vi "Results_file_Plotter.vi"() -> ()   [LabVIEW 2015]
uses:
  Anemometry/Anemometry Sub Vis/Data_plotting_vis/Plot_Slice.ctl
  Anemometry/Anemometry Sub Vis/Data_plotting_vis/Plotter_Mode.ctl
  Anemometry/Anemometry Sub Vis/Data_plotting_vis/Data_File_Type.ctl
  Anemometry/Anemometry Sub Vis/File/Setup_Filetype.ctl
  Anemometry/Anemometry Sub Vis/Controls/Global_mode.ctl
  Anemometry/Anemometry Sub Vis/Data_plotting_vis/Results_plotter_Global.vi
  Instance           1 28Saved   Results_file_Plotter .vi
  Anemometry/Anemometry Sub Vis/Globals/Constants_global.vi
  Anemometry/Anemometry Sub Vis/Globals/Trav_pos_global.vi
  kernel32.dll
panel:
  out "Index when last displayed":i32
  out "Index when last plotted":i32
  out "Edit Raw DF?":bool
  in  "Tab Control":T1(tab)=enum."Save "
  in  "Template":path
  in  "Empty":bool
  in  "Result files to read":path[](array[path])
  in  "Add results file":bool
  in  "File Types to Read":T2
  in  "Dot Plot?":bool
  in  "Vector Plot?":bool
  in  "Ordinate Name":string
  out "2nd Add label":string
  out "First Add label":string
  in  "Additional X Values":dbl[](array[numeric]) format="%.2f"
  in  "Additional Y Values":dbl[](array[numeric]) format="%.2f"
  in  "Show Results Space Analysis":bool
  in  "Show Plot Space Analysis":bool
  in  "Multi Ordinate":i32[](listbox)
  in  "Multi Ordinate?":bool
  in  "Ordinate":u16(ring) items=["File", "Date", "Time", "Comments", "Chilled Water Temp", "Inlet_Temp Average", "Av Floor Temp", "Max deltaT", "X (mm)", "Y (mm)", "Z (mm)", "Z (m)", "U/Uref", "u^2/Uref^2", "w^2/Uref^2", "-uw/Uref^2", "Inlet DeltaT", "DeltaT", "t^2", "ut", "wt", "Grad Ri", "Flux Ri", "B-V Freq N", "DeltaT/DeltaTmax", "W/Uref", "T thermistor", "dT/dZ", "dU/dZ", "Inlet Delta_Set", "u'/U", "w'/U", "W/U", "Location XY", "Location XZ", "U m/s", "W m/s", "u^2", "w^2", "Speed/Uref", "T cw", "Uref", "Flow Meas Time", "Profile", "t'/T", "t'", "uw", "Spires", "Roughness", "Z=1450 Inlet Temp", "Z=1350 Inlet Temp", "Z=1250 Inlet Temp", "Z=1150 Inlet Temp", "Z=1050 Inlet Temp", "Z=950 Inlet Temp", "Z=850 Inlet Temp", "Z=750 Inlet Temp", "Z=650 Inlet Temp", "Z=550 Inlet Temp", "Z=450 Inlet Temp", "Z=350 Inlet Temp", "Z=250 Inlet Temp", "Z=150 Inlet Temp", "Z=50 Inlet Temp", "EnFlo Lab Hygrometry Dew Point temp", "EnFlo Lab Hygrometry Dew Point temp_PN", "Multi Run Start Time", "T cw Offset A", "T cw Grad B", "LDA (U) Standard Error in Variance", "LDA (U) Standard Error in Mean", "LDA (W) Standard Error in Mean", "LDA (W) Standard Error in Variance", "U/Uref Err", "u^2/Uref^2 Err", "W/Uref Err", "w^2/Uref^2 Err", "Inlet Temp", "Inlet Setpoint", "Inlet Temp Error", "Seconds since 1st Jan", "Uni Chilled Water Temp", "EnFlo_Tunnel Chilled Water Valve Dem Pos", "EnFlo_Tunnel Temp Floor_Up_Y=-1585", "EnFlo_Tunnel Temp Floor_Up_Y=-1250", "EnFlo_Tunnel Temp Floor_Up_Y=-920", "EnFlo_Tunnel Temp Floor_Up_Y=-585", "EnFlo_Tunnel Temp Floor_Up_Y=-250", "EnFlo_Tunnel Temp Floor_Up_Y=80", "EnFlo_Tunnel Temp Floor_Up_Y=415", "EnFlo_Tunnel Temp Floor_Up_Y=750", "EnFlo_Tunnel Temp Floor_Up_Y=1080", "EnFlo_Tunnel Temp Floor_Up_Y=1415", "Raw Data Filename", "Z=1450 Inlet Setpoint", "Z=1350 Inlet Setpoint", "Z=1250 Inlet Setpoint", "Z=1150 Inlet Setpoint", "Z=1050 Inlet Setpoint", "Z=950 Inlet Setpoint", "Z=850 Inlet Setpoint", "Z=750 Inlet Setpoint", "Z=650 Inlet Setpoint", "Z=550 Inlet Setpoint", "Z=450 Inlet Setpoint", "Z=350 Inlet Setpoint", "Z=250 Inlet Setpoint", "Z=150 Inlet Setpoint", "Z=50 Inlet Setpoint", "Freq Hz", "LDA (U) E(f)", "LDA (W) E(f)", "CW (T) f.E(f)", "LDA (U) f.E(f)", "LDA (W) f.E(f)", "Folder"]
  in  "Intensity Plot?":bool
  in  "Absisca":u16(ring) items=["File", "Date", "Time", "Comments", "Chilled Water Temp", "Inlet_Temp Average", "Av Floor Temp", "Max deltaT", "X (mm)", "Y (mm)", "Z (mm)", "Z (m)", "U/Uref", "u^2/Uref^2", "w^2/Uref^2", "-uw/Uref^2", "Inlet DeltaT", "DeltaT", "t^2", "ut", "wt", "Grad Ri", "Flux Ri", "B-V Freq N", "DeltaT/DeltaTmax", "W/Uref", "T thermistor", "dT/dZ", "dU/dZ", "Inlet Delta_Set", "u'/U", "w'/U", "W/U", "Location XY", "Location XZ", "U m/s", "W m/s", "u^2", "w^2", "Speed/Uref", "T cw", "Uref", "Flow Meas Time", "Profile", "t'/T", "t'", "uw", "Spires", "Roughness", "Z=1450 Inlet Temp", "Z=1350 Inlet Temp", "Z=1250 Inlet Temp", "Z=1150 Inlet Temp", "Z=1050 Inlet Temp", "Z=950 Inlet Temp", "Z=850 Inlet Temp", "Z=750 Inlet Temp", "Z=650 Inlet Temp", "Z=550 Inlet Temp", "Z=450 Inlet Temp", "Z=350 Inlet Temp", "Z=250 Inlet Temp", "Z=150 Inlet Temp", "Z=50 Inlet Temp", "EnFlo Lab Hygrometry Dew Point temp", "EnFlo Lab Hygrometry Dew Point temp_PN", "Multi Run Start Time", "T cw Offset A", "T cw Grad B", "LDA (U) Standard Error in Variance", "LDA (U) Standard Error in Mean", "LDA (W) Standard Error in Mean", "LDA (W) Standard Error in Variance", "U/Uref Err", "u^2/Uref^2 Err", "W/Uref Err", "w^2/Uref^2 Err", "Inlet Temp", "Inlet Setpoint", "Inlet Temp Error", "Seconds since 1st Jan", "Uni Chilled Water Temp", "EnFlo_Tunnel Chilled Water Valve Dem Pos", "EnFlo_Tunnel Temp Floor_Up_Y=-1585", "EnFlo_Tunnel Temp Floor_Up_Y=-1250", "EnFlo_Tunnel Temp Floor_Up_Y=-920", "EnFlo_Tunnel Temp Floor_Up_Y=-585", "EnFlo_Tunnel Temp Floor_Up_Y=-250", "EnFlo_Tunnel Temp Floor_Up_Y=80", "EnFlo_Tunnel Temp Floor_Up_Y=415", "EnFlo_Tunnel Temp Floor_Up_Y=750", "EnFlo_Tunnel Temp Floor_Up_Y=1080", "EnFlo_Tunnel Temp Floor_Up_Y=1415", "Raw Data Filename", "Z=1450 Inlet Setpoint", "Z=1350 Inlet Setpoint", "Z=1250 Inlet Setpoint", "Z=1150 Inlet Setpoint", "Z=1050 Inlet Setpoint", "Z=950 Inlet Setpoint", "Z=850 Inlet Setpoint", "Z=750 Inlet Setpoint", "Z=650 Inlet Setpoint", "Z=550 Inlet Setpoint", "Z=450 Inlet Setpoint", "Z=350 Inlet Setpoint", "Z=250 Inlet Setpoint", "Z=150 Inlet Setpoint", "Z=50 Inlet Setpoint", "Freq Hz", "LDA (U) E(f)", "LDA (W) E(f)", "CW (T) f.E(f)", "LDA (U) f.E(f)", "LDA (W) f.E(f)", "Folder"]
  in  "Job Directory":path
  in  "Save Averaged rows":bool
  in  "Save Surface Fit":bool
  in  "Output Filename":path
  in  "Save Data in Rows":bool
  in  "Save Plot data":bool
  in  "Header":string
  in  "Process Point":bool
  in  "Kill Point":bool
  out "Table":string[][](table)
  in  "Post Process Plotted Data":bool
  in  "...using routine":string
  in  "Calculate new metadata":bool
  in  "Add /Edit metadata":bool
  in  "Delete Plotted data from file":bool
  in  "Add Inlet Temperature offset":bool
  in  "Plot EnFlo Tunnel Display":bool
  in  "Save Setup":bool
  in  "Load Setup":bool
  in  "stop":bool
  out "Current":string="Graph Scales"
  in  "Single Series":i32[](listbox)=[0]
  in  "Edit Template File":bool
  in  "color and symbol":bool
  out "nRows":i32
  in  "Filter Bins 2":i32[](listbox)=[0]
  in  "Filter 6":u16(ring)
  in  "Filter 5":u16(ring)
  in  "Filter 4":u16(ring)
  in  "Filter 3":u16(ring) items=["Show All (135)", "Vertical Profile (135)", "NOT Vertical Profile (0)"]
  in  "Filter Array":u16[](array[ring])=[0, 0, 0, 0, 0, 0] items=["Don't Filter", "File", "Date", "Time", "Comments", "Chilled Water Temp", "Inlet_Temp Average", "Av Floor Temp", "Max deltaT", "X (mm)", "Y (mm)", "Z (mm)", "Z (m)", "U/Uref", "u^2/Uref^2", "w^2/Uref^2", "-uw/Uref^2", "Inlet DeltaT", "DeltaT", "t^2", "ut", "wt", "Grad Ri", "Flux Ri", "B-V Freq N", "DeltaT/DeltaTmax", "W/Uref", "T thermistor", "dT/dZ", "dU/dZ", "Inlet Delta_Set", "u'/U", "w'/U", "W/U", "Location XY", "Location XZ", "U m/s", "W m/s", "u^2", "w^2", "Speed/Uref", "T cw", "Uref", "Flow Meas Time", "Profile", "t'/T", "t'", "uw", "Spires", "Roughness", "Z=1450 Inlet Temp", "Z=1350 Inlet Temp", "Z=1250 Inlet Temp", "Z=1150 Inlet Temp", "Z=1050 Inlet Temp", "Z=950 Inlet Temp", "Z=850 Inlet Temp", "Z=750 Inlet Temp", "Z=650 Inlet Temp", "Z=550 Inlet Temp", "Z=450 Inlet Temp", "Z=350 Inlet Temp", "Z=250 Inlet Temp", "Z=150 Inlet Temp", "Z=50 Inlet Temp", "EnFlo Lab Hygrometry Dew Point temp", "EnFlo Lab Hygrometry Dew Point temp_PN", "Multi Run Start Time", "T cw Offset A", "T cw Grad B", "LDA (U) Standard Error in Variance", "LDA (U) Standard Error in Mean", "LDA (W) Standard Error in Mean", "LDA (W) Standard Error in Variance", "U/Uref Err", "u^2/Uref^2 Err", "W/Uref Err", "w^2/Uref^2 Err", "Inlet Temp", "Inlet Setpoint", "Inlet Temp Error", "Seconds since 1st Jan", "Uni Chilled Water Temp", "EnFlo_Tunnel Chilled Water Valve Dem Pos", "EnFlo_Tunnel Temp Floor_Up_Y=-1585", "EnFlo_Tunnel Temp Floor_Up_Y=-1250", "EnFlo_Tunnel Temp Floor_Up_Y=-920", "EnFlo_Tunnel Temp Floor_Up_Y=-585", "EnFlo_Tunnel Temp Floor_Up_Y=-250", "EnFlo_Tunnel Temp Floor_Up_Y=80", "EnFlo_Tunnel Temp Floor_Up_Y=415", "EnFlo_Tunnel Temp Floor_Up_Y=750", "EnFlo_Tunnel Temp Floor_Up_Y=1080", "EnFlo_Tunnel Temp Floor_Up_Y=1415", "Raw Data Filename", "Z=1450 Inlet Setpoint", "Z=1350 Inlet Setpoint", "Z=1250 Inlet Setpoint", "Z=1150 Inlet Setpoint", "Z=1050 Inlet Setpoint", "Z=950 Inlet Setpoint", "Z=850 Inlet Setpoint", "Z=750 Inlet Setpoint", "Z=650 Inlet Setpoint", "Z=550 Inlet Setpoint", "Z=450 Inlet Setpoint", "Z=350 Inlet Setpoint", "Z=250 Inlet Setpoint", "Z=150 Inlet Setpoint", "Z=50 Inlet Setpoint", "Freq Hz", "LDA (U) E(f)", "LDA (W) E(f)", "CW (T) f.E(f)", "LDA (U) f.E(f)", "LDA (W) f.E(f)", "Folder"]
  in  "Filter Bins 1":i32[](listbox)=[0]
  in  "Create picture Vi Name":string caption="Picture VI:"
  in  "Save Plot as jpg":bool
  in  "Reload Files":bool
  out "Selected Row":i32
  out "Selected Row?":bool
  out "Warning!":string
  out "XY Plot":cluster{dbl[], dbl[]}[](graph)
  out "Edit Raw Data Header Info":bool
  out "Raw DF in Orig Pos?":bool
  out "Intensity Graph":dbl[][](graph)
  in  "Bkgnd Value":dbl
  in  "Update":bool
  in  "Plot Resolution":bool
  in  "Point Size":i32(slide)=1 scale=0.0..10.0
  in  "No of Contours":i32=20
  in  "Slice mode":T3
  in  "Z Ch Name":u16(ring) items=["File", "Date", "Time", "Comments", "Chilled Water Temp", "Inlet_Temp Average", "Av Floor Temp", "Max deltaT", "X (mm)", "Y (mm)", "Z (mm)", "Z (m)", "U/Uref", "u^2/Uref^2", "w^2/Uref^2", "-uw/Uref^2", "Inlet DeltaT", "DeltaT", "t^2", "ut", "wt", "Grad Ri", "Flux Ri", "B-V Freq N", "DeltaT/DeltaTmax", "W/Uref", "T thermistor", "dT/dZ", "dU/dZ", "Inlet Delta_Set", "u'/U", "w'/U", "W/U", "Location XY", "Location XZ", "U m/s", "W m/s", "u^2", "w^2", "Speed/Uref", "T cw", "Uref", "Flow Meas Time", "Profile", "t'/T", "t'", "uw", "Spires", "Roughness", "Z=1450 Inlet Temp", "Z=1350 Inlet Temp", "Z=1250 Inlet Temp", "Z=1150 Inlet Temp", "Z=1050 Inlet Temp", "Z=950 Inlet Temp", "Z=850 Inlet Temp", "Z=750 Inlet Temp", "Z=650 Inlet Temp", "Z=550 Inlet Temp", "Z=450 Inlet Temp", "Z=350 Inlet Temp", "Z=250 Inlet Temp", "Z=150 Inlet Temp", "Z=50 Inlet Temp", "EnFlo Lab Hygrometry Dew Point temp", "EnFlo Lab Hygrometry Dew Point temp_PN", "Multi Run Start Time", "T cw Offset A", "T cw Grad B", "LDA (U) Standard Error in Variance", "LDA (U) Standard Error in Mean", "LDA (W) Standard Error in Mean", "LDA (W) Standard Error in Variance", "U/Uref Err", "u^2/Uref^2 Err", "W/Uref Err", "w^2/Uref^2 Err", "Inlet Temp", "Inlet Setpoint", "Inlet Temp Error", "Seconds since 1st Jan", "Uni Chilled Water Temp", "EnFlo_Tunnel Chilled Water Valve Dem Pos", "EnFlo_Tunnel Temp Floor_Up_Y=-1585", "EnFlo_Tunnel Temp Floor_Up_Y=-1250", "EnFlo_Tunnel Temp Floor_Up_Y=-920", "EnFlo_Tunnel Temp Floor_Up_Y=-585", "EnFlo_Tunnel Temp Floor_Up_Y=-250", "EnFlo_Tunnel Temp Floor_Up_Y=80", "EnFlo_Tunnel Temp Floor_Up_Y=415", "EnFlo_Tunnel Temp Floor_Up_Y=750", "EnFlo_Tunnel Temp Floor_Up_Y=1080", "EnFlo_Tunnel Temp Floor_Up_Y=1415", "Raw Data Filename", "Z=1450 Inlet Setpoint", "Z=1350 Inlet Setpoint", "Z=1250 Inlet Setpoint", "Z=1150 Inlet Setpoint", "Z=1050 Inlet Setpoint", "Z=950 Inlet Setpoint", "Z=850 Inlet Setpoint", "Z=750 Inlet Setpoint", "Z=650 Inlet Setpoint", "Z=550 Inlet Setpoint", "Z=450 Inlet Setpoint", "Z=350 Inlet Setpoint", "Z=250 Inlet Setpoint", "Z=150 Inlet Setpoint", "Z=50 Inlet Setpoint", "Freq Hz", "LDA (U) E(f)", "LDA (W) E(f)", "CW (T) f.E(f)", "LDA (U) f.E(f)", "LDA (W) f.E(f)", "Folder"]
  in  "Y Ch Name":u16(ring) items=["File", "Date", "Time", "Comments", "Chilled Water Temp", "Inlet_Temp Average", "Av Floor Temp", "Max deltaT", "X (mm)", "Y (mm)", "Z (mm)", "Z (m)", "U/Uref", "u^2/Uref^2", "w^2/Uref^2", "-uw/Uref^2", "Inlet DeltaT", "DeltaT", "t^2", "ut", "wt", "Grad Ri", "Flux Ri", "B-V Freq N", "DeltaT/DeltaTmax", "W/Uref", "T thermistor", "dT/dZ", "dU/dZ", "Inlet Delta_Set", "u'/U", "w'/U", "W/U", "Location XY", "Location XZ", "U m/s", "W m/s", "u^2", "w^2", "Speed/Uref", "T cw", "Uref", "Flow Meas Time", "Profile", "t'/T", "t'", "uw", "Spires", "Roughness", "Z=1450 Inlet Temp", "Z=1350 Inlet Temp", "Z=1250 Inlet Temp", "Z=1150 Inlet Temp", "Z=1050 Inlet Temp", "Z=950 Inlet Temp", "Z=850 Inlet Temp", "Z=750 Inlet Temp", "Z=650 Inlet Temp", "Z=550 Inlet Temp", "Z=450 Inlet Temp", "Z=350 Inlet Temp", "Z=250 Inlet Temp", "Z=150 Inlet Temp", "Z=50 Inlet Temp", "EnFlo Lab Hygrometry Dew Point temp", "EnFlo Lab Hygrometry Dew Point temp_PN", "Multi Run Start Time", "T cw Offset A", "T cw Grad B", "LDA (U) Standard Error in Variance", "LDA (U) Standard Error in Mean", "LDA (W) Standard Error in Mean", "LDA (W) Standard Error in Variance", "U/Uref Err", "u^2/Uref^2 Err", "W/Uref Err", "w^2/Uref^2 Err", "Inlet Temp", "Inlet Setpoint", "Inlet Temp Error", "Seconds since 1st Jan", "Uni Chilled Water Temp", "EnFlo_Tunnel Chilled Water Valve Dem Pos", "EnFlo_Tunnel Temp Floor_Up_Y=-1585", "EnFlo_Tunnel Temp Floor_Up_Y=-1250", "EnFlo_Tunnel Temp Floor_Up_Y=-920", "EnFlo_Tunnel Temp Floor_Up_Y=-585", "EnFlo_Tunnel Temp Floor_Up_Y=-250", "EnFlo_Tunnel Temp Floor_Up_Y=80", "EnFlo_Tunnel Temp Floor_Up_Y=415", "EnFlo_Tunnel Temp Floor_Up_Y=750", "EnFlo_Tunnel Temp Floor_Up_Y=1080", "EnFlo_Tunnel Temp Floor_Up_Y=1415", "Raw Data Filename", "Z=1450 Inlet Setpoint", "Z=1350 Inlet Setpoint", "Z=1250 Inlet Setpoint", "Z=1150 Inlet Setpoint", "Z=1050 Inlet Setpoint", "Z=950 Inlet Setpoint", "Z=850 Inlet Setpoint", "Z=750 Inlet Setpoint", "Z=650 Inlet Setpoint", "Z=550 Inlet Setpoint", "Z=450 Inlet Setpoint", "Z=350 Inlet Setpoint", "Z=250 Inlet Setpoint", "Z=150 Inlet Setpoint", "Z=50 Inlet Setpoint", "Freq Hz", "LDA (U) E(f)", "LDA (W) E(f)", "CW (T) f.E(f)", "LDA (U) f.E(f)", "LDA (W) f.E(f)", "Folder"]
  in  "X Ch Name":u16(ring) items=["File", "Date", "Time", "Comments", "Chilled Water Temp", "Inlet_Temp Average", "Av Floor Temp", "Max deltaT", "X (mm)", "Y (mm)", "Z (mm)", "Z (m)", "U/Uref", "u^2/Uref^2", "w^2/Uref^2", "-uw/Uref^2", "Inlet DeltaT", "DeltaT", "t^2", "ut", "wt", "Grad Ri", "Flux Ri", "B-V Freq N", "DeltaT/DeltaTmax", "W/Uref", "T thermistor", "dT/dZ", "dU/dZ", "Inlet Delta_Set", "u'/U", "w'/U", "W/U", "Location XY", "Location XZ", "U m/s", "W m/s", "u^2", "w^2", "Speed/Uref", "T cw", "Uref", "Flow Meas Time", "Profile", "t'/T", "t'", "uw", "Spires", "Roughness", "Z=1450 Inlet Temp", "Z=1350 Inlet Temp", "Z=1250 Inlet Temp", "Z=1150 Inlet Temp", "Z=1050 Inlet Temp", "Z=950 Inlet Temp", "Z=850 Inlet Temp", "Z=750 Inlet Temp", "Z=650 Inlet Temp", "Z=550 Inlet Temp", "Z=450 Inlet Temp", "Z=350 Inlet Temp", "Z=250 Inlet Temp", "Z=150 Inlet Temp", "Z=50 Inlet Temp", "EnFlo Lab Hygrometry Dew Point temp", "EnFlo Lab Hygrometry Dew Point temp_PN", "Multi Run Start Time", "T cw Offset A", "T cw Grad B", "LDA (U) Standard Error in Variance", "LDA (U) Standard Error in Mean", "LDA (W) Standard Error in Mean", "LDA (W) Standard Error in Variance", "U/Uref Err", "u^2/Uref^2 Err", "W/Uref Err", "w^2/Uref^2 Err", "Inlet Temp", "Inlet Setpoint", "Inlet Temp Error", "Seconds since 1st Jan", "Uni Chilled Water Temp", "EnFlo_Tunnel Chilled Water Valve Dem Pos", "EnFlo_Tunnel Temp Floor_Up_Y=-1585", "EnFlo_Tunnel Temp Floor_Up_Y=-1250", "EnFlo_Tunnel Temp Floor_Up_Y=-920", "EnFlo_Tunnel Temp Floor_Up_Y=-585", "EnFlo_Tunnel Temp Floor_Up_Y=-250", "EnFlo_Tunnel Temp Floor_Up_Y=80", "EnFlo_Tunnel Temp Floor_Up_Y=415", "EnFlo_Tunnel Temp Floor_Up_Y=750", "EnFlo_Tunnel Temp Floor_Up_Y=1080", "EnFlo_Tunnel Temp Floor_Up_Y=1415", "Raw Data Filename", "Z=1450 Inlet Setpoint", "Z=1350 Inlet Setpoint", "Z=1250 Inlet Setpoint", "Z=1150 Inlet Setpoint", "Z=1050 Inlet Setpoint", "Z=950 Inlet Setpoint", "Z=850 Inlet Setpoint", "Z=750 Inlet Setpoint", "Z=650 Inlet Setpoint", "Z=550 Inlet Setpoint", "Z=450 Inlet Setpoint", "Z=350 Inlet Setpoint", "Z=250 Inlet Setpoint", "Z=150 Inlet Setpoint", "Z=50 Inlet Setpoint", "Freq Hz", "LDA (U) E(f)", "LDA (W) E(f)", "CW (T) f.E(f)", "LDA (U) f.E(f)", "LDA (W) f.E(f)", "Folder"]
  in  "Resolution":dbl=1.0 min=0.0 format="%.4f"
  out "Surface Area":dbl format="%^_6g"
  out "Surface Integral":dbl format="%^_6g"
  out "Surface Average":dbl format="%^#.6g"
  out "Uadvec":dbl
  in  "Full_Res_Results_Folder":path
  out "Last used Template":path
  out "Cursor index":i32
  out "Choosen Path":path
  in  "VI Refnum Calculation":refnum<vi>
  out "Filetype":string[](array[string])
  out "Mode":T4
  out "Plotted rows only?":bool
  in  "type specifier VI Refnum (for type only) 2":refnum<vi>
  in  "type specifier VI Refnum (for type only)":refnum<vi>
  out "Accept Array":bool[][](array[boolean])
  out "Previous slice mode":T3
  out "Slice mode Change?":bool
  out "Non-Blank Rows":bool[](array[boolean])
  out "File Index":i32
  out "Tolerances":dbl[](array[numeric]) format="%.2f"
  in  "Results files choosen":path[](array[path])
  in  "Transpose":bool
  out "Plotted Series":bool[][](array[boolean])
  in  "Results file":path
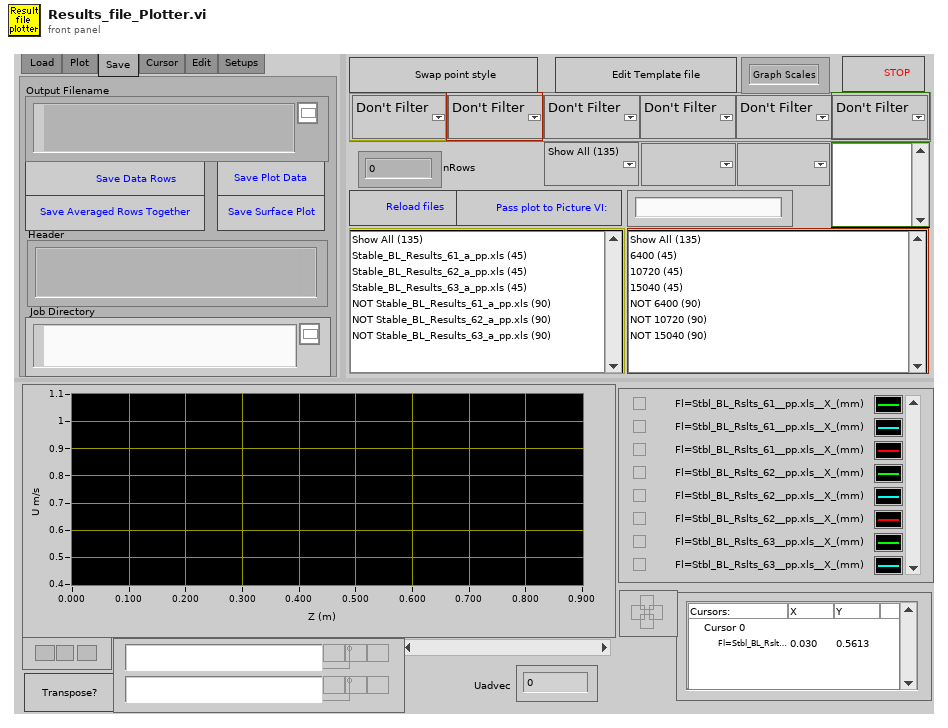
[diagram p1: front panel]
types:
  T1 = enum32{"Load ", "Plot ", "Save ", "Cursor", "Edit", "Setups"}
  T2 = typedef "Data_File_Type.ctl" = enum16{"Read All File Types", "Results Files Only", "Raw Data Files Only", "Calibration Files Only", "Gas Desk Files Only", "Old Results Files Only", "Tabulated Data Files Only"}
  T3 = typedef "Plot_Slice.ctl" = enum16{"XY Slice (Plan)", "YX Slice (Plan)", "YZ Slice (Cross)", "ZY Slice (Cross)", "XZ Slice (Side)", "ZX Slice (Side)"}
  T4 = typedef "Plotter_Mode.ctl" = enum16{"Save file", "Delete unwanted rows", "Edit Values with constants", "Edit values per row", "Edit Raw Data file header", "Post Process Plotted Rows", "Plot EnFlo Tunnel Display", "Add Inlet Temperature Offset"}
  T5 = typedef "Setup_Filetype.ctl" = enum16{"Measurement Setups", "Calibration Setups", "General", "Results File Plotter Setups", "Speed Calib Tweaks"}
  T6 = enum16{"Zero or one", "One", "Zero or more", "One or more"}
  T7 = typedef "Global_mode.ctl" = enum16{"Read Global", "Load Global From File", "Write Global to File"}
  T8 = enum16{"Edit Existing Template File", "Create New Template File"}
  T9 = enum16{"Show only data summary", "Show data summary", "No data summary"}
  T10 = typedef "All_Setup.ctl" = cluster{"Result files to read":path[], "Template":path, "Transpose":bool, "Additional X Values":dbl[], "Additional Y Values":dbl[], "Ordinate":u16, "Absisca":u16, "Filter Array":u16[], "color and symbol":bool, "Output Filename":path, "Jpg Vi Name":string, "Intensity Plot?":bool, "Multi Ordinate?":bool, "Filter Bins 1":i32[], "Filter Bins 2":i32[], "Multi Ordinate":i32[]}
  T11 = enum16{"Left Button", "Center Button", "Right Button", "Window Close"}
  T12 = enum32{"existing file", "new file", "new or existing file", "existing dir", "new dir", "new or existing dir", "existing file (use LLBs)", "new file (use LLBs)", "new or existing file (use LLBs)", "new or existing file or directory (use LLBs)"}
  T13 = cluster{"Plot Color":u32, "Plot Interpolation":u8, "Point Style":u8, "Line Style":u8, "Fill/Pt. Color":u32, "Line Width":u8, "Bar Plot Style":u8, "Fill To":i16}[]
  T14 = cluster{"X Max":dbl, "Y Max ":dbl, "X Scale":cluster{"Xo":dbl, "delta X":dbl}, "Y Scale":cluster{"Xo":dbl, "delta X":dbl}, "X Values":dbl[], "Y Values":dbl[], "Z Max":dbl, "Z Min":dbl}
  T15 = typedef "Group_Binning.ctl" = cluster{"Index":i32, "Tolerance":dbl, "Precision":string}
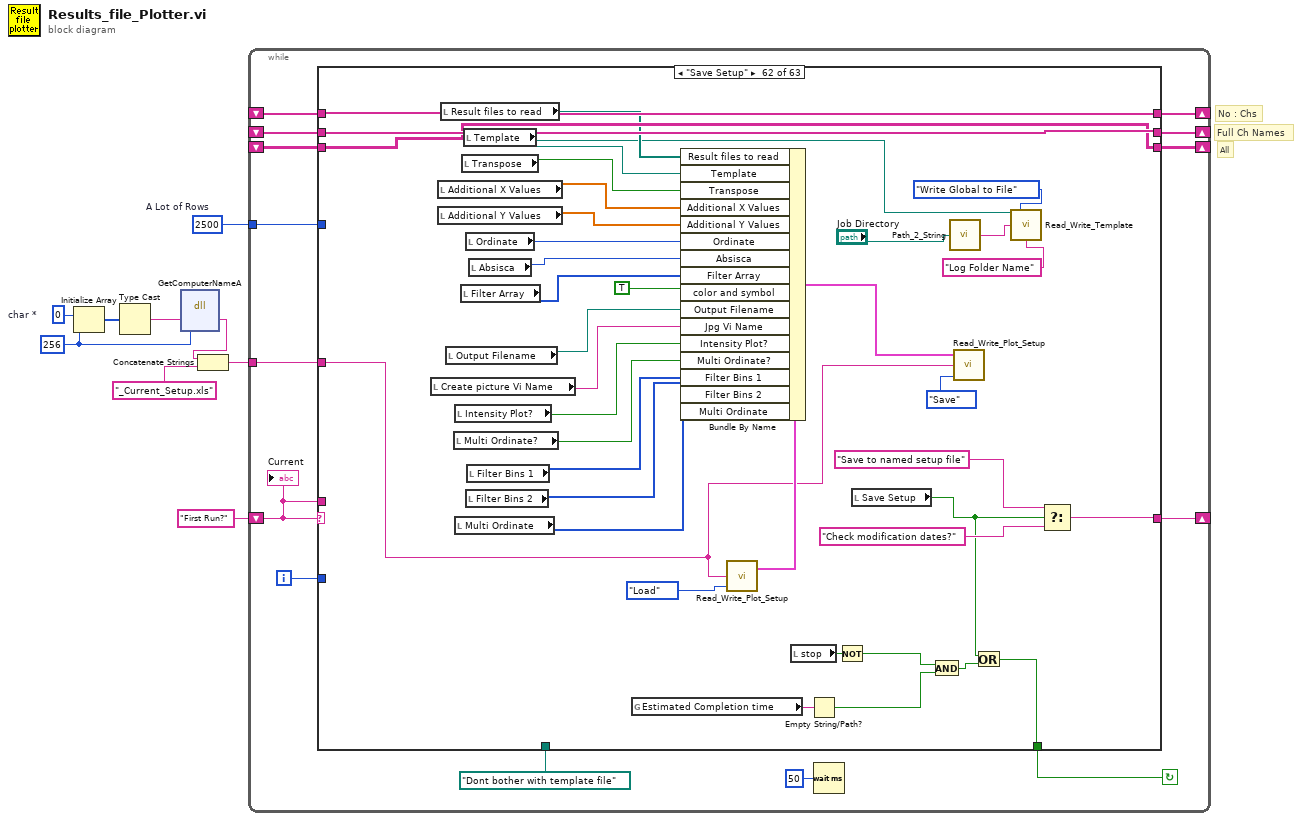
[diagram p0: block diagram]
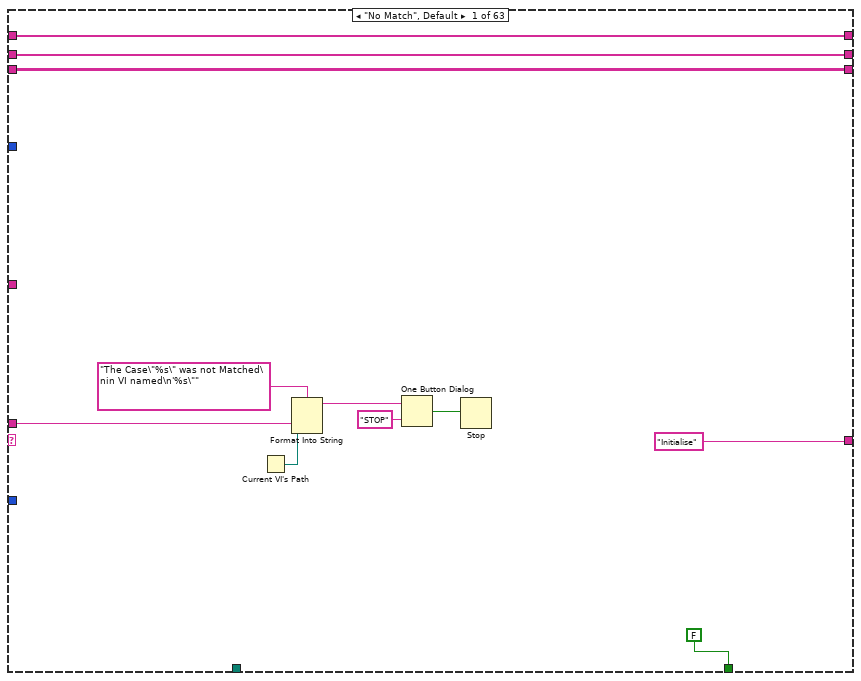
[diagram p2: hidden frame]
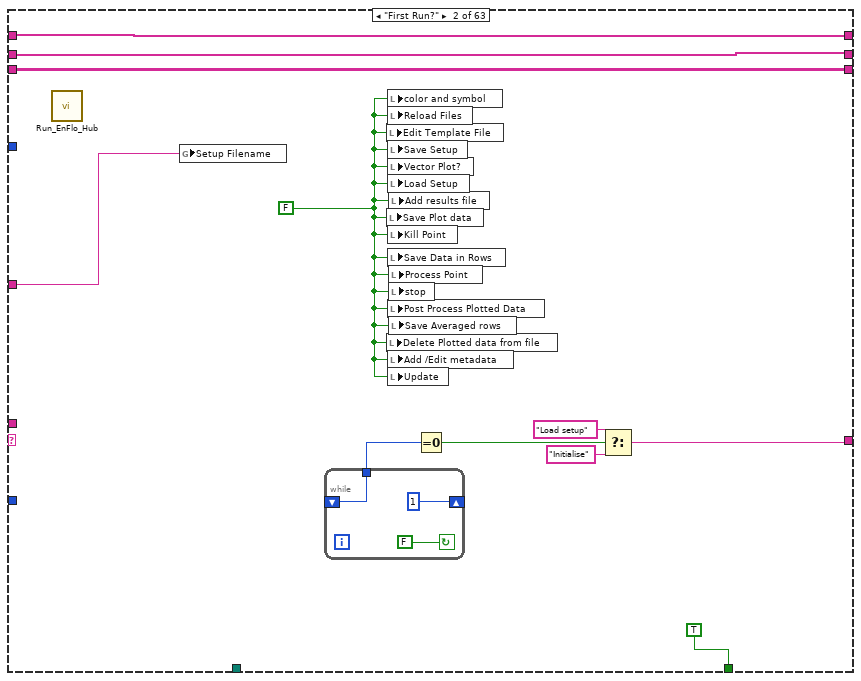
[diagram p3: hidden frame]
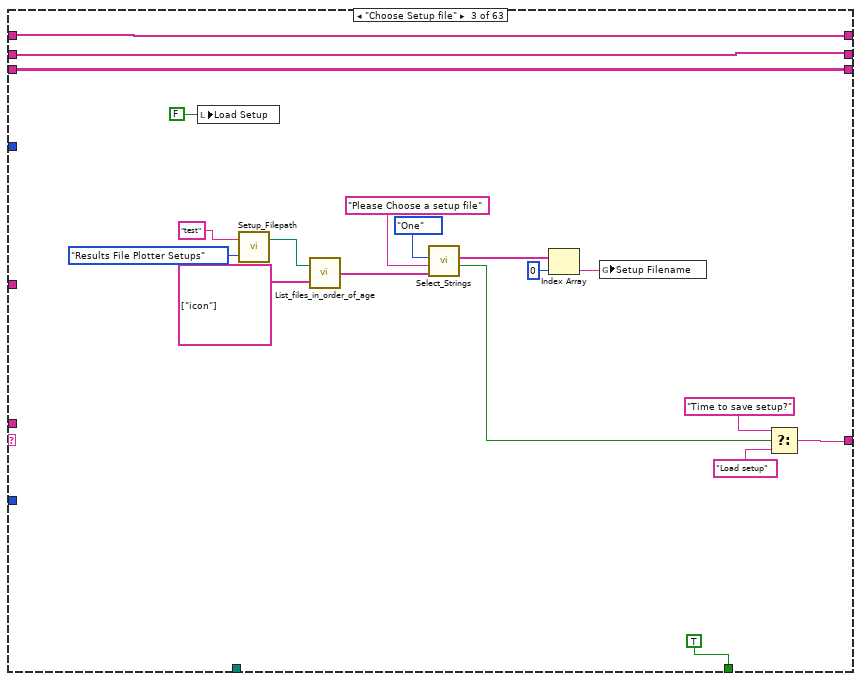
[diagram p4: hidden frame]
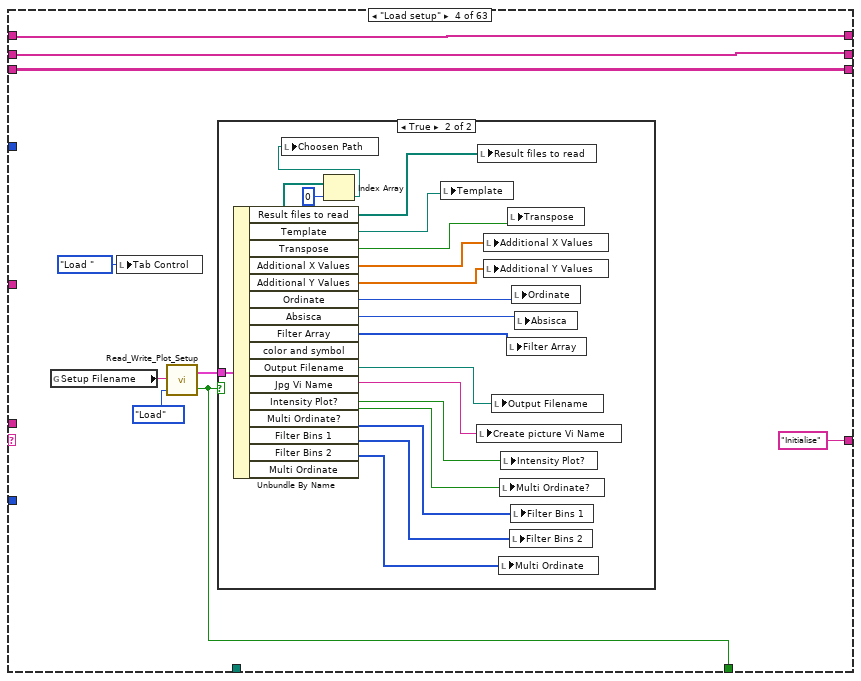
[diagram p5: hidden frame]
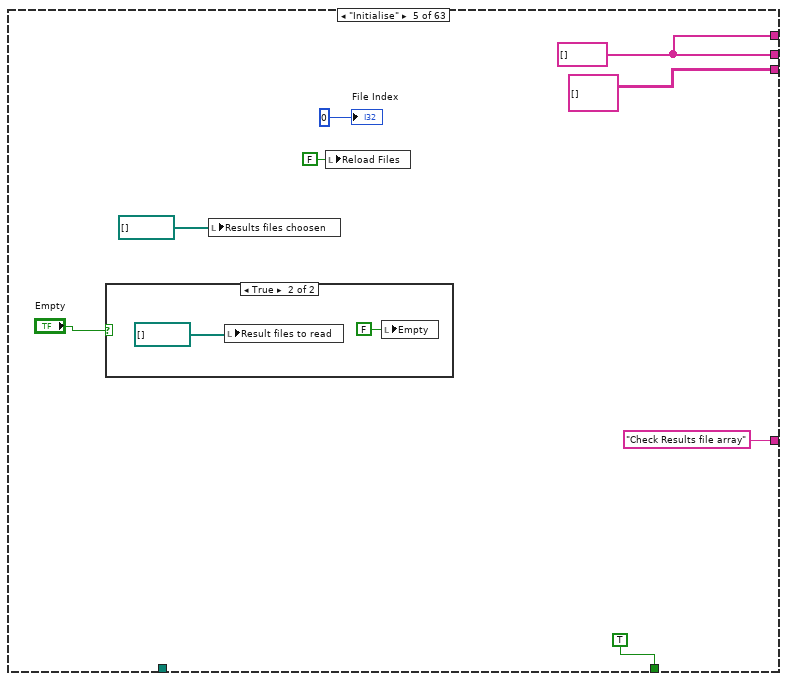
[diagram p7: hidden frame]
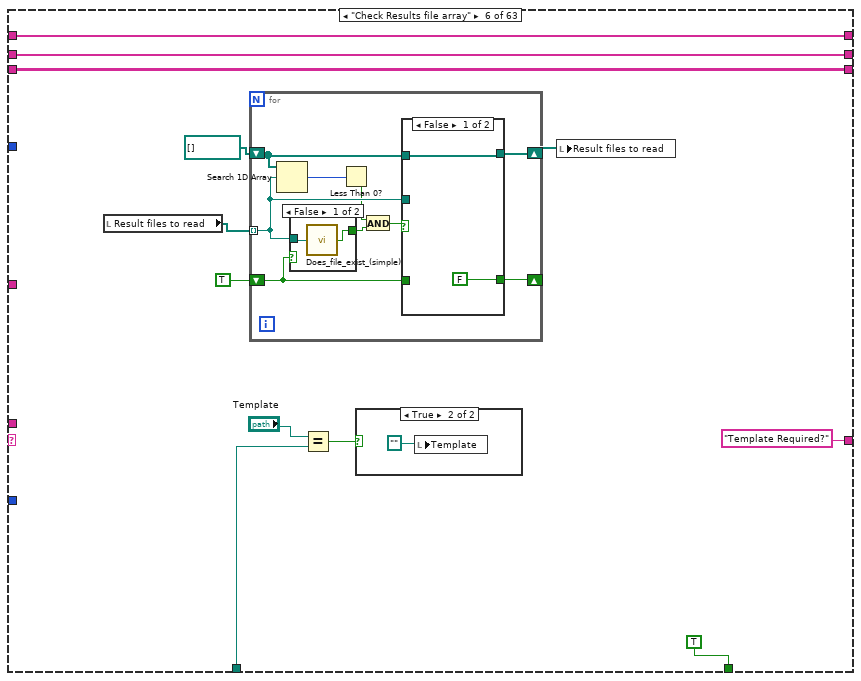
[diagram p9: hidden frame]
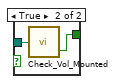
[diagram p11: hidden frame]
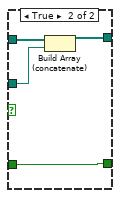
[diagram p12: hidden frame]
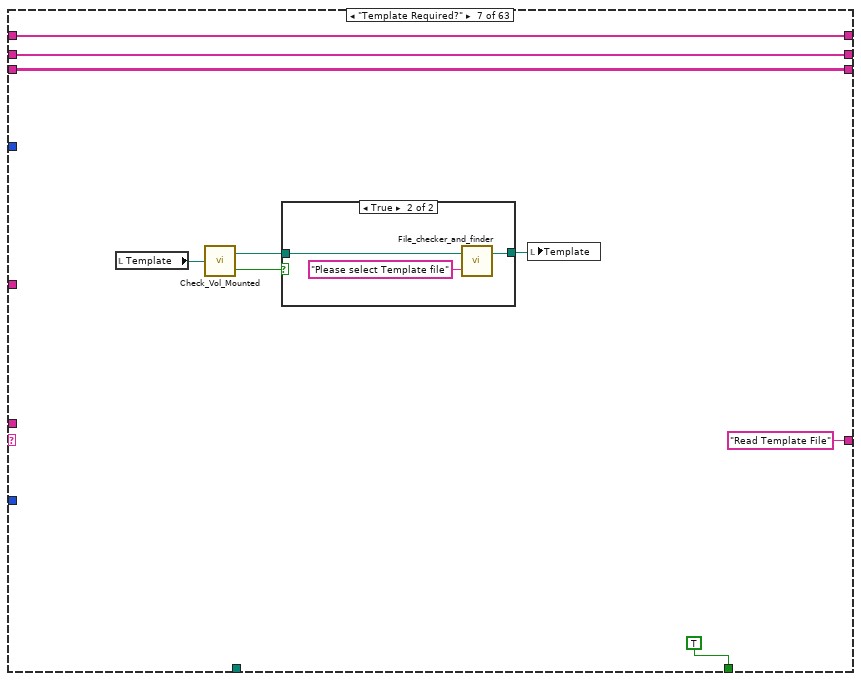
[diagram p13: hidden frame]
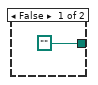
[diagram p14: hidden frame]
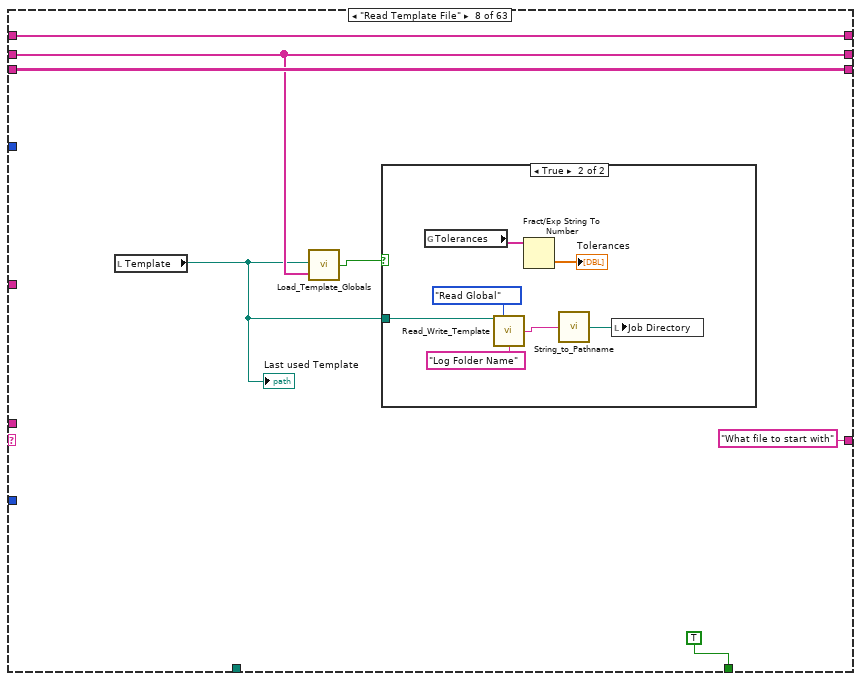
[diagram p15: hidden frame]
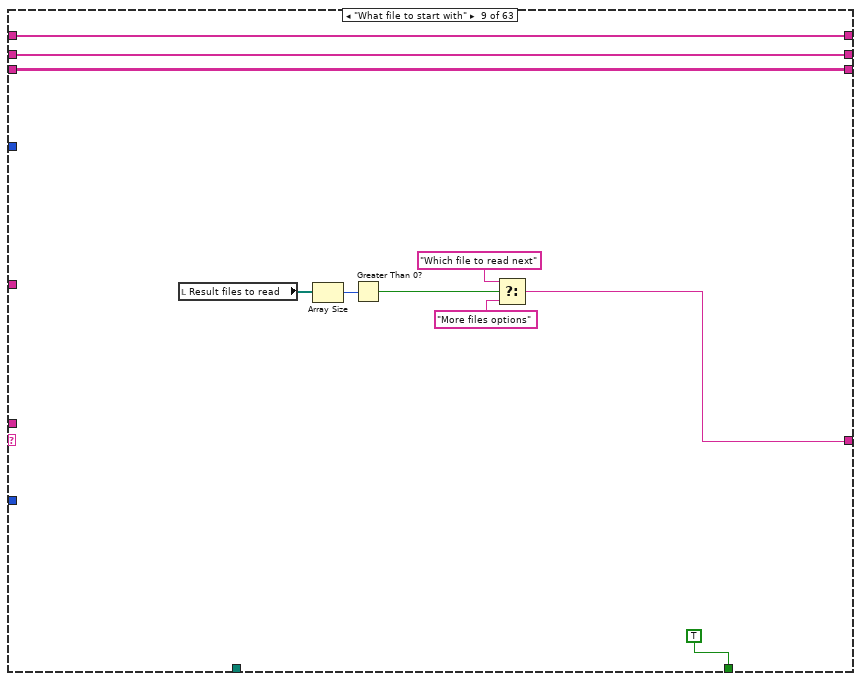
[diagram p17: hidden frame]
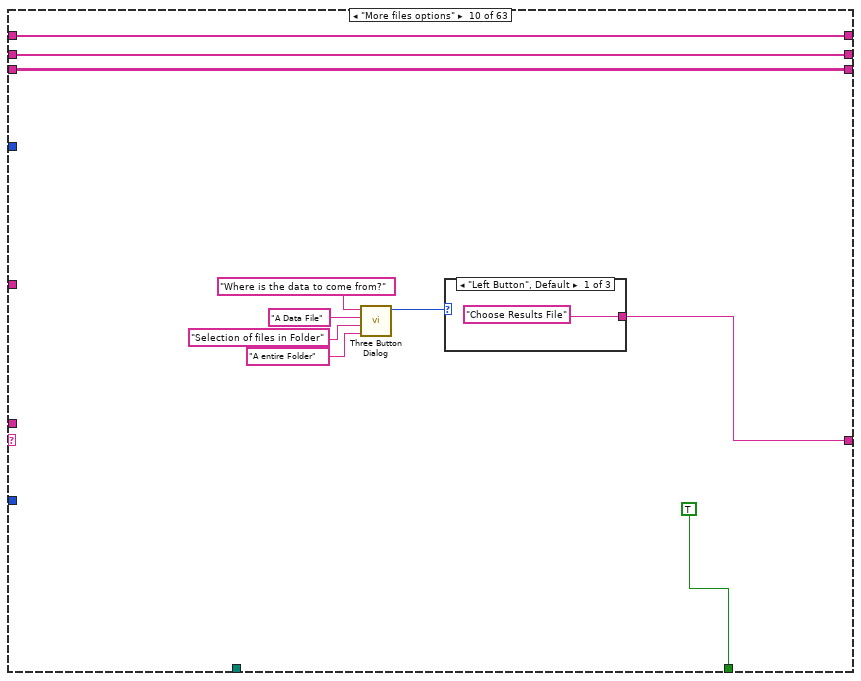
[diagram p18: hidden frame]
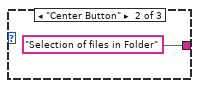
[diagram p19: hidden frame]
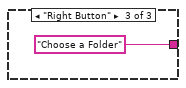
[diagram p20: hidden frame]
diagram:
  w7 = 256 ("dimension size")
  w4 = u8 0  # char *
  w8 = 2500  # A Lot of Rows
  # "No : Chs"
  # "Full Ch Names"
  # "All"
  n1 = Initialize Array(w4, w7) -> (w5:u8[])
  n2 = Type Cast(x=w5) -> (*(type *) &x=w6:string)  [unwired: 1 in]
  n3 = dll-call lib="kernel32.dll" fn="GetComputerNameA" label="unsigned long GetComputerNameA(CStr lpBuffer, long *nSize);"("lpBuffer"=w6, "nSize"=w7) -> ("lpBuffer"=w2:string)  [unwired: 5 in, 2 out]
  n4 = Concatenate Strings(w2, "_Current_Setup.xls" ("Setup filename")) -> (w1:string)
  n5 = while {
    shift-left: _ -> [w16]
    shift-right: [w17] -> _
    shift-left: "First Run?" -> [w20]
    shift-right: [w13] -> _
    shift-left: _ -> [w18]
    shift-right: [w23] -> _
    shift-left: _ -> [w21]
    shift-right: [w14] -> _
    tunnel: w8 -> [w12]
    tunnel: w1 -> [w10]
    i -> [w15]
    stop <- w22 continue-if-true
    n6 = case shown="\"Save Setup\"" w20 {
      tunnel: w18 -> [w34 w44 w66 w74 _ w115 w143 w152 w173 w183 w195 w209 w240 w267 w290 w412 w434 w460 w485 w511 w565 w579 w616 w926 w997 w1052 w1077 w1097 w1185 w1239 w1269 w1569 w1585 w1597 w1629 w1659 w1731 w1769 w1779 w1848 w1871 w1886 w1950 w2004 w2030 w2239 w2251 w2279 w2423 w2567 w2601 w2616 w2641 w2668 w2711 w2729 w2772 w2875 w2909 w3318 w3333 w3373 w3381]
      tunnel: [w34 w44 w66 w74 w100 w115 w143 w152 w173 w183 w195 w209 w240 w267 w288 w412 w434 w460 w485 w511 w565 w579 w616 w926 w997 w1052 w1077 w1097 w1185 w1239 w1267 w1569 w1585 w1597 w1629 w1659 w1731 w1769 w1779 w1848 w1871 w1886 w1950 w2004 w2028 w2239 w2251 w2277 w2416 w2567 w2601 w2616 w2641 w2668 w2711 w2729 w2772 w2875 w2909 w3318 w3333 w3373 w3381] -> w23
      tunnel: ["Initialise" w37 w61 "Initialise" ("t") "Check Results file array" ("t") "Template Required?" "Read Template File" "What file to start with" w164 w179 "Which file to read next" "Which file to read next" "Which file to read next" w263 w285 w403 "What is present?" "Ordinate Selector Type" w482 "Which rows are Non-Blank?" w558 "Create Selectors" w605 "Re Plot Data?" w993 "Prepare Filter2 strings" "Plot Data" w1094 "Add Axis names" "Analyse Plot Space" w1270 "What to do next?" "What to do next?" ("t") "What to do next?" ("t") w1611 w1652 w1707 w1765 w1777 w1843 w1867 w1885 w1949 "Initialise" w2031 w2230 "Create Selectors" w2280 w2424 w2565 w2599 w2606 w2625 "Save XY plot as jpg" "Create Selectors" w2726 w2775 w2859 w2914 "Save Setup" ("t") "Initialise" ("t") w3347 "Time to save setup?"] -> w13
      tunnel: [FALSE TRUE TRUE w70 TRUE TRUE TRUE TRUE TRUE TRUE TRUE TRUE TRUE w258 w292 TRUE TRUE TRUE TRUE TRUE TRUE TRUE TRUE TRUE TRUE TRUE TRUE w1095 TRUE TRUE w1271 TRUE TRUE ("OK?") TRUE ("OK?") TRUE TRUE ("OK?") TRUE ("OK?") TRUE ("OK?") TRUE ("OK?") TRUE TRUE w1884 w1948 TRUE w2032 TRUE ("OK?") TRUE ("OK?") w2281 w2425 TRUE TRUE TRUE TRUE TRUE TRUE TRUE TRUE TRUE TRUE TRUE TRUE w3340 TRUE ("OK?")] -> w22
      tunnel: w21 -> [w33 w43 w65 w73 _ w114 w142 w154 w172 w182 w194 w208 w239 w266 w291 w408 w433 w461 w486 w512 w564 w577 w611 w928 w987 w1054 w1079 w1096 w1187 w1241 w1268 w1568 w1584 w1596 w1628 w1670 w1730 w1768 w1778 w1847 w1870 w1883 w1947 w2003 w2029 w2238 w2248 w2278 w2422 w2568 w2600 w2615 w2645 w2671 w2710 w2728 w2771 w2874 w2908 w3317 w3332 w3372 w3380]
      tunnel: w20 -> [w25 _ _ _ _ _ _ _ _ _ _ _ _ _ _ _ _ _ _ _ _ _ _ _ _ _ _ _ _ _ _ _ _ _ _ _ _ _ _ _ _ _ _ _ _ _ _ _ _ _ _ _ _ _ _ _ _ _ _ _ _ _ _]
      tunnel: path "Dont bother with template file" ("Template File") -> [_ _ _ _ _ w108 _ _ _ _ _ _ _ _ _ _ _ _ _ _ _ _ _ _ _ _ _ _ _ _ _ _ _ _ _ _ _ _ _ _ _ _ _ _ _ _ _ _ _ _ _ _ _ _ _ _ _ _ _ w3315 w3327 _ _]
      tunnel: [w24 w42 w64 w75 w100 w113 w141 w153 w170 w180 w192 w206 w237 w265 w287 w396 w432 w462 w484 w510 w556 w578 w609 w925 w989 w1045 w1072 w1093 w1179 w1234 w1263 w1565 w1586 w1598 w1627 w1660 w1732 w1770 w1780 w1846 w1869 w1882 w1946 w2002 w2022 w2240 w2256 w2268 w2419 w2577 w2602 w2617 w2642 w2669 w2712 w2730 w2776 w2876 w2915 w3319 w3334 w3374 w3382] -> w17
      tunnel: w16 -> [w24 w42 w64 w75 _ w113 w141 w153 w170 w180 w192 w206 w237 w265 w286 w396 w432 w462 w484 w510 w556 w578 w609 w925 w989 w1045 w1072 w1093 w1179 w1234 w1262 w1565 w1586 w1598 w1627 w1660 w1732 w1770 w1780 w1846 w1869 w1882 w1946 w2002 w2021 w2240 w2256 w2272 w2418 w2577 w2602 w2617 w2642 w2669 w2712 w2730 w2776 w2876 w2915 w3319 w3334 w3374 w3382]
      tunnel: w15 -> [_ _ _ _ _ _ _ _ _ _ _ _ _ _ _ _ _ _ _ _ _ _ _ _ _ _ _ w1092 _ _ _ _ _ _ _ _ _ _ w1776 _ _ _ _ _ _ _ _ _ _ _ _ _ _ _ _ _ _ _ _ _ _ _ _]
      tunnel: [w33 w43 w65 w73 string[][] [] w114 w142 w154 w172 w182 w194 w208 w239 w266 w289 w408 w433 w461 w486 w512 w564 w577 w611 w928 w987 w1054 w1079 w1096 w1187 w1241 w1266 w1568 w1584 w1596 w1628 w1670 w1730 w1768 w1778 w1847 w1870 w1883 w1947 w2003 w2027 w2238 w2248 w2276 w2415 w2568 w2600 w2615 w2645 w2671 w2710 w2728 w2771 w2874 w2908 w3317 w3332 w3372 w3380] -> w14
      tunnel: w12 -> [_ _ _ _ _ _ _ _ _ _ _ _ _ _ _ _ _ _ _ _ _ _ _ _ _ _ _ _ _ _ _ _ _ _ _ _ _ _ _ _ w1865 _ w1945 _ _ _ _ _ _ _ _ _ _ _ _ w2725 w2769 _ w2906 _ _ _ _]
      tunnel: w10 -> [_ w35 _ _ _ _ _ _ _ _ _ _ _ _ _ _ _ _ _ _ _ _ _ _ _ _ _ _ _ _ _ _ _ _ _ _ _ _ _ _ _ _ _ _ _ _ _ _ _ _ _ _ _ _ _ _ _ _ _ _ _ w3339 _]
      frame "No Match", Default {
        n7 = Current VI's Path() -> (path=w26:path)
        n8 = Format Into String(format string="The Case\"%s\" was not Matched\nin VI named\n'%s\"" ("Format String"), w25, w26) -> (resulting string=w29:string)  [unwired: 2 in, 1 out]
        n9 = One Button Dialog(message=w29, button name ("OK")="STOP") -> (true=w27:bool)
        n10 = Stop(stop? (T)=w27) -> ()
      }
      frame "First Run?" {
        w36 = FALSE ("Save Plot data")
        n11 = call "Run_EnFlo_Hub.vi"() -> ()  [unwired: 8 out]
        n12 = global write "Results_plotter_Global.vi" "Setup Filename"(w35) -> ()
        n13 = while {
          shift-right: [1] -> _
          shift-left: _ -> [w47]
          tunnel: [w47] -> w39
          stop <- FALSE continue-if-true
        }
        n14 = local write "Edit Template File"(w36) -> ()
        n15 = local write "Save Plot data"(w36) -> ()
        n16 = local write "Delete Plotted data from file"(w36) -> ()
        n17 = local write "color and symbol"(w36) -> ()
        n18 = local write "Reload Files"(w36) -> ()
        n19 = local write "Save Setup"(w36) -> ()
        n20 = local write "Vector Plot?"(w36) -> ()
        n21 = local write "Load Setup"(w36) -> ()
        n22 = local write "Kill Point"(w36) -> ()
        n23 = local write "Save Data in Rows"(w36) -> ()
        n24 = local write "Post Process Plotted Data"(w36) -> ()
        n25 = local write "Add /Edit metadata"(w36) -> ()
        n26 = local write "Update"(w36) -> ()
        n27 = local write "Add results file"(w36) -> ()
        n28 = local write "Process Point"(w36) -> ()
        n29 = local write "stop"(w36) -> ()
        n30 = local write "Save Averaged rows"(w36) -> ()
        n31 = Equal To 0?(x=w39) -> (x = 0?=w38:bool)
        n32 = Select(t="Load setup", s=w38, f="Initialise") -> (s? t:f=w37:string)
      }
      frame "Choose Setup file" {
        n33 = local write "Load Setup"(FALSE ("Save Setup")) -> ()
        n34 = call "Setup_Filepath.vi"("Setup File Type"=Setup_Filetype."Results File Plotter Setups", "Filename in"="test") -> ("Directory"=w49:path)  [unwired: 1 out]
        n35 = call "List_files_in_order_of_age.vi"("Files to Hide"=string[] ["icon"], "Folder"=w49) -> ("file names"=w60:string[])
        n36 = call "Select_Strings.vi"("Available Ch names"=w60, "Message"="Please Choose a setup file", "Selector mode"=T6."One") -> ("Cancel"=w54:bool, "Selected Channel Names"=w57:string[])  [unwired: 1 in, 3 out]
        n37 = Index Array(array=w57, index=0) -> (element=w55:string)
        n38 = global write "Results_plotter_Global.vi" "Setup Filename"(w55) -> ()
        n39 = Select(t="Time to save setup?", s=w54, f="Load setup") -> (s? t:f=w61:string)
      }
      frame "Load setup" {
        n40 = global read "Results_plotter_Global.vi" "Setup Filename"() -> (w69:string)
        n41 = local write "Tab Control"(T1."Load " ("Tab Control")) -> ()
        n42 = call "Read_Write_Plot_Setup.vi"("Mode"=enum16{"Load", "Save"}."Load", "Setup filename"=w69) -> ("OK?"=w70:bool, "Cluster 2"=w71:T10)  [unwired: 1 in]
        n43 = case shown="True" w70 {
          tunnel: w71 -> [_ w94]
          frame False {
          }
          frame True {
            n44 = Unbundle By Name(w94) -> ("Result files to read"=w79:path[], "Template"=w77:path, "Transpose"=w84:bool, "Additional X Values"=w85:dbl[], "Additional Y Values"=w86:dbl[], "Ordinate"=w87:u16, "Absisca"=w88:u16, "Filter Array"=w89:u16[], "Output Filename"=w90:path, "Jpg Vi Name"=w91:string, "Intensity Plot?"=w92:bool, "Multi Ordinate?"=w93:bool, "Filter Bins 1"=w83:i32[], "Filter Bins 2"=w82:i32[], "Multi Ordinate"=w81:i32[])  [unwired: 1 out]
            n45 = Index Array(array=w79, index=0) -> (element=w78:path)
            n46 = local write "Choosen Path"(w78) -> ()
            n47 = local write "Template"(w77) -> ()
            n48 = local write "Create picture Vi Name"(w91) -> ()
            n49 = local write "Result files to read"(w79) -> ()
            n50 = local write "Additional X Values"(w85) -> ()
            n51 = local write "Additional Y Values"(w86) -> ()
            n52 = local write "Output Filename"(w90) -> ()
            n53 = local write "Multi Ordinate"(w81) -> ()
            n54 = local write "Multi Ordinate?"(w93) -> ()
            n55 = local write "Intensity Plot?"(w92) -> ()
            n56 = local write "Filter Array"(w89) -> ()
            n57 = local write "Transpose"(w84) -> ()
            n58 = local write "Filter Bins 2"(w82) -> ()
            n59 = local write "Filter Bins 1"(w83) -> ()
            n60 = local write "Ordinate"(w87) -> ()
            n61 = local write "Absisca"(w88) -> ()
          }
        }
      }
      frame "Initialise" {
        w100 = string[] [] ("Channel names")
        n62 = case shown="True" "Empty" {
          frame False {
          }
          frame True {
            n63 = local write "Result files to read"(path[] [] ("Result files to read")) -> ()
            n64 = local write "Empty"(FALSE ("Empty")) -> ()
          }
        }
        n65 = local write "Results files choosen"(path[] [] ("Results file choosen")) -> ()
        n66 = local write "Reload Files"(FALSE ("Reload Files")) -> ()
        "File Index" <- 0
      }
      frame "Check Results file array" {
        n67 = local read "Result files to read"() -> (w112:path[])
        n68 = for {
          shift-right: [w126] -> w110
          shift-left: path[] [] -> [w125]
          tunnel: w112 -> [w124] mode=indexing
          shift-right: [w119] -> _
          shift-left: TRUE -> [w118]
          n69 = Search 1D Array(1D array=w125, element=w124) -> (index of element=w123:i32)  [unwired: 1 out]
          n70 = case shown="False" w118 {
            tunnel: w124 -> [w128 w130]
            tunnel: [w127 w129] -> w121
            frame False {
              n71 = call "Does_file_exist_(simple).vi"("Pathname"=w128) -> ("exists?"=w127:bool)
            }
            frame True {
              n72 = call "Check_Vol_Mounted.vi"("Filename"=w130) -> ("exists?"=w129:bool)  [unwired: 1 out]
            }
          }
          n73 = Less Than 0?(x=w123) -> (x < 0?=w120:bool)
          n74 = And(x=w120, y=w121) -> (x .and. y?=w122:bool)
          n75 = case shown="False" w122 {
            tunnel: w125 -> [w132 w136]
            tunnel: w124 -> [_ w135]
            tunnel: [w132 w134] -> w126
            tunnel: [FALSE w133] -> w119
            tunnel: w118 -> [_ w133]
            frame False {
            }
            frame True {
              n76 = Build Array (concatenate)(w136, w135) -> (w134:path[])
            }
          }
        }
        n77 = Equal?(x="Template", y=w108) -> (x = y?=w107:bool)
        n78 = case shown="True" w107 {
          frame False {
          }
          frame True {
            n79 = local write "Template"(path "") -> ()
          }
        }
        n80 = local write "Result files to read"(w110) -> ()
      }
      frame "Template Required?" {
        n81 = local read "Template"() -> (w140:path)
        n82 = call "Check_Vol_Mounted.vi"("Filename"=w140) -> ("Filename Out"=w139:path, "exists?"=w138:bool)
        n83 = case shown="True" w138 {
          tunnel: w139 -> [_ w148]
          tunnel: [path "" w147] -> w137
          frame False {
          }
          frame True {
            n84 = call "File_checker_and_finder.vi"("Promp if not found"="Please select Template file", "Filename In"=w148) -> ("Filename Out"=w147:path)  [unwired: 1 out]
          }
        }
        n85 = local write "Template"(w137) -> ()
      }
      frame "Read Template File" {
        n86 = local read "Template"() -> (w150:path)
        "Last used Template" <- w150
        n87 = call "Load_Template_Globals.vi"("Channel Names"=w152, "Template-read"=w150) -> ("Valid Template File?"=w151:bool)
        n88 = case shown="True" w151 {
          tunnel: w150 -> [_ w159]
          frame False {
          }
          frame True {
            n89 = global read "Results_plotter_Global.vi" "Tolerances"() -> (w162:string[])
            n90 = call "Read_Write_Template.vi"("Template File"=w159, "Mode"=Global_mode."Read Global", "Data type"="Log Folder Name" ("Variable name")) -> ("Single Value Out"=w157:string)  [unwired: 5 in, 7 out]
            n91 = Fract/Exp String To Number(string=w162) -> (number=→"Tolerances":dbl[])  [unwired: 4 out]
            n92 = call "String_to_Pathname.vi"("Input String"=w157) -> ("path"=w158:path)
            n93 = local write "Job Directory"(w158) -> ()
          }
        }
      }
      frame "What file to start with" {
        n94 = local read "Result files to read"() -> (w169:path[])
        n95 = Array Size(array=w169) -> (size(s)=w168:i32)
        n96 = Greater Than 0?(x=w168) -> (x > 0?=w165:bool)
        n97 = Select(t="Which file to read next", s=w165, f="More files options") -> (s? t:f=w164:string)
      }
      frame "More files options" {
        n98 = call <vilib>:"Three Button Dialog.vi"("Right Button Text (\"Cancel\")"="A entire Folder" ("F button name (\"Cancel\")"), "Center Button Text (\"No\")"="Selection of files in Folder" ("T button name (\"OK\")"), "Left Button Text (\"Yes\")"="A Data File" ("T button name (\"OK\")"), "message"="Where is the data to come from?") -> ("Which Button?"=w178:T11)  [unwired: 1 in, 6 out]
        n99 = case shown="\"Left Button\", Default" w178 {
          tunnel: ["Choose Results File" "Selection of files in Folder" "Choose a Folder"] -> w179
          frame "Left Button", Default {
          }
          frame "Center Button" {
          }
          frame "Right Button" {
          }
        }
      }
      frame "Choose Results File" {
        (unwired) T12."existing file" ("select mode (2)")
        n100 = local read "Choosen Path"() -> (w187:path)
        n101 = File Dialog(7:"Please Choose a Results File" ("Promp if not found"), 11:w187) -> (1:w189:bool, 3:w188:path)  [unwired: 1 in, 6 out]
        "Choosen Path" <- w188
        n102 = case shown="False" w189 {
          tunnel: w188 -> [w196 _]
          frame False {
            n103 = local read "Result files to read"() -> (w197:path[])
            n104 = Build Array (concatenate)(w197, w196) -> (w198:path[])
            n105 = local write "Result files to read"(w198) -> ()
          }
          frame True {
          }
        }
      }
      frame "Choose a Folder" {
        n106 = local read "Choosen Path"() -> (w200:path)
        n107 = File Dialog(7:"Please Choose the folder that contains the Results files to be plotted" ("prompt"), 11:w200) -> (3:w199:path)  [unwired: 1 in, 7 out]
        n108 = local write "Choosen Path"(w199) -> ()
        n109 = call "Get_folder_and_filenames.vi"("file path (dialog if empty)"=w199) -> ("Files"=w201:path[])  [unwired: 1 out]
        n110 = for {
          shift-right: [w220] -> w202
          shift-left: "Result files to read" -> [w219]
          tunnel: w201 -> [w217] mode=indexing
          n111 = Search 1D Array(1D array=w219, element=w217) -> (index of element=w218:i32)  [unwired: 1 out]
          n112 = Strip Path(path=w217) -> (name=w216:string)  [unwired: 1 out]
          n113 = Less Than 0?(x=w218) -> (x < 0?=w215:bool)
          n114 = call "Add_filename_suffix.vi"("Filename"=w216) -> ("Original Suffix"=w213:string)  [unwired: 1 in, 3 out]
          n115 = call "Match_Pat_Case_In.vi"("String to match"=".jpg" ("x"), "String"=w213) -> ("offset past match"=w211:i32)  [unwired: 1 in, 3 out]
          n116 = Less Than 0?(x=w211) -> (x < 0?=w210:bool)
          n117 = And(x=w215, y=w210) -> (x .and. y?=w214:bool)
          n118 = case shown="True" w214 {
            tunnel: w219 -> [w221 w224]
            tunnel: w217 -> [_ w223]
            tunnel: [w221 w222] -> w220
            frame False {
            }
            frame True {
              n119 = Build Array (concatenate)(w224, w223) -> (w222:path[])
            }
          }
        }
        n120 = local write "Result files to read"(w202) -> ()
      }
      frame "Selection of files in Folder" {
        n121 = local read "Choosen Path"() -> (w226:path)
        n122 = local read "Result files to read"() -> (w229:path[])
        n123 = File Dialog(7:"Please Choose the folder that contains the Results files to be plotted" ("prompt"), 11:w226) -> (3:w225:path)  [unwired: 1 in, 7 out]
        n124 = call "Get_folder_and_filenames.vi"("file path (dialog if empty)"=w225) -> ("Files"=w231:path[])  [unwired: 1 out]
        n125 = local write "Choosen Path"(w225) -> ()
        n126 = for {
          tunnel: w231 -> [w254] mode=indexing
          tunnel: [w253] -> w234 mode=indexing
          n127 = Strip Path(path=w254) -> (name=w253:string)  [unwired: 1 out]
        }
        n128 = call "Select_Strings.vi"("Available Ch names"=w234, "Message"="Please select the desired data files", "Selector mode"=T6."Zero or more") -> ("Ch Indicies Choosen"=w232:i32[])  [unwired: 1 in, 4 out]
        n129 = for {
          tunnel: w232 -> [w252] mode=indexing
          tunnel: w231 -> [w251]
          tunnel: [w250] -> w227 mode=indexing
          n130 = Index Array(array=w251, index=w252) -> (element=w250:path)
        }
        n131 = for {
          shift-right: [w245] -> w228
          shift-left: w229 -> [w244]
          tunnel: w227 -> [w243] mode=indexing
          n132 = Search 1D Array(1D array=w244, element=w243) -> (index of element=w242:i32)  [unwired: 1 out]
          n133 = Less Than 0?(x=w242) -> (x < 0?=w241:bool)
          n134 = case shown="True" w241 {
            tunnel: w244 -> [w246 w249]
            tunnel: w243 -> [_ w248]
            tunnel: [w246 w247] -> w245
            frame False {
            }
            frame True {
              n135 = Build Array (concatenate)(w249, w248) -> (w247:path[])
            }
          }
        }
        n136 = local write "Result files to read"(w228) -> ()
      }
      frame "Which file to read next" {
        n137 = local read "Result files to read"() -> (w264:path[])
        n138 = local read "File Index"() -> (w261:i32)
        n139 = Array Size(array=w264) -> (size(s)=w262:i32)
        n140 = Equal?(x=w262, y=w261) -> (x = y?=w260:bool)
        n141 = case shown="False" w260 {
          tunnel: w264 -> [w270 _]
          tunnel: [w271 "Load Selectors"] -> w263
          tunnel: w261 -> [w269 w283]
          tunnel: [w268 w283] -> w256
          frame False {
            n142 = Index Array(array=w270, index=w269) -> (element=w272:path)
            n143 = Search 1D Array(1D array="Results files choosen", element=w272) -> (index of element=w274:i32)  [unwired: 1 out]
            n144 = call "Add_filename_suffix.vi"() -> ()  [unwired: 2 in, 4 out]
            n145 = case shown="-1" w274 {
              tunnel: "Results files choosen" -> [_ w282]
              tunnel: w272 -> [w278 w281]
              tunnel: ["Which file to read next" "Load Data"] -> w271
              frame 0, Default {
                n146 = Format Into String(format string="The filename\n \"%s\"\n has already been chosen" ("Format String"), w278) -> (resulting string=w276:string)  [unwired: 2 in, 1 out]
                n147 = One Button Dialog(message=w276) -> ()  [unwired: 2 out]
              }
              frame -1 {
                n148 = Build Array (concatenate)(w282, w281) -> (w280:path[])
                n149 = local write "Results files choosen"(w280) -> ()
              }
            }
            n150 = local write "Results file"(w272) -> ()
            n151 = Increment(x=w269) -> (x+1=w268:i32)
          }
          frame True {
          }
        }
        n152 = local read "stop"() -> (w259:bool)
        n153 = Decrement(x=w256) -> (x-1=w255:i32)
        n154 = Build Array(w255) -> (w257:i32[])
        n155 = Not(x=w259) -> (.not. x?=w258:bool)
        n156 = local write "File Index"(w256) -> ()
        n157 = property on="Result files to read" class="Arr (strict)"("Index Values"=w257) -> ()  [unwired: 2 in, 2 out]
      }
      frame "Load Data" {
        n158 = stacked-sequence {
          seq-local: [w297 _] -> [_ w357]
          seq-local: [w296 _] -> [_ w362]
          seq-local: [w295 _] -> [_ w361]
          seq-local: [w293 _] -> [_ w360]
          tunnel: [TRUE _] -> w292
          tunnel: w291 -> [w311 w363]
          tunnel: w290 -> [w310 _]
          tunnel: [w309 _] -> w289
          tunnel: [w308 _] -> w288
          tunnel: [w307 _] -> w287
          tunnel: w286 -> [w306 _]
          tunnel: ["Which file to read next" _] -> w285
          frame #0 {
            w300 = TRUE  # Add Extra Channels?
            n159 = local read "Template"() -> (w304:path)
            n160 = call "Read_Data_file.vi"("Results file"="Results file", "Add Extra Channels?"=w300, "Template File"=w304, "Desired File Types"="File Types to Read") -> ("Row numbers"=w295:i32[], "Template File Out"=w301:path, "Filetype"=w296:string, "Results file Out"=w297:path, "Ch names Out"=w302:string[], "Channel Values Out"=w298:string[][])  [unwired: 1 in, 9 out]
            n161 = local write "Template"(w301) -> ()
            n162 = Array Size(array=w302) -> (size(s)=w303:i32)
            n163 = Greater Than 0?(x=w303) -> (x > 0?=w293:bool)
            n164 = case shown="True" w293 {
              tunnel: w311 -> [w313 w327]
              tunnel: w310 -> [w315 w322]
              tunnel: w298 -> [_ w320]
              tunnel: [w313 w318] -> w309
              tunnel: [w315 w316] -> w308
              tunnel: [w314 w317] -> w307
              tunnel: w306 -> [w314 _]
              tunnel: w302 -> [_ w321]
              frame False {
              }
              frame True {
                n165 = for {
                  tunnel: w320 -> [w329] mode=indexing
                  tunnel: [w328] -> w319 mode=indexing
                  n166 = for {
                    tunnel: w329 -> [w331] mode=indexing
                    tunnel: [w330] -> w328 mode=indexing
                    n167 = call "Fast_string_Replace.vi"("Replace match with:"="[", "Input String"=w331, "regular expression"="(") -> ("Output String"=w332:string)  [unwired: 2 out]
                    n168 = call "Fast_string_Replace.vi"("Replace match with:"="]", "Input String"=w332, "regular expression"=")") -> ("Output String"=w330:string)  [unwired: 2 out]
                  }
                }
                n169 = call "Merge_channel_names.vi"("Preferred Channel array"=w322, "Channel array"=w321) -> ("Merged Channels"=w316:string[], "Preferred Channels Changed?"=w324:bool, "Channel Array Changed?"=w325:bool)
                n170 = for {
                  tunnel: w316 -> [w354] mode=indexing
                  tunnel: [w351] -> w317 mode=indexing
                  n171 = call "Fast_string_Replace.vi"("Replace match with:"=" ", "Input String"=w354, "regular expression"=":") -> ("Output String"=w350:string)  [unwired: 2 out]
                  n172 = call "Fast_string_Replace.vi"("Replace match with:"=" ", "Input String"=w350, "regular expression"="  ") -> ("Output String"=w349:string)  [unwired: 2 out]
                  n173 = call <vilib>:"Trim Whitespace.vi"("string"=w349) -> ("trimmed string"=w351:string)  [unwired: 1 in]
                }
                n174 = case shown="True" w324 {
                  tunnel: w327 -> [w342 w344]
                  tunnel: w322 -> [_ w346]
                  tunnel: [w342 w343] -> w323
                  tunnel: w316 -> [_ w345]
                  frame False {
                  }
                  frame True {
                    n175 = call "Merge_2D_values.vi"("Values In"=w344, "Present Channels"=w346, "Desired Channels"=w345) -> ("Values Out"=w343:string[][])
                  }
                }
                n176 = case shown="True" w325 {
                  tunnel: [w337 w341] -> w326
                  tunnel: w321 -> [_ w340]
                  tunnel: w319 -> [w337 w339]
                  tunnel: w316 -> [_ w338]
                  frame False {
                  }
                  frame True {
                    n177 = call "Merge_2D_values.vi"("Values In"=w339, "Present Channels"=w340, "Desired Channels"=w338) -> ("Values Out"=w341:string[][])
                  }
                }
                n178 = global write "Results_plotter_Global.vi" "Channel names"(w317) -> ()
                n179 = global write "Results_plotter_Global.vi" "Full Ch Names"(w316) -> ()
                n180 = Build Array (concatenate)(w323, w326) -> (w318:string[][])
                n181 = global write "Results_plotter_Global.vi" "All Data"(w318) -> ()
              }
            }
          }
          frame #1 {
            n182 = local read "File Index"() -> (w359:i32)
            n183 = Decrement(x=w359) -> (x-1=w358:i32)
            n184 = local read "Result files to read"() -> (w356:path[])
            n185 = case shown="True" w360 {
              tunnel: w363 -> [_ w376]
              tunnel: w362 -> [_ w374]
              tunnel: w361 -> [_ w372]
              tunnel: w358 -> [w364 w370]
              tunnel: w357 -> [_ w369]
              tunnel: w356 -> [w366 w371]
              tunnel: [w365 w368] -> w355
              frame False {
                n186 = Delete From Array(array=w366, length=1, index=w364) -> (array with subset deleted=w365:path[])  [unwired: 1 out]
                n187 = local write "File Index"(w364) -> ()
              }
              frame True {
                n188 = Array Size(array=w376) -> (size(s)=w378:i32[])
                n189 = Index Array(array=w378, index=0 ("Index")) -> (element=w375:i32)
                n190 = for {
                  tunnel: w370 -> [w395]
                  tunnel: [w394] -> w380 mode=indexing
                  tunnel: w375 -> [w391]
                  tunnel: w372 -> [w390] mode=indexing
                  i -> [w392]
                  n191 = Add(x=w392, y=w391) -> (x+y=w393:i32)
                  n192 = Build Array(w395, w390, w393) -> (w394:i32[])
                }
                n193 = case shown="1, Default" w370 {
                  tunnel: w380 -> [w383 w388]
                  tunnel: [w383 w387] -> w379
                  tunnel: w374 -> [w382 w386]
                  tunnel: [w381 w384] -> w373
                  frame 0 {
                    n194 = Build Array(w382) -> (w381:string[])
                  }
                  frame 1, Default {
                    n195 = global read "Results_plotter_Global.vi" "Row Reference"() -> (w389:i32[][])
                    n196 = local read "Filetype"() -> (w385:string[])
                    n197 = Build Array (concatenate)(w385, w386) -> (w384:string[])
                    n198 = Build Array (concatenate)(w389, w388) -> (w387:i32[][])
                  }
                }
                "Filetype" <- w373
                n199 = Replace Array Subset(array=w371, new element=w369, index=w370) -> (w368:path[])
                n200 = global write "Results_plotter_Global.vi" "Row Reference"(w379) -> ()
              }
            }
            n201 = local write "Result files to read"(w355) -> ()
          }
        }
      }
      frame "Load Selectors" {
        n202 = while {
          shift-right: [w416] -> w401
          shift-left: _ -> [w418]
          tunnel: [w418] -> w400
          tunnel: w396 -> [w416]
          stop <- FALSE continue-if-true
        }
        n203 = Array Size(array=w408) -> (size(s)=w407:i32[])
        n204 = local read "Tolerances"() -> (w404:dbl[])
        n205 = Index Array(array=w407, index=0 ("Index")) -> (element=→"nRows":i32)
        n206 = Equal?(x=w401, y=w400) -> (x = y?=w399:bool)
        n207 = Build Array (concatenate)("Don't Filter" ("Input Element"), w396) -> (w413:string[])
        n208 = Array Size(array=w396) -> (size(s)=w410:i32)
        n209 = Array Size(array=w404) -> (size(s)=w409:i32)
        n210 = property on="Multi Ordinate" class="LstBox (strict)"("Item Names"=w396) -> ()  [unwired: 2 in, 2 out]
        n211 = property on="Z Ch Name" class="Ring (strict)"("Strings []"=w396) -> ()  [unwired: 2 in, 2 out]
        n212 = property on="Y Ch Name" class="Ring (strict)"("Strings []"=w396) -> ()  [unwired: 2 in, 2 out]
        n213 = property on="X Ch Name" class="Ring (strict)"("Strings []"=w396) -> ()  [unwired: 2 in, 2 out]
        n214 = property on="X Axis" class="Ring (strict)"("Strings []"=w396) -> ()  [unwired: 2 in, 2 out]
        n215 = property on="Ordinate" class="Ring (strict)"("Strings []"=w396) -> ()  [unwired: 2 in, 2 out]
        n216 = property on="Filter on column 1:" class="Ring (strict)"("Strings []"=w413) -> ()  [unwired: 2 in, 2 out]
        n217 = Not Equal?(x=w410, y=w409) -> (x != y?=w411:bool)
        n218 = case shown="True" w411 {
          tunnel: w410 -> [_ w425]
          tunnel: w409 -> [_ w424]
          tunnel: w404 -> [_ w421]
          frame False {
          }
          frame True {
            n219 = Subtract(x=w425, y=w424) -> (x-y=w423:i32)
            n220 = Initialize Array(1.0 ("Element Data"), w423) -> (w420:dbl[])
            n221 = Build Array (concatenate)(w421, w420) -> (w419:dbl[])
            n222 = local write "Tolerances"(w419) -> ()
          }
        }
        n223 = global write "Results_plotter_Global.vi" "First Loop"(TRUE) -> ()
        n224 = Select(t="What is present?", s=w399, f="Set Axis Channels") -> (s? t:f=w403:string)
      }
      frame "Set Axis Channels" {
        n225 = Array Size(array=w432) -> (size(s)=w431:i32)
        n226 = Build Array("X" ("regular expression"), "Y" ("regular expression"), "Z" ("regular expression")) -> (w426:string[])
        n227 = Decrement(x=w431) -> (x-1=w430:i32)
        n228 = for {
          tunnel: w432 -> [w444]
          tunnel: w430 -> [w443]
          tunnel: w426 -> [w442] mode=indexing
          i -> [w438]
          n229 = while {
            tunnel: w444 -> [w458] mode=indexing
            tunnel: w443 -> [w457]
            tunnel: w442 -> [w455]
            tunnel: [w448] -> w441
            tunnel: [w453] -> w440
            i -> [w453]
            stop <- w456 continue-if-true
            n230 = call "Match_Pat_Case_In.vi"("String to match"=w455, "String"=w458) -> ("offset past match"=w452:i32)  [unwired: 1 in, 3 out]
            n231 = In Range and Coerce(upper limit=4, x=w452, lower limit=0) -> (In Range?=w449:bool)  [unwired: 1 out]
            n232 = Less?(x=w453, y=w457) -> (x < y?=w454:bool)
            n233 = Not(x=w449) -> (.not. x?=w448:bool)
            n234 = And(x=w448, y=w454) -> (x .and. y?=w456:bool)
          }
          n235 = Select(t=0, s=w441, f=w440) -> (s? t:f=w437:i32)
          n236 = case shown="1" w438 {
            tunnel: w437 -> [w445 w446 w447]
            frame 0, Default {
              n237 = local write "X Ch Name"(w445) -> ()
            }
            frame 1 {
              n238 = local write "Y Ch Name"(w446) -> ()
            }
            frame 2 {
              n239 = local write "Z Ch Name"(w447) -> ()
            }
          }
        }
      }
      frame "What is present?" {
        n240 = case shown="True" "Show Results Space Analysis" {
          tunnel: w462 -> [_ w466]
          tunnel: w461 -> [_ w465]
          frame False {
          }
          frame True {
            n241 = stacked-sequence {
              tunnel: w466 -> [w470]
              tunnel: w465 -> [w469]
              frame #0 {
                w467 = FALSE  # Summarise All
                n242 = call "Summarise.vi"("Channel Names"=w470, "Data"=w469, "Summarise All"=w467) -> ("Summary"=w468:string[][])  [unwired: 2 in]
                n243 = call "Results_Space_Analysis.vi"("Table"=w468) -> ()
              }
            }
          }
        }
      }
      frame "Ordinate Selector Type" {
        n244 = while {
          tunnel: [w489] -> w480
          shift-left: _ -> [w489]
          shift-right: ["Slice mode"] -> w481
          stop <- FALSE continue-if-true
          "Previous slice mode" <- w489
        }
        n245 = Not(x="Multi Ordinate?") -> (.not. x?=w475:bool)
        n246 = property on="Multi Ordinate" class="LstBox (strict)"("Visible"="Multi Ordinate?") -> ()  [unwired: 2 in, 2 out]
        n247 = property on="Ordinate Name" class="Str"("Visible"="Multi Ordinate?") -> ()  [unwired: 2 in, 2 out]
        n248 = property on="Ordinate" class="Ring (strict)"("Visible"=w475) -> ()  [unwired: 2 in, 2 out]
        n249 = property on="First Add label" class="Str"("Visible"=w475) -> ()  [unwired: 2 in, 2 out]
        n250 = property on="2nd Add label" class="Str"("Visible"=w475) -> ()  [unwired: 2 in, 2 out]
        n251 = property on="Additional Y Values" class="Arr (strict)"("Visible"=w475) -> ()  [unwired: 2 in, 2 out]
        n252 = property on="Additional X Values" class="Arr (strict)"("Visible"=w475) -> ()  [unwired: 2 in, 2 out]
        n253 = Not Equal?(x=w481, y=w480) -> (x != y?=w472:bool)
        n254 = local read "Intensity Plot?"() -> (w479:bool)
        n255 = Or(x=w472, y="Update") -> (x .or. y?=w473:bool)
        n256 = global read "Results_plotter_Global.vi" "First Loop"() -> (w476:bool)
        n257 = case shown="False" "Multi Ordinate?" {
          frame False {
            n258 = Build Array("Ordinate") -> (w491:u16[])
            n259 = local write "Multi Ordinate"(w491) -> ()
          }
          frame True {
          }
        }
        n260 = Compound Arithmetic op=AND(invert w476, w473, w479) -> (w478:bool)
        "Slice mode Change?" <- w478
        n261 = Select(t="Change Slice mode", s=w478, f="Which rows are Non-Blank?") -> (s? t:f=w482:string)
      }
      frame "Change Slice mode" {
        n262 = local read "Previous slice mode"() -> (w495:T3)
        n263 = local read "Slice mode"() -> (w509:T3)
        n264 = case shown="\"YX Slice (Plan)\"" w509 {
          tunnel: [w521 w526 w533 w538 w545 w551] -> w508
          tunnel: "Y Ch Name" -> [w519 w526 w533 w539 w544 w549]
          tunnel: "X Ch Name" -> [w521 w525 w532 w537 w545 w550]
          tunnel: [w520 w527 w532 w537 w544 w549] -> w499
          tunnel: "Z Ch Name" -> [w520 w527 w531 w538 w543 w551]
          tunnel: [w519 w525 w531 w539 w543 w550] -> w497
          tunnel: w495 -> [w518 w523 w529 w535 w542 w547]
          tunnel: [w516 w522 w528 w534 w541 w546] -> w494
          frame "XY Slice (Plan)" {
            n265 = Equal?(x=Plot_Slice."YX Slice (Plan)" ("Previous slice mode"), y=w518) -> (x = y?=w516:bool)
          }
          frame "YX Slice (Plan)" {
            n266 = Equal?(x=Plot_Slice."XY Slice (Plan)" ("Previous slice mode"), y=w523) -> (x = y?=w522:bool)
          }
          frame "YZ Slice (Cross)" {
            n267 = Equal?(x=Plot_Slice."ZY Slice (Cross)" ("Previous slice mode"), y=w529) -> (x = y?=w528:bool)
          }
          frame "ZY Slice (Cross)" {
            n268 = Equal?(x=Plot_Slice."YZ Slice (Cross)" ("Previous slice mode"), y=w535) -> (x = y?=w534:bool)
          }
          frame "XZ Slice (Side)" {
            n269 = Equal?(x=Plot_Slice."ZX Slice (Side)" ("Previous slice mode"), y=w542) -> (x = y?=w541:bool)
          }
          frame "ZX Slice (Side)" {
            n270 = Equal?(x=Plot_Slice."XZ Slice (Side)" ("Previous slice mode"), y=w547) -> (x = y?=w546:bool)
          }
        }
        n271 = case shown="True" w494 {
          frame False {
          }
          frame True {
            n272 = local read "Transpose"() -> (w515:bool)
            n273 = Not(x=w515) -> (.not. x?=w514:bool)
            n274 = local write "Transpose"(w514) -> ()
          }
        }
        n275 = local write "Update"(FALSE ("Update")) -> ()
        n276 = Increment(x=w499) -> (x+1=w502:u16)
        n277 = Increment(x=w497) -> (x+1=w501:u16)
        n278 = local read "Filter Array"() -> (w506:u16[])
        n279 = Array Subset(array=w506, index=2 ("Array Index")) -> (w504:u16[])  [unwired: 1 in]
        n280 = Build Array (concatenate)(w502, w501, w504) -> (w503:u16[])
        n281 = local write "Filter Array"(w503) -> ()
        n282 = local write "Absisca"(w508) -> ()
      }
      frame "Which rows are Non-Blank?" {
        n283 = while {
          tunnel: [w568] -> w562
          tunnel: [w569] -> w563
          shift-left: _ -> [w570]
          shift-right: [w571] -> w555
          shift-left: _ -> [w573]
          shift-right: [w572] -> _
          stop <- FALSE continue-if-true
          n284 = local read "Multi Ordinate"() -> (w571:i32[])
          n285 = local read "Absisca"() -> (w572:u16)
          n286 = Equal?(x=w572, y=w573) -> (x = y?=w569:bool)
          n287 = Equal?(x=w571, y=w570) -> (x = y?=w568:bool)
        }
        n288 = global read "Results_plotter_Global.vi" "First Loop"() -> (w557:bool)
        n289 = Compound Arithmetic op=AND(invert w557, w563, w562) -> (w561:bool)
        n290 = Array Size(array=w555) -> (size(s)=w554:i32)
        n291 = Greater?(x=w554, y=1) -> (0:w552:bool)
        n292 = global write "Results_plotter_Global.vi" "Multi Ordinate?"(w552) -> ()
        n293 = Select(t="Create Selectors", s=w561, f="Evaluate Blank Rows") -> (s? t:f=w558:string)
      }
      frame "Evaluate Blank Rows" {
        n294 = local read "Multi Ordinate"() -> (w575:i32[])
        n295 = local read "Absisca"() -> (w576:u16)
        n296 = for {
          tunnel: w577 -> [w583] mode=indexing
          tunnel: w576 -> [w586]
          tunnel: w575 -> [w585]
          tunnel: [w582] -> w574 mode=indexing
          n297 = Index Array(array=w583, index=w586) -> (element=w587:string)
          n298 = call "Convert_to_number.vi"("string"=w587) -> ("Number"=w588:dbl)  [unwired: 1 out]
          n299 = Not A Number/Path/Refnum?(number/path/refnum=w588) -> (NaN/Path/Refnum?=w584:bool)
          n300 = case shown="False" w584 {
            tunnel: w585 -> [w592 _]
            tunnel: w583 -> [w591 _]
            tunnel: [w589 FALSE] -> w582
            frame False {
              n301 = for {
                tunnel: w592 -> [w598] mode=indexing
                tunnel: w591 -> [w596]
                tunnel: [w593] -> w590 mode=indexing
                n302 = Index Array(array=w596, index=w598) -> (element=w597:string)
                n303 = call "Convert_to_number.vi"("string"=w597) -> ("Number"=w595:dbl)  [unwired: 1 out]
                n304 = Not A Number/Path/Refnum?(number/path/refnum=w595) -> (NaN/Path/Refnum?=w594:bool)
                n305 = Not(x=w594) -> (.not. x?=w593:bool)
              }
              n306 = Or Array Elements(Boolean array=w590) -> (logical OR=w589:bool)
            }
            frame True {
            }
          }
        }
        "Non-Blank Rows" <- w574
      }
      frame "Create Selectors" {
        n307 = local read "Non-Blank Rows"() -> (w603:bool[])
        n308 = local read "Tolerances"() -> (w601:dbl[])
        n309 = global read "Results_plotter_Global.vi" "Precision"() -> (w600:string[])
        n310 = Array Size(array=w611) -> (size(s)=w610:i32[])
        n311 = Index Array(array=w610, index=0 ("Index")) -> (element=w613:i32)
        n312 = for {
          tunnel: w611 -> [w629]
          tunnel: "Filter Array" -> [w621] mode=indexing
          shift-right: [w628] -> w602
          shift-left: _ -> [w626]
          tunnel: w613 -> [w627]
          tunnel: [w624] -> w608 mode=indexing
          tunnel: w603 -> [w623]
          tunnel: w601 -> [w622]
          tunnel: w600 -> [w619]
          i -> [w625]
          n313 = Decrement(x=w621) -> (x-1=w618:u16)
          n314 = Index Array(array=w619, index=w618) -> (element=w617:string)
          n315 = Index Array(array=w622, index=w618) -> (element=w620:dbl)
          n316 = case shown="0, Default" w625 {
            tunnel: w629 -> [w642 w678 w719 w760 w801 w844 w885]
            tunnel: w621 -> [w641 w677 w718 w759 w800 w843 w884]
            tunnel: w620 -> [w640 w676 w717 w758 w799 w842 w883]
            tunnel: [w639 w675 w716 w757 w798 w841 w882] -> w628
            tunnel: w627 -> [w637 w674 w715 w756 w797 w840 w881]
            tunnel: w626 -> [_ w673 w714 w755 w796 w839 w880]
            tunnel: w625 -> [w636 w672 w711 w752 w793 w838 w877]
            tunnel: [w632 w667 w710 w751 w792 w833 w876] -> w624
            tunnel: w623 -> [w631 w666 w709 w750 w791 w832 w875]
            tunnel: w617 -> [w630 w665 w708 w749 w790 w831 w874]
            frame 0, Default {
              n317 = case shown="1, Default" w641 {
                tunnel: w642 -> [w648 w658]
                tunnel: w641 -> [w649 w657]
                tunnel: w640 -> [_ w664]
                tunnel: [w644 w661] -> w639
                tunnel: "Filter Bins 1" -> [_ w662]
                tunnel: [string[] [] ("Write Attribute") w663] -> w638
                tunnel: w637 -> [w646 _]
                tunnel: w636 -> [w652 w660]
                tunnel: [i32[] [0] ("Filter Bins Out") w659] -> w634
                tunnel: [TRUE ("Unchanged?") w656] -> w632
                tunnel: w631 -> [_ w655]
                tunnel: w630 -> [_ w654]
                frame 0 {
                  n318 = call "Create_filter_points.vi"("Channel to Filter On"=w649, "Index"=w652, "Ch Values In"=w648) -> ()  [unwired: 4 in, 4 out]
                  n319 = Initialize Array(TRUE, w646) -> (w645:bool[])
                  n320 = Build Array(w645) -> (w644:bool[][])
                }
                frame 1, Default {
                  n321 = call "Create_filter_points.vi"("Non-Blank Rows"=w655, "Precision"=w654, "Channel to Filter On"=w657, "Tolerance"=w664, "Index"=w660, "Filter Bins 1"=w662, "Ch Values In"=w658) -> ("Unchanged?"=w656:bool, "Accept array"=w661:bool[][], "Filter Bins Out"=w659:i32[], "Bin Names"=w663:string[])
                }
              }
              n322 = Equal?(x="Filter Bins 1", y=w634) -> (x = y?=w633:bool)
              n323 = case shown="False" w633 {
                tunnel: w634 -> [w643 _]
                frame False {
                  n324 = local write "Filter Bins 1"(w643) -> ()
                }
                frame True {
                }
              }
              n325 = property on="Filter bins 1" class="LstBox (strict)"("Item Names"=w638) -> ()  [unwired: 2 in, 2 out]
            }
            frame 1 {
              n326 = case shown="0" w677 {
                tunnel: w678 -> [_ w690]
                tunnel: w677 -> [w681 w689]
                tunnel: w676 -> [_ w697]
                tunnel: [w685 w693] -> w675
                tunnel: "Filter Bins 2" -> [_ w695]
                tunnel: [string[] [] ("Write Attribute") w699] -> w671
                tunnel: w674 -> [_ _]
                tunnel: w673 -> [w685 w698]
                tunnel: w672 -> [w684 w696]
                tunnel: [i32[] [0] ("Filter Bins Out") w691] -> w670
                tunnel: [TRUE ("Unchanged?") w688] -> w667
                tunnel: w666 -> [_ w687]
                tunnel: w665 -> [_ w686]
                frame 0 {
                  n327 = call "Create_filter_points.vi"("Channel to Filter On"=w681, "Index"=w684) -> ()  [unwired: 5 in, 4 out]
                }
                frame 1, Default {
                  n328 = call "Create_filter_points.vi"("Non-Blank Rows"=w687, "Precision"=w686, "Channel to Filter On"=w689, "Tolerance"=w697, "Index"=w696, "Filter Bins 1"=w695, "Ch Values In"=w690) -> ("Unchanged?"=w688:bool, "Accept array"=w694:bool[][], "Filter Bins Out"=w691:i32[], "Bin Names"=w699:string[])
                  n329 = for {
                    tunnel: w698 -> [w704]
                    tunnel: w694 -> [w703] mode=indexing
                    shift-right: [w700] -> w693
                    shift-left: bool[][] [] -> [w702]
                    n330 = for {
                      tunnel: w703 -> [w707]
                      tunnel: w704 -> [w706] mode=indexing
                      tunnel: [w705] -> _ mode=indexing
                      tunnel: [w705] -> w701 mode=indexing
                      n331 = And(x=w707, y=w706) -> (x .and. y?=w705:bool[])
                    }
                    n332 = Build Array (concatenate)(w702, w701) -> (w700:bool[][])
                  }
                }
              }
              n333 = Equal?(x="Filter Bins 2", y=w670) -> (x = y?=w668:bool)
              n334 = case shown="False" w668 {
                tunnel: w670 -> [w679 _]
                frame False {
                  n335 = local write "Filter Bins 2"(w679) -> ()
                }
                frame True {
                }
              }
              n336 = property on="Filter Bins 2" class="LstBox (strict)"("Item Names"=w671) -> ()  [unwired: 2 in, 2 out]
            }
            frame 2 {
              n337 = case shown="0" w718 {
                tunnel: w719 -> [_ w729]
                tunnel: w718 -> [w722 w730]
                tunnel: w717 -> [_ w741]
                tunnel: [w725 w742] -> w716
                tunnel: "Filter 3" -> [_ w733]
                tunnel: [string[] [] ("Write Attribute") w744] -> w712
                tunnel: w715 -> [_ _]
                tunnel: w714 -> [w725 w743]
                tunnel: w711 -> [w724 w736]
                tunnel: [TRUE ("Unchanged?") w728] -> w710
                tunnel: w709 -> [_ w727]
                tunnel: w708 -> [_ w726]
                frame 0 {
                  n338 = call "Create_filter_points.vi"("Channel to Filter On"=w722, "Index"=w724) -> ()  [unwired: 5 in, 4 out]
                  n339 = local write "Filter 3"(0) -> ()
                }
                frame 1, Default {
                  n340 = Build Array(w733) -> (w740:u16[])
                  n341 = call "Create_filter_points.vi"("Non-Blank Rows"=w727, "Precision"=w726, "Channel to Filter On"=w730, "Tolerance"=w741, "Index"=w736, "Filter Bins 1"=w740, "Ch Values In"=w729) -> ("Unchanged?"=w728:bool, "Accept array"=w738:bool[][], "Filter Bins Out"=w734:i32[], "Bin Names"=w744:string[])
                  n342 = Index Array(array=w734, index=0 ("Index")) -> (element=w731:i32)
                  n343 = Index Array(array=w738, index (row)=0 ("Index")) -> (element=w737:bool[])  [unwired: 1 in]
                  n344 = Equal?(x=w733, y=w731) -> (x = y?=w732:bool)
                  n345 = case shown="True" w732 {
                    tunnel: w731 -> [w745 _]
                    frame False {
                      n346 = local write "Filter 3"(w745) -> ()
                    }
                    frame True {
                    }
                  }
                  n347 = for {
                    tunnel: w737 -> [w748]
                    tunnel: w743 -> [w747] mode=indexing
                    tunnel: [w746] -> w742 mode=indexing
                    n348 = And(x=w748, y=w747) -> (x .and. y?=w746:bool[])
                  }
                }
              }
              n349 = property on="Filter 3" class="Ring (strict)"("Strings []"=w712) -> ()  [unwired: 2 in, 2 out]
            }
            frame 3 {
              n350 = case shown="1, Default" w759 {
                tunnel: w760 -> [_ w771]
                tunnel: w759 -> [w763 w770]
                tunnel: w758 -> [_ w782]
                tunnel: [w766 w783] -> w757
                tunnel: "Filter 4" -> [_ w774]
                tunnel: [string[] [] ("Write Attribute") w785] -> w753
                tunnel: w756 -> [_ _]
                tunnel: w755 -> [w766 w784]
                tunnel: w752 -> [w765 w777]
                tunnel: [TRUE ("Unchanged?") w769] -> w751
                tunnel: w750 -> [_ w768]
                tunnel: w749 -> [_ w767]
                frame 0 {
                  n351 = call "Create_filter_points.vi"("Channel to Filter On"=w763, "Index"=w765) -> ()  [unwired: 5 in, 4 out]
                  n352 = local write "Filter 4"(0) -> ()
                }
                frame 1, Default {
                  n353 = Build Array(w774) -> (w781:u16[])
                  n354 = call "Create_filter_points.vi"("Non-Blank Rows"=w768, "Precision"=w767, "Channel to Filter On"=w770, "Tolerance"=w782, "Index"=w777, "Filter Bins 1"=w781, "Ch Values In"=w771) -> ("Unchanged?"=w769:bool, "Accept array"=w779:bool[][], "Filter Bins Out"=w775:i32[], "Bin Names"=w785:string[])
                  n355 = Index Array(array=w775, index=0 ("Index")) -> (element=w773:i32)
                  n356 = Equal?(x=w774, y=w773) -> (x = y?=w772:bool)
                  n357 = Index Array(array=w779, index (row)=0 ("Index")) -> (element=w778:bool[])  [unwired: 1 in]
                  n358 = case shown="False" w772 {
                    tunnel: w773 -> [w786 _]
                    frame False {
                      n359 = local write "Filter 4"(w786) -> ()
                    }
                    frame True {
                    }
                  }
                  n360 = for {
                    tunnel: w778 -> [w789]
                    tunnel: w784 -> [w788] mode=indexing
                    tunnel: [w787] -> w783 mode=indexing
                    n361 = And(x=w789, y=w788) -> (x .and. y?=w787:bool[])
                  }
                }
              }
              n362 = property on="Filter 4" class="Ring (strict)"("Strings []"=w753) -> ()  [unwired: 2 in, 2 out]
            }
            frame 4 {
              n363 = case shown="1, Default" w800 {
                tunnel: w801 -> [_ w812]
                tunnel: w800 -> [w804 w811]
                tunnel: w799 -> [_ w823]
                tunnel: [w807 w824] -> w798
                tunnel: "Filter 5" -> [_ w814]
                tunnel: [string[] [] ("Write Attribute") w826] -> w794
                tunnel: w797 -> [_ _]
                tunnel: w796 -> [w807 w825]
                tunnel: w793 -> [w806 w818]
                tunnel: [TRUE ("Unchanged?") w810] -> w792
                tunnel: w791 -> [_ w809]
                tunnel: w790 -> [_ w808]
                frame 0 {
                  n364 = call "Create_filter_points.vi"("Channel to Filter On"=w804, "Index"=w806) -> ()  [unwired: 5 in, 4 out]
                  n365 = local write "Filter 5"(0) -> ()
                }
                frame 1, Default {
                  n366 = Build Array(w814) -> (w822:u16[])
                  n367 = call "Create_filter_points.vi"("Non-Blank Rows"=w809, "Precision"=w808, "Channel to Filter On"=w811, "Tolerance"=w823, "Index"=w818, "Filter Bins 1"=w822, "Ch Values In"=w812) -> ("Unchanged?"=w810:bool, "Accept array"=w820:bool[][], "Filter Bins Out"=w816:i32[], "Bin Names"=w826:string[])
                  n368 = Index Array(array=w816, index=0 ("Index")) -> (element=w815:i32)
                  n369 = Equal?(x=w814, y=w815) -> (x = y?=w813:bool)
                  n370 = Index Array(array=w820, index (row)=0 ("Index")) -> (element=w819:bool[])  [unwired: 1 in]
                  n371 = case shown="False" w813 {
                    tunnel: w815 -> [w827 _]
                    frame False {
                      n372 = local write "Filter 5"(w827) -> ()
                    }
                    frame True {
                    }
                  }
                  n373 = for {
                    tunnel: w819 -> [w830]
                    tunnel: w825 -> [w829] mode=indexing
                    tunnel: [w828] -> w824 mode=indexing
                    n374 = And(x=w830, y=w829) -> (x .and. y?=w828:bool[])
                  }
                }
              }
              n375 = property on="Filter 5" class="Ring (strict)"("Strings []"=w794) -> ()  [unwired: 2 in, 2 out]
            }
            frame 5 {
              n376 = case shown="1, Default" w843 {
                tunnel: w844 -> [_ w861]
                tunnel: w843 -> [w847 w860]
                tunnel: w842 -> [_ w865]
                tunnel: [w851 w852] -> w841
                tunnel: "Single Series" -> [_ w863]
                tunnel: [string[] [] ("Write Attribute") w867] -> w837
                tunnel: w840 -> [_ _]
                tunnel: w839 -> [w851 w866]
                tunnel: w838 -> [w850 w864]
                tunnel: [i32[] [0] ("Filter Bins Out") w862] -> w836
                tunnel: [TRUE ("Unchanged?") w859] -> w833
                tunnel: w832 -> [_ w858]
                tunnel: w831 -> [_ w857]
                frame 0 {
                  n377 = call "Create_filter_points.vi"("Channel to Filter On"=w847, "Index"=w850) -> ()  [unwired: 5 in, 4 out]
                }
                frame 1, Default {
                  n378 = call "Create_filter_points.vi"("Non-Blank Rows"=w858, "Precision"=w857, "Channel to Filter On"=w860, "Tolerance"=w865, "Index"=w864, "Filter Bins 1"=w863, "Ch Values In"=w861) -> ("Unchanged?"=w859:bool, "Accept array"=w854:bool[][], "Filter Bins Out"=w862:i32[], "Bin Names"=w867:string[])
                  n379 = Index Array(array=w854, index (row)=0 ("Index")) -> (element=w855:bool[])  [unwired: 1 in]
                  n380 = for {
                    shift-right: [w868] -> w853
                    shift-left: w855 -> [w870]
                    tunnel: w854 -> [w869] mode=indexing
                    n381 = Or(x=w869, y=w870) -> (x .or. y?=w868:bool[])
                  }
                  n382 = for {
                    tunnel: w853 -> [w873]
                    tunnel: w866 -> [w872] mode=indexing
                    tunnel: [w871] -> w852 mode=indexing
                    n383 = And(x=w873, y=w872) -> (x .and. y?=w871:bool[])
                  }
                }
              }
              n384 = Equal?(x="Single Series", y=w836) -> (x = y?=w834:bool)
              n385 = case shown="False" w834 {
                tunnel: w836 -> [w845 _]
                frame False {
                  n386 = local write "Single Series"(w845) -> ()
                }
                frame True {
                }
              }
              n387 = property on="Single Series" class="LstBox (strict)"("Item Names"=w837) -> ()  [unwired: 2 in, 2 out]
            }
            frame 6 {
              n388 = case shown="1, Default" w884 {
                tunnel: w885 -> [_ w896]
                tunnel: w884 -> [w888 w895]
                tunnel: w883 -> [_ w903]
                tunnel: [w891 w908] -> w882
                tunnel: "Filter 6" -> [_ w898]
                tunnel: [string[] [] ("Write Attribute") w910] -> w878
                tunnel: w881 -> [_ _]
                tunnel: w880 -> [w891 w909]
                tunnel: w877 -> [w890 w902]
                tunnel: [TRUE ("Unchanged?") w894] -> w876
                tunnel: w875 -> [_ w893]
                tunnel: w874 -> [_ w892]
                frame 0 {
                  n389 = call "Create_filter_points.vi"("Channel to Filter On"=w888, "Index"=w890) -> ()  [unwired: 5 in, 4 out]
                  n390 = local write "Filter 6"(0) -> ()
                }
                frame 1, Default {
                  n391 = Build Array(w898) -> (w904:u16[])
                  n392 = call "Create_filter_points.vi"("Non-Blank Rows"=w893, "Precision"=w892, "Channel to Filter On"=w895, "Tolerance"=w903, "Index"=w902, "Filter Bins 1"=w904, "Ch Values In"=w896) -> ("Unchanged?"=w894:bool, "Accept array"=w906:bool[][], "Filter Bins Out"=w900:i32[], "Bin Names"=w910:string[])
                  n393 = Index Array(array=w900, index=0 ("Index")) -> (element=w899:i32)
                  n394 = Equal?(x=w898, y=w899) -> (x = y?=w897:bool)
                  n395 = Index Array(array=w906, index (row)=0 ("Index")) -> (element=w905:bool[])  [unwired: 1 in]
                  n396 = case shown="False" w897 {
                    tunnel: w899 -> [w911 _]
                    frame False {
                      n397 = local write "Filter 6"(w911) -> ()
                    }
                    frame True {
                    }
                  }
                  n398 = for {
                    tunnel: w905 -> [w914]
                    tunnel: w909 -> [w913] mode=indexing
                    tunnel: [w912] -> w908 mode=indexing
                    n399 = And(x=w914, y=w913) -> (x .and. y?=w912:bool[])
                  }
                }
              }
              n400 = property on="Filter 6" class="Ring (strict)"("Strings []"=w878) -> ()  [unwired: 2 in, 2 out]
            }
          }
        }
        "Accept Array" <- w602
        n401 = And Array Elements(Boolean array=w608) -> (logical AND=w607:bool)
        n402 = Select(t="Select all for Filter 2", s=w607, f="Create Selectors") -> (s? t:f=w605:string)
      }
      frame "Select all for Filter 2" {
        n403 = local read "Slice mode Change?"() -> (w924:bool)
        n404 = property on="Filter bins 1" class="LstBox (strict)"() -> ("Item Names"=w920:string[], "Top Row"=w919:i32)  [unwired: 2 in, 2 out]
        n405 = case shown="True" w924 {
          frame False {
          }
          frame True {
            n406 = property on="Filter Bins 2" class="LstBox (strict)"() -> ("Item Names"=w940:string[])  [unwired: 2 in, 2 out]
            n407 = Array Size(array=w940) -> (size(s)=w939:i32)
            n408 = Build Array("Blanks", "Numeric", "Non Numeric", "Non Blanks", "Show All" ("Input Element")) -> (w933:string[])
            n409 = local read "Filter Bins 1"() -> (w942:i32[])
            n410 = while {
              tunnel: w940 -> [w955] mode=indexing
              tunnel: w939 -> [w958]
              shift-right: [w949] -> w931
              shift-left: i32[] [] -> [w950]
              tunnel: w933 -> [w952]
              i -> [w951]
              stop <- w956 stop-if-true
              n411 = String Subset(string=w955, length (rest)=4 ("length (rest)")) -> (substring=w960:string)  [unwired: 1 out]
              n412 = Match Pattern(string=w955, regular expression=" (") -> (before substring=w953:string)  [unwired: 4 out]
              n413 = Search 1D Array(1D array=w952, element=w953) -> (index of element=w948:i32)  [unwired: 1 out]
              n414 = Equal?(x="NOT ", y=w960) -> (x = y?=w947:bool)
              n415 = Equal?(x=w958, y=w951) -> (x = y?=w957:bool)
              n416 = Less Than 0?(x=w948) -> (x < 0?=w946:bool)
              n417 = Or(x=w947, y=w957) -> (x .or. y?=w956:bool)
              n418 = Compound Arithmetic op=AND(w946, invert w947) -> (w945:bool)
              n419 = case shown="False" w945 {
                tunnel: w951 -> [_ w965]
                tunnel: w950 -> [w962 w964]
                tunnel: [w962 w963] -> w949
                frame False {
                }
                frame True {
                  n420 = Build Array (concatenate)(w964, w965) -> (w963:i32[])
                }
              }
            }
            n421 = Array Size(array=w942) -> (size(s)=w944:i32)
            n422 = case shown="1" w944 {
              tunnel: [w966 w969] -> w943
              tunnel: w942 -> [_ w968]
              tunnel: i32[] [1] ("Filter Bins 1") -> [w966 w967]
              frame 0, Default {
              }
              frame 1 {
                n423 = Index Array(array=w968, index=0 ("Index")) -> (element=w971:i32)
                n424 = Greater Than 0?(x=w971) -> (x > 0?=w970:bool)
                n425 = Select(t=w968, s=w970, f=w967) -> (s? t:f=w969:i32[])
              }
            }
            n426 = local write "Filter Bins 1"(w943) -> ()
            n427 = local write "Filter Bins 2"(w931) -> ()
          }
        }
        n428 = Array Size(array=w920) -> (size(s)=w921:i32)
        n429 = Less?(x=w921, y=w919) -> (x < y?=w922:bool)
        n430 = case shown="True" w922 {
          frame False {
          }
          frame True {
            n431 = property on="Filter bins 1" class="LstBox (strict)"("Top Row"=0 ("Active Row:Active Row Number")) -> ()  [unwired: 2 in, 2 out]
          }
        }
        n432 = property on="Filter Bins 2" class="LstBox (strict)"() -> ("Item Names"=w918:string[], "Top Row"=w916:i32)  [unwired: 2 in, 2 out]
        n433 = Array Size(array=w918) -> (size(s)=w917:i32)
        n434 = Less?(x=w917, y=w916) -> (x < y?=w915:bool)
        n435 = case shown="True" w915 {
          frame False {
          }
          frame True {
            n436 = property on="Filter Bins 2" class="LstBox (strict)"("Top Row"=0 ("Active Row:Active Row Number")) -> ()  [unwired: 2 in, 2 out]
          }
        }
      }
      frame "Re Plot Data?" {
        n437 = while {
          tunnel: [w1019] -> w982
          shift-left: _ -> [w1021]
          shift-right: [w1020] -> _
          tunnel: [w1024] -> w988
          shift-left: _ -> [w1022]
          shift-right: [w1023] -> _
          tunnel: [w1028] -> w990
          shift-left: _ -> [w1027]
          shift-right: [w1026] -> w974
          tunnel: [w1029] -> w991
          shift-left: _ -> [w1031]
          shift-right: [w1030] -> _
          tunnel: [w1033] -> w992
          shift-left: _ -> [w1032]
          shift-right: [w1025] -> _
          tunnel: [w1034] -> w994
          tunnel: [w1035] -> w995
          shift-left: _ -> [w1036]
          shift-right: [w1037] -> _
          shift-left: _ -> [w1039]
          shift-right: [w1038] -> _
          tunnel: [w1040] -> w975
          shift-left: _ -> [w1041]
          shift-right: [w1042] -> _
          tunnel: [w1017] -> w985
          shift-right: [w1014] -> _
          shift-left: _ -> [w1013]
          tunnel: [w1016] -> w984
          shift-right: [w1012] -> _
          shift-left: _ -> [w1015]
          tunnel: [w1009] -> w983
          shift-right: [w1010] -> _
          shift-left: _ -> [w1011]
          shift-right: [w1007] -> _
          shift-left: _ -> [w1008]
          tunnel: [w1006] -> w977
          stop <- FALSE continue-if-true
          n438 = local read "Ordinate Name"() -> (w1007:string)
          n439 = local read "Additional X Values"() -> (w1014:dbl[])
          n440 = local read "Additional Y Values"() -> (w1012:dbl[])
          n441 = local read "Intensity Plot?"() -> (w1026:bool)
          n442 = local read "color and symbol"() -> (w1010:bool)
          n443 = local read "Accept Array"() -> (w1042:bool[][])
          n444 = local read "No of Contours"() -> (w1023:i32)
          n445 = local read "Point Size"() -> (w1020:i32)
          n446 = local read "Multi Ordinate"() -> (w1037:i32[])
          n447 = local read "Resolution"() -> (w1030:dbl)
          n448 = local read "Transpose"() -> (w1025:bool)
          n449 = local read "Absisca"() -> (w1038:u16)
          n450 = Equal?(x=w1007, y=w1008) -> (x = y?=w1006:bool)
          n451 = Equal?(x=w1025, y=w1032) -> (x = y?=w1033:bool)
          n452 = Equal?(x=w1010, y=w1011) -> (x = y?=w1009:bool)
          n453 = Equal?(x=w1023, y=w1022) -> (x = y?=w1024:bool)
          n454 = Equal?(x=w1020, y=w1021) -> (x = y?=w1019:bool)
          n455 = Equal?(x=w1030, y=w1031) -> (x = y?=w1029:bool)
          n456 = Equal?(x=w1014, y=w1013) -> (x = y?=w1017:bool)
          n457 = Equal?(x=w1012, y=w1015) -> (x = y?=w1016:bool)
          n458 = Equal?(x=w1038, y=w1039) -> (x = y?=w1035:bool)
          n459 = Equal?(x=w1042, y=w1041) -> (x = y?=w1040:bool)
          n460 = Equal?(x=w1026, y=w1027) -> (x = y?=w1028:bool)
          n461 = Equal?(x=w1037, y=w1036) -> (x = y?=w1034:bool)
        }
        n462 = global read "Results_plotter_Global.vi" "First Loop"() -> (w986:bool)
        n463 = while {
          shift-right: [w1005] -> _
          shift-left: _ -> [w1004]
          shift-right: [w1002] -> _
          shift-left: _ -> [w1003]
          tunnel: [w1001] -> w981
          tunnel: [w1000] -> w980
          stop <- FALSE continue-if-true
          n464 = local read "Filter Bins 1"() -> (w1002:i32[])
          n465 = local read "Filter Bins 2"() -> (w1005:i32[])
          n466 = Equal?(x=w1002, y=w1003) -> (x = y?=w1000:bool)
          n467 = Equal?(x=w1005, y=w1004) -> (x = y?=w1001:bool)
        }
        n468 = Not(x=w974) -> (.not. x?=w978:bool)
        n469 = property on="Resolution" class="DigNum (strict)"("Visible"=w974) -> ()  [unwired: 2 in, 2 out]
        n470 = property on="Bkgnd Value" class="DigNum (strict)"("Visible"=w974) -> ()  [unwired: 2 in, 2 out]
        n471 = property on="Intensity Graph" class="IntGraph (strict)"("Visible"=w974) -> ()  [unwired: 2 in, 2 out]
        n472 = property on="XY Plot" class="XYGraph (strict)"("Visible"=w978) -> ()  [unwired: 2 in, 2 out]
        n473 = Compound Arithmetic op=AND(w981, w980) -> (w979:bool)
        n474 = Compound Arithmetic op=AND(w977, w979, w982, w983, w988, w991, w992, w995, w994, w975, w990, w985, w984, invert w986) -> (w973:bool)
        n475 = Select(t="What to do next?", s=w973, f="Prepare for Plotting") -> (s? t:f=w993:string)
      }
      frame "Prepare for Plotting" {
        n476 = local read "Filter Array"() -> (w1051:u16[])
        n477 = local read "Multi Ordinate"() -> (w1046:i32[])
        n478 = Index Array(array=w1051, index=0 ("Index")) -> (element=w1048:u16)
        n479 = Equal To 0?(x=w1048) -> (x = 0?=w1049:bool)
        n480 = for {
          tunnel: w1046 -> [w1057] mode=indexing
          tunnel: [w1056] -> w1044 mode=indexing
          tunnel: w1045 -> [w1055]
          n481 = Index Array(array=w1055, index=w1057) -> (element=w1056:string)
        }
        n482 = case shown="False" w1049 {
          tunnel: w1048 -> [w1063 _]
          tunnel: w1045 -> [w1061 _]
          tunnel: [w1058 string[] []] -> w1043
          frame False {
            n483 = Decrement(x=w1063) -> (x-1=w1062:u16)
            n484 = local read "Filter Bins 1"() -> (w1065:i32[])
            n485 = property on="Filter bins 1" class="LstBox (strict)"() -> ("Item Names"=w1064:string[])  [unwired: 2 in, 2 out]
            n486 = Index Array(array=w1061, index=w1062) -> (element=w1059:string)
            n487 = for {
              tunnel: w1065 -> [w1068] mode=indexing
              tunnel: w1064 -> [w1067]
              tunnel: [w1066] -> w1060 mode=indexing
              n488 = Index Array(array=w1067, index=w1068) -> (element=w1066:string)
            }
            n489 = Build Array (concatenate)(w1059, w1060) -> (w1058:string[])
          }
          frame True {
          }
        }
        n490 = global write "Results_plotter_Global.vi" "Ordinate Strings"(w1044) -> ()
        n491 = global write "Results_plotter_Global.vi" "Filter 1 Strings"(w1043) -> ()
      }
      frame "Prepare Filter2 strings" {
        n492 = local read "Filter Array"() -> (w1076:u16[])
        n493 = Index Array(array=w1076, index=1 ("Index")) -> (element=w1073:u16)
        n494 = Equal To 0?(x=w1073) -> (x = 0?=w1074:bool)
        n495 = case shown="False" w1074 {
          tunnel: w1073 -> [w1085 _]
          tunnel: w1072 -> [w1083 _]
          tunnel: [w1080 string[] []] -> w1070
          frame False {
            n496 = Decrement(x=w1085) -> (x-1=w1084:u16)
            n497 = local read "Filter Bins 2"() -> (w1087:i32[])
            n498 = property on="Filter Bins 2" class="LstBox (strict)"() -> ("Item Names"=w1086:string[])  [unwired: 2 in, 2 out]
            n499 = Index Array(array=w1083, index=w1084) -> (element=w1081:string)
            n500 = for {
              tunnel: w1087 -> [w1090] mode=indexing
              tunnel: w1086 -> [w1089]
              tunnel: [w1088] -> w1082 mode=indexing
              n501 = Index Array(array=w1089, index=w1090) -> (element=w1088:string)
            }
            n502 = Build Array (concatenate)(w1081, w1082) -> (w1080:string[])
          }
          frame True {
          }
        }
        n503 = global write "Results_plotter_Global.vi" "Filter 2 Strings"(w1070) -> ()
      }
      frame "Plot Data" {
        n504 = stacked-sequence {
          seq-local: [w1098 _ _] -> [_ w1136 _]
          seq-local: [w1099 _ _] -> [_ w1135 _]
          tunnel: w1096 -> [_ w1145 _]
          tunnel: [_ TRUE _] -> w1095
          tunnel: [_ _ w1163] -> w1094
          tunnel: w1093 -> [w1100 _ _]
          frame #0 {
            n505 = global read "Results_plotter_Global.vi" "Ordinate Strings"() -> (w1098:string[])
            n506 = for {
              tunnel: w1098 -> [w1102] mode=indexing
              tunnel: w1100 -> [w1105]
              tunnel: [w1103] -> w1099 mode=indexing
              n507 = String Length(string=w1102) -> (length=w1101:i32)
              n508 = for {
                tunnel: w1102 -> [w1109]
                tunnel: w1105 -> [w1106] mode=indexing
                shift-right: [w1113] -> w1103
                shift-left: -1 -> [w1111]
                tunnel: w1101 -> [w1107]
                i -> [w1112]
                n509 = String Subset(string=w1106, length (rest)=w1107) -> (substring=w1108:string)  [unwired: 1 out]
                n510 = Equal?(x=w1108, y=w1109) -> (x = y?=w1110:bool)
                n511 = case shown="True" w1110 {
                  tunnel: [w1127 w1130] -> w1113
                  tunnel: w1112 -> [w1126 _]
                  tunnel: w1111 -> [w1125 w1130]
                  tunnel: w1107 -> [w1124 _]
                  tunnel: w1106 -> [w1123 _]
                  frame True {
                    n512 = String Subset(string=w1123, offset (0)=w1124) -> (substring=w1118:string)  [unwired: 1 out]
                    n513 = call <vilib>:"Trim Whitespace.vi"("string"=w1118) -> ("trimmed string"=w1116:string)  [unwired: 1 in]
                    n514 = Equal?(x=w1116, y="Err") -> (x = y?=w1120:bool)
                    n515 = Equal?(x=w1116, y="err") -> (x = y?=w1117:bool)
                    n516 = Equal?(x=w1116, y="St Error") -> (x = y?=w1114:bool)
                    n517 = Compound Arithmetic op=OR(w1120, w1117, w1114) -> (w1119:bool)
                    n518 = case shown="True" w1119 {
                      tunnel: [w1128 w1129] -> w1127
                      tunnel: w1126 -> [w1128 _]
                      tunnel: w1125 -> [_ w1129]
                      frame True {
                      }
                      frame False {
                      }
                    }
                  }
                  frame False {
                  }
                }
              }
            }
          }
          frame #1 {
            n519 = global read "Results_plotter_Global.vi" "Filter 1 Strings"() -> (w1131:string[])
            n520 = global read "Results_plotter_Global.vi" "Filter 2 Strings"() -> (w1132:string[])
            n521 = local read "Accept Array"() -> (w1147:bool[][])
            n522 = local read "Multi Ordinate?"() -> (w1141:bool)
            n523 = Select(t=5, s=w1141, f=2 ("y")) -> (s? t:f=w1139:i32)
            n524 = global write "Results_plotter_Global.vi" "Ordinate"("Multi Ordinate") -> ()
            n525 = global write "Results_plotter_Global.vi" "Absisca"("Absisca") -> ()
            n526 = global write "Results_plotter_Global.vi" "Transpose"("Transpose") -> ()
            n527 = while {
              shift-right: [w1150] -> w1144
              shift-left: _ -> [w1151]
              tunnel: "color and symbol" -> [w1152]
              tunnel: w1139 -> [w1148]
              stop <- FALSE continue-if-true
              n528 = case shown="True" w1152 {
                tunnel: w1151 -> [w1159 w1161]
                tunnel: [w1158 w1161] -> w1150
                tunnel: w1148 -> [w1153 _]
                frame True {
                  n529 = Add(x=w1159, y=1) -> (x+y=w1156:i32)
                  n530 = local write "color and symbol"(FALSE ("color and symbol")) -> ()
                  n531 = Greater?(x=w1156, y=w1153) -> (0:w1157:bool)
                  n532 = Select(t=0, s=w1157, f=w1156) -> (s? t:f=w1158:i32)
                }
                frame False {
                }
              }
            }
            n533 = call "Plot_XY_data.vi"("Channel Values"=w1145, "Ordinate Strings"=w1136, "Swap color and symbol"=w1144, "Error Bar Chs"=w1135, "Accept Array"=w1147, "Filter 1 Strings"=w1131, "Filter 2 Strings"=w1132, "Ordinate"="Multi Ordinate", "Absisca"="Absisca", "Transpose"="Transpose") -> ("Accept Array Out"=→"Plotted Series":bool[][])  [unwired: 5 out]
          }
          frame #2 {
            n534 = Select(t="Intensity plot", s="Intensity Plot?", f="Add Legend and scales") -> (s? t:f=w1163:string)
            n535 = property on="Surface Area" class="DigNum (strict)"("Visible"="Intensity Plot?") -> ()  [unwired: 2 in, 2 out]
            n536 = property on="Surface Integral" class="DigNum (strict)"("Visible"="Intensity Plot?") -> ()  [unwired: 2 in, 2 out]
            n537 = property on="Surface Average" class="DigNum (strict)"("Visible"="Intensity Plot?") -> ()  [unwired: 2 in, 2 out]
            n538 = property on="X Ch Name" class="Ring (strict)"("Visible"="Intensity Plot?") -> ()  [unwired: 2 in, 2 out]
            n539 = property on="Y Ch Name" class="Ring (strict)"("Visible"="Intensity Plot?") -> ()  [unwired: 2 in, 2 out]
            n540 = property on="Z Ch Name" class="Ring (strict)"("Visible"="Intensity Plot?") -> ()  [unwired: 2 in, 2 out]
            n541 = property on="Point Size" class="Slide (strict)"("Visible"="Intensity Plot?") -> ()  [unwired: 2 in, 2 out]
            n542 = property on="No of Contours" class="DigNum (strict)"("Visible"="Intensity Plot?") -> ()  [unwired: 2 in, 2 out]
            n543 = property on="Slice mode" class="Enum (strict)"("Visible"="Intensity Plot?") -> ()  [unwired: 2 in, 2 out]
            n544 = property on="Plot Resolution" class="Bool (strict)"("Visible"="Intensity Plot?") -> ()  [unwired: 2 in, 2 out]
            n545 = property on="Update" class="Bool (strict)"("Visible"="Intensity Plot?") -> ()  [unwired: 2 in, 2 out]
          }
        }
        "Index when last plotted" <- w1092
      }
      frame "Add Legend and scales" {
        n546 = global read "Results_plotter_Global.vi" "Point info"() -> (w1177:T13)
        n547 = global read "Results_plotter_Global.vi" "Legend"() -> (w1178:string[])
        n548 = local read "Transpose"() -> (w1169:bool)
        n549 = global read "Results_plotter_Global.vi" "XY Graph Cluster"() -> (→"XY Plot":cluster{dbl[], dbl[]}[])
        n550 = global read "Results_plotter_Global.vi" "Plot Index values"() -> (w1172:dbl[][])
        n551 = for {
          tunnel: w1178 -> [w1208] mode=indexing
          tunnel: w1177 -> [w1217] mode=indexing
          tunnel: [w1218] -> w1182
          i -> [w1218]
          n552 = String Length(string=w1208) -> (length=w1214:i32)
          n553 = Subtract(x=w1214, y=2) -> (x-y=w1212:i32)
          n554 = String Subset(string=w1208, length (rest)=w1212) -> (substring=w1206:string)  [unwired: 1 out]
          n555 = call "Abbreviate_string.vi"("Input String"=w1206, "Max String Length"=35) -> ("Output String"=w1205:string)
          n556 = Unbundle By Name(w1217) -> ("Point Style"=w1216:u8, "Fill/Pt. Color"=w1215:u32)
          n557 = call "Fast_string_Replace.vi"("Replace match with:"="_", "Input String"=w1205, "regular expression"=" ") -> ("Output String"=w1209:string)  [unwired: 1 in, 1 out]
          n558 = property on="XY Plot" class="XYGraph (strict)"("Active Plot"=w1218, "Plot.Plot Name"=w1209, "Plot.Point Style"=w1216, "Plot.Fill/Point Color"=w1215, "Plot.Plot Color"=w1215, "LegAutosize"=FALSE ("Legend:Autosize")) -> ()  [unwired: 2 in, 2 out]
        }
        n559 = Select(t=1 ("index (row)"), s=w1169, f=0 ("index (row)")) -> (s? t:f=w1166:i32)
        n560 = Index Array(array=w1172, index (row)=w1166) -> (element=w1171:dbl[])  [unwired: 1 in]
        n561 = Array Max & Min(array=w1171) -> (max value=w1170:dbl)  [unwired: 3 out]
        n562 = Greater?(x=w1170, y=2680560000.0) -> (0:w1174:bool)
        n563 = case shown="False" w1174 {
          tunnel: [w1189 u8 7 ("X Scale.Format & Precision:Precision")] -> w1173
          tunnel: w1170 -> [w1195 _]
          frame False {
            n564 = Absolute Value(x=w1195) -> (abs(x)=w1188:dbl)
            n565 = In Range and Coerce(upper limit=100000.0 ("y"), x=w1188, lower limit=0.0001) -> (In Range?=w1192:bool)  [unwired: 1 out]
            n566 = Select(t=u8 0 ("f"), s=w1192, f=u8 1) -> (s? t:f=w1189:u8)
          }
          frame True {
          }
        }
        n567 = Increment(x=w1182) -> (x+1=w1181:i32)
        n568 = for {
          N: 10 -> [_]
          tunnel: w1181 -> [w1202]
          i -> [w1203]
          w1199 = u32 0
          n569 = Add(x=w1202, y=w1203) -> (x+y=w1201:i32)
          n570 = property on="XY Plot" class="XYGraph (strict)"("Active Plot"=w1201, "Plot.Plot Name"="" ("Write Attribute"), "Plot.Plot Color"=w1199, "Plot.Fill/Point Color"=w1199, "LegAutosize"=FALSE ("Legend:Autosize"), "PlotVisCheckbox"=TRUE ("Legend:Plot Visibility Checkbox Visible")) -> ()  [unwired: 2 in, 2 out]
        }
        n571 = local write "Warning!"("") -> ()
        n572 = property on="XY Plot" class="XYGraph (strict)"("X Scale.Format & Precision:Format"=w1173) -> ()  [unwired: 2 in, 2 out]
      }
      frame "Add Axis names" {
        n573 = local read "Multi Ordinate"() -> (w1233:i32[])
        n574 = for {
          tunnel: w1233 -> [w1250] mode=indexing
          shift-right: [w1247] -> w1226
          shift-left: "" -> [w1246]
          tunnel: w1234 -> [w1249]
          tunnel: [w1242] -> w1225
          i -> [w1242]
          n575 = Index Array(array=w1249, index=w1250) -> (element=w1248:string)
          n576 = String Length(string=w1246) -> (length=w1245:i32)
          n577 = Less?(x=w1245, y=40) -> (x < y?=w1243:bool)
          n578 = case shown="True" w1243 {
            tunnel: w1248 -> [_ w1255]
            tunnel: [w1251 w1254] -> w1247
            tunnel: w1246 -> [w1251 w1252]
            frame False {
            }
            frame True {
              n579 = Concatenate Strings(w1252, w1255, "   ") -> (w1254:string)
            }
          }
        }
        n580 = Greater Than 0?(x=w1225) -> (x > 0?=w1223:bool)
        n581 = local read "Transpose"() -> (w1236:bool)
        n582 = local read "Absisca"() -> (w1237:u16)
        n583 = Index Array(array=w1234, index=w1237) -> (element=w1235:string)
        n584 = String Length(string=w1226) -> (length=w1229:i32)
        n585 = Empty String/Path?(string/path="Ordinate Name") -> (empty?=w1224:bool)
        n586 = Subtract(x=w1229, y=3) -> (x-y=w1227:i32)
        n587 = Compound Arithmetic op=AND(invert w1224, w1223) -> (w1222:bool)
        n588 = String Subset(string=w1226, length (rest)=w1227) -> (substring=w1221:string)  [unwired: 1 out]
        n589 = Select(t="Ordinate Name", s=w1222, f=w1221) -> (s? t:f=w1219:string)
        n590 = case shown="False" w1236 {
          tunnel: [w1256 w1259] -> w1232
          tunnel: w1219 -> [w1257 w1259]
          tunnel: [w1257 w1258] -> w1231
          tunnel: w1235 -> [w1256 w1258]
          frame False {
          }
          frame True {
          }
        }
        n591 = global write "Results_plotter_Global.vi" "X Axis Name"(w1232) -> ()
        n592 = global write "Results_plotter_Global.vi" "Y Axis Name"(w1231) -> ()
        n593 = global write "Results_plotter_Global.vi" "Value plotted Name"(w1219) -> ()
        n594 = property on="XY Plot" class="XYGraph (strict)"("X Scale.Name Label.Text"=w1232, "Y Scale.Name Label.Text"=w1231) -> ()  [unwired: 2 in, 2 out]
      }
      frame "Intensity plot" {
        # "Max"
        # "Min"
        n595 = global read "Results_plotter_Global.vi" "XY Graph Cluster"() -> (w1260:cluster{dbl[], dbl[]}[])
        n596 = local read "Tolerances"() -> (w1265:dbl[])
        n597 = local read "Absisca"() -> (w1264:u16)
        n598 = local read "Transpose"() -> (w1261:bool)
        n599 = stacked-sequence {
          seq-local: [w1278 _ _ _ _ _ _ _ _ _ _ _ _ _] -> [_ _ _ w1343 w1350 _ w1377 _ _ _ _ _ _ _]
          seq-local: [_ w1294 _ _ _ _ _ _ _ _ _ _ _ _] -> [_ _ _ _ w1349 _ w1376 _ _ _ _ _ _ _]
          seq-local: [_ _ w1326 _ _ _ _ _ _ _ _ _ _ _] -> [_ _ _ _ _ _ w1385 _ _ _ _ _ _ _]
          seq-local: [_ _ _ _ _ _ w1387 _ _ _ _ _ _ _] -> [_ _ _ _ _ _ _ _ _ w1420 _ _ _ _]
          seq-local: [_ _ _ _ _ _ w1386 _ _ _ _ _ _ _] -> [_ _ _ _ _ _ _ _ _ w1421 _ _ _ _]
          seq-local: [_ w1290 _ _ _ _ _ _ _ _ _ _ _ _] -> [_ _ _ _ _ _ _ _ _ _ w1485 _ _ _]
          seq-local: [_ _ _ w1341 _ _ _ _ _ _ _ _ _ _] -> [_ _ _ _ w1348 _ w1381 _ _ _ _ _ _ _]
          seq-local: [_ _ _ _ _ _ _ _ _ _ _ _ w1511 _] -> [_ _ _ _ _ _ _ _ _ _ _ _ _ w1561]
          seq-local: [_ _ _ _ _ _ _ _ _ _ _ _ w1510 _] -> [_ _ _ _ _ _ _ _ _ _ _ _ _ w1562]
          seq-local: [_ _ _ w1340 _ _ _ _ _ _ _ _ _ _] -> [_ _ _ _ _ w1363 _ _ _ _ _ _ _ _]
          seq-local: [_ _ _ _ _ _ _ _ _ _ _ _ w1508 _] -> [_ _ _ _ _ _ _ _ _ _ _ _ _ w1554]
          seq-local: [_ _ _ _ _ _ w1369 _ _ _ _ _ _ _] -> [_ _ _ _ _ _ _ w1398 _ _ _ _ _ _]
          tunnel: [_ _ _ TRUE _ _ _ _ _ _ _ _ _ _] -> w1271
          tunnel: [_ _ _ _ _ _ _ _ _ _ _ _ _ "Analyse Plot Space"] -> w1270
          tunnel: w1268 -> [w1275 _ _ _ _ _ _ _ _ _ _ _ _ _]
          tunnel: w1269 -> [w1276 _ w1327 _ _ _ _ _ _ _ w1466 _ _ _]
          tunnel: [w1276 _ _ _ _ _ _ _ _ _ _ _ _ _] -> w1267
          tunnel: [w1275 _ _ _ _ _ _ _ _ _ _ _ _ _] -> w1266
          tunnel: w1265 -> [w1280 _ _ _ _ _ _ _ _ _ _ _ _ _]
          tunnel: w1260 -> [w1279 _ _ w1345 _ _ _ _ _ _ _ _ _ _]
          tunnel: w1264 -> [w1277 _ _ _ _ _ _ _ _ _ w1482 _ _ _]
          tunnel: w1261 -> [w1274 _ _ w1342 _ _ w1389 _ _ _ w1480 _ _ _]
          tunnel: [_ w1295 _ _ _ _ _ _ _ _ _ _ _ _] -> w1263
          tunnel: w1262 -> [_ w1295 _ _ _ _ _ _ _ _ w1467 _ _ _]
          frame #0 {
            n600 = Not(x=w1274) -> (.not. x?=w1273:bool)
            n601 = for {
              tunnel: w1279 -> [w1289] mode=indexing
              tunnel: w1273 -> [w1286]
              shift-right: [w1284] -> w1281
              shift-left: dbl[] [] -> [w1285]
              n602 = Unbundle(w1289) -> (w1288:dbl[], w1287:dbl[])
              n603 = Select(t=w1288, s=w1286, f=w1287) -> (s? t:f=w1283:dbl[])
              n604 = Build Array (concatenate)(w1285, w1283) -> (w1284:dbl[])
            }
            n605 = Index Array(array=w1280, index=w1277) -> (element=w1272:dbl)
            n606 = call "Numeric_bins.vi"("Values"=w1281, "Tolerance"=w1272) -> ("Bin Centres"=w1278:dbl[])  [unwired: 2 out]
          }
          frame #1 {
            n607 = local read "Filter Bins 2"() -> (w1296:i32[])
            n608 = local read "Filter Bins 1"() -> (w1298:i32[])
            n609 = Array Size(array=w1296) -> (size(s)=w1300:i32)
            n610 = Array Size(array=w1298) -> (size(s)=w1301:i32)
            n611 = Greater Or Equal?(x=w1301, y=w1300) -> (x >= y?=w1299:bool)
            n612 = case shown="False" w1299 {
              tunnel: w1298 -> [_ w1323]
              tunnel: [w1319 w1323] -> w1297
              tunnel: [w1320 w1322] -> w1292
              tunnel: w1296 -> [w1319 _]
              tunnel: [1 0] -> w1290
              frame False {
                n613 = property on="Filter Bins 2" class="LstBox (strict)"() -> ("Item Names"=w1320:string[])  [unwired: 2 in, 2 out]
              }
              frame True {
                n614 = property on="Filter Bins 1" class="LstBox (strict)"() -> ("Item Names"=w1322:string[])  [unwired: 2 in, 2 out]
              }
            }
            n615 = Array Size(array=w1292) -> (size(s)=w1291:i32)
            n616 = for {
              tunnel: w1297 -> [w1306] mode=indexing
              tunnel: w1292 -> [w1312]
              shift-right: [w1309] -> w1294
              shift-left: dbl[] [] -> [w1310]
              tunnel: w1291 -> [w1305]
              n617 = Index Array(array=w1312, index=w1306) -> (element=w1308:string)
              n618 = Less?(x=w1306, y=w1305) -> (x < y?=w1304:bool)
              n619 = Match Pattern(string=w1308, regular expression=" (0)") -> (offset past match=w1307:i32)  [unwired: 4 out]
              n620 = Less Than 0?(x=w1307) -> (x < 0?=w1303:bool)
              n621 = And(x=w1303, y=w1304) -> (x .and. y?=w1302:bool)
              n622 = case shown="True" w1302 {
                tunnel: w1310 -> [w1313 w1317]
                tunnel: [w1313 w1316] -> w1309
                tunnel: w1308 -> [_ w1315]
                frame False {
                }
                frame True {
                  n623 = Fract/Exp String To Number(string=w1315) -> (number=w1314:dbl)  [unwired: 4 out]
                  n624 = Build Array (concatenate)(w1317, w1314) -> (w1316:dbl[])
                }
              }
            }
          }
          frame #2 {
            n625 = local read "Template"() -> (w1325:path)
            n626 = call "Valid_Path.vi"("Filename"=w1325) -> ("Valid Path?"=w1324:bool)
            n627 = case shown="True" w1324 {
              tunnel: w1325 -> [_ w1337]
              tunnel: w1327 -> [_ w1336]
              tunnel: [nan w1333] -> w1326
              frame False {
              }
              frame True {
                n628 = local read "Multi Ordinate"() -> (w1332:i32[])
                n629 = call "Read_Write_Template.vi"("Template File"=w1337, "Mode"=Global_mode."Read Global", "Channel names In"=w1336, "Data type"="Minimum Value") -> ("1D Info Out"=w1335:string[])  [unwired: 4 in, 7 out]
                n630 = Index Array(array=w1332, index=0 ("Index")) -> (element=w1331:i32)
                n631 = Index Array(array=w1335, index=w1331) -> (element=w1334:string)
                n632 = Fract/Exp String To Number(string=w1334, default (0 dbl)=nan) -> (number=w1333:dbl)  [unwired: 3 out]
              }
            }
          }
          frame #3 {
            n633 = call "Grid_Data.vi"("Transpose"=w1342, "XY Graph"=w1345, "Bin Centres"=w1343) -> ("No of Duplicates"=w1340:i32, "Grided data"=w1341:dbl[][])
          }
          frame #4 {
            n634 = for {
              tunnel: w1350 -> [w1355]
              tunnel: w1349 -> [w1354] mode=indexing
              tunnel: w1348 -> [w1353] mode=indexing
              shift-right: [w1351] -> w1346
              shift-left: dbl[][] [] -> [w1352]
              n635 = for {
                tunnel: w1355 -> [w1361] mode=indexing
                tunnel: w1354 -> [w1356]
                tunnel: w1353 -> [w1360] mode=indexing
                shift-right: [w1357] -> w1351
                shift-left: w1352 -> [w1359]
                n636 = Build Array(w1361, w1356, w1360) -> (w1358:dbl[])
                n637 = Build Array (concatenate)(w1359, w1358) -> (w1357:dbl[][])
              }
            }
            n638 = global write "Results_plotter_Global.vi" "Intensity Plot data in rows"(w1346) -> ()
          }
          frame #5 {
            n639 = case shown="1, Default" w1363 {
              tunnel: w1363 -> [_ w1367]
              tunnel: ["" w1365] -> w1362
              frame 0 {
              }
              frame 1, Default {
                n640 = Format Into String(format string="%d duplicate points have been averaged together!", w1367) -> (resulting string=w1365:string)  [unwired: 2 in, 1 out]
              }
            }
            "Warning!" <- w1362
          }
          frame #6 {
            n641 = call "Insert_extra_rows_and_col.vi"("Row Values In"=w1376, "Additional Row Values"="Additional X Values", "Column Values In"=w1377, "Data In"=w1381, "Additional Column Values"="Additional Y Values") -> ("Row Values Out"=w1378:dbl[], "Column Values Out"=w1379:dbl[], "Data Out"=w1380:dbl[][])  [unwired: 2 out]
            n642 = Select(t="Resolution", s="Plot Resolution", f=0.0) -> (s? t:f=w1371:dbl)
            n643 = call "2D_interpolation.vi"("X Axis Current"=w1379, "Min Z Value In"=w1385, "Y axis Current"=w1378, "Bkgnd Value"="Bkgnd Value", "Plot In"=w1380, "Increment Value"=w1371, "Transpose"=w1389, "Point Size"="Point Size") -> ("min Z value"=w1387:dbl, "max Z value"=w1386:dbl, "Increment Value Out"=w1375:dbl, "Axis info"=w1369:T14, "Plot Out"=→"Intensity Graph":dbl[][], "Raw Interpolation"=w1368:dbl[][])  [unwired: 2 out]
            n644 = global write "Results_plotter_Global.vi" "Raw Interpolation"(w1368) -> ()
            n645 = local write "Resolution"(w1375) -> ()
          }
          frame #7 {
            n646 = Unbundle By Name(w1398) -> ("X Max"=w1397:dbl, "Y Max"=w1396:dbl, "X Scale"=w1395:cluster{"Xo":dbl, "delta X":dbl}, "Y Scale"=w1394:cluster{"Xo":dbl, "delta X":dbl}, "X Values"=w1393:dbl[], "Y Values"=w1392:dbl[], "Z Max"=w1391:dbl, "Z Min"=w1390:dbl)
            n647 = global write "Results_plotter_Global.vi" "X Scale"(w1395) -> ()
            n648 = global write "Results_plotter_Global.vi" "X Values"(w1393) -> ()
            n649 = global write "Results_plotter_Global.vi" "Y Values"(w1392) -> ()
            n650 = global write "Results_plotter_Global.vi" "Y Scale"(w1394) -> ()
            n651 = global write "Results_plotter_Global.vi" "Y Max"(w1396) -> ()
            n652 = global write "Results_plotter_Global.vi" "Z Max"(w1391) -> ()
            n653 = global write "Results_plotter_Global.vi" "Z Min"(w1390) -> ()
            n654 = global write "Results_plotter_Global.vi" "X Max"(w1397) -> ()
          }
          frame #8 {
            n655 = global read "Results_plotter_Global.vi" "X Scale"() -> (w1406:cluster{"Xo":dbl, "delta X":dbl})
            n656 = global read "Results_plotter_Global.vi" "Y Scale"() -> (w1402:cluster{"Xo":dbl, "delta X":dbl})
            n657 = global read "Results_plotter_Global.vi" "Y Max"() -> (w1403:dbl)
            n658 = global read "Results_plotter_Global.vi" "X Max"() -> (w1404:dbl)
            n659 = Unbundle By Name(w1402) -> ("Xo"=w1401:dbl)
            n660 = Unbundle By Name(w1406) -> ("Xo"=w1405:dbl)
            n661 = Subtract(x=w1403, y=w1401) -> (x-y=w1407:dbl)
            n662 = Subtract(x=w1404, y=w1405) -> (x-y=w1416:dbl)
            n663 = Greater?(x=w1416, y=5.0) -> (0:w1414:bool)
            n664 = Greater?(x=w1407, y=5.0) -> (0:w1409:bool)
            n665 = Select(t=u8 0 ("Write Attribute"), s=w1414, f=u8 3) -> (s? t:f=w1400:u8)
            n666 = Select(t=u8 0 ("Write Attribute"), s=w1409, f=u8 3) -> (s? t:f=w1399:u8)
            n667 = property on="Intensity Graph" class="IntGraph (strict)"("X Scale.Offset and Multiplier"=w1406, "X Scale.Range:Maximum"=w1404, "Y Scale.Offset and Multiplier"=w1402, "Y Scale.Range:Maximum"=w1403, "X Scale.Format & Precision:Precision"=w1400, "Y Scale.Format & Precision:Precision"=w1399) -> ()  [unwired: 2 in, 2 out]
          }
          frame #9 {
            n668 = Greater Than 0?(x=w1421) -> (x > 0?=w1418:bool)
            n669 = Less Than 0?(x=w1420) -> (x < 0?=w1419:bool)
            n670 = And(x=w1418, y=w1419) -> (x .and. y?=w1417:bool)
            n671 = case shown="False" w1417 {
              tunnel: w1421 -> [w1450 w1464]
              tunnel: [w1458 w1462] -> w1423
              tunnel: w1420 -> [w1446 w1459]
              frame True {
                (unwired) u32 3743
                (unwired) u32 16721152
                n672 = Absolute Value(x=w1446) -> (abs(x)=w1445:dbl)
                n673 = Absolute Value(x=w1450) -> (abs(x)=w1452:dbl)
                n674 = Absolute Value(x=w1446) -> (abs(x)=w1453:dbl)
                n675 = Max & Min(x=w1452, y=w1453) -> (max(x,y)=w1448:dbl)  [unwired: 1 out]
                n676 = Divide(x=w1445, y=w1448) -> (x/y=w1439:dbl)
                n677 = Subtract(x=1.0, y=w1439) -> (x-y=w1438:dbl)
                n678 = Multiply(x=w1438, y=u32 255) -> (x*y=w1444:dbl)
                n679 = To Unsigned Long Integer(number=w1444) -> (unsigned 32bit integer=w1428:u32)
                n680 = Multiply(x=w1428, y=u32 256) -> (x*y=w1430:u32)
                n681 = Multiply(x=w1428, y=u32 65536) -> (x*y=w1427:u32)
                n682 = Compound Arithmetic op=ADD(w1427, w1430, u32 255) -> (w1426:u32)
                n683 = Bundle("min Z value"=w1446, w1426) -> (w1455:cluster{"min Z value":dbl, u32})  [unwired: 1 out]
                n684 = Divide(x=w1450, y=w1448) -> (x/y=w1443:dbl)
                n685 = Bundle("max Z value"=0.0, u32 16777215) -> (w1454:cluster{"max Z value":dbl, u32})  [unwired: 1 out]
                n686 = Subtract(x=1.0, y=w1443) -> (x-y=w1441:dbl)
                n687 = Multiply(x=w1441, y=u32 255) -> (x*y=w1437:dbl)
                n688 = To Unsigned Long Integer(number=w1437) -> (unsigned 32bit integer=w1424:u32)
                n689 = Multiply(x=w1424, y=u32 256) -> (x*y=w1434:u32)
                n690 = Compound Arithmetic op=ADD(w1424, w1434, u32 16711680) -> (w1425:u32)
                n691 = Bundle("max Z value"=w1450, w1425) -> (w1457:cluster{"max Z value":dbl, u32})  [unwired: 1 out]
                n692 = Build Array(w1457, w1455) -> (w1456:cluster{"min Z value":dbl, u32}[])
                n693 = Build Array (concatenate)(w1456, w1454) -> (w1458:cluster{"max Z value":dbl, u32}[])
              }
              frame False {
                n694 = Bundle("max Z value"=w1464, u32 16721152) -> (w1461:cluster{"max Z value":dbl, u32})  [unwired: 1 out]
                n695 = Bundle("min Z value"=w1459, u32 3743) -> (w1460:cluster{"min Z value":dbl, u32})  [unwired: 1 out]
                n696 = Build Array(w1461, w1460) -> (w1462:cluster{"min Z value":dbl, u32}[])
              }
            }
            n697 = property on="Intensity Graph" class="IntGraph (strict)"("Ignore Array"=FALSE ("Write Attribute"), "Z Scale.Marker Values[]"=w1423) -> ()  [unwired: 2 in, 2 out]
          }
          frame #10 {
            n698 = local read "Filter Array"() -> (w1484:u16[])
            n699 = Index Array(array=w1484, index=w1485) -> (element=w1483:u16)
            n700 = Decrement(x=w1483) -> (x-1=w1481:u16)
            n701 = local read "Multi Ordinate"() -> (w1471:i32[])
            n702 = Index Array(array=w1467, index=w1481) -> (element=w1475:string)
            n703 = Index Array(array=w1467, index=w1482) -> (element=w1474:string)
            n704 = case shown="False" w1480 {
              tunnel: [w1487 w1489] -> w1473
              tunnel: w1475 -> [w1487 w1488]
              tunnel: w1474 -> [w1486 w1489]
              tunnel: [w1486 w1488] -> w1472
              frame False {
              }
              frame True {
              }
            }
            n705 = Index Array(array=w1471, index=0) -> (element=w1469:i32)
            n706 = Index Array(array=w1466, index=w1469) -> (element=w1468:string)
            n707 = global write "Results_plotter_Global.vi" "Value plotted Name"(w1468) -> ()
            n708 = property on="Intensity Graph" class="IntGraph (strict)"("X Scale.Name Label.Text"=w1472, "Y Scale.Name Label.Text"=w1473) -> ()  [unwired: 2 in, 2 out]
            n709 = global write "Results_plotter_Global.vi" "Y Axis Name"(w1472) -> ()
            n710 = global write "Results_plotter_Global.vi" "X Axis Name"(w1473) -> ()
            n711 = Format Into String(format string="Add %s values", w1475) -> (resulting string=→"First Add label":string)  [unwired: 2 in, 1 out]
            n712 = Format Into String(format string="Add %s values", w1474) -> (resulting string=→"2nd Add label":string)  [unwired: 2 in, 1 out]
          }
          frame #11 {
            n713 = property on="Intensity Graph" class="IntGraph (strict)"() -> ("Color Table"=w1491:u32[])  [unwired: 2 in, 2 out]
            n714 = Increment(x="No of Contours") -> (x+1=w1492:i32)
            n715 = Divide(x=255, y=w1492) -> (x/y=w1496:dbl)
            n716 = To Long Integer(number=w1496) -> (32bit integer=w1495:i32)
            n717 = for {
              tunnel: w1495 -> [w1504]
              tunnel: [w1501] -> w1490 mode=indexing
              tunnel: w1491 -> [w1500] mode=indexing
              tunnel: u32 0 -> [w1499]
              i -> [w1505]
              n718 = Increment(x=w1505) -> (x+1=w1502:i32)
              n719 = Quotient & Remainder(x=w1502, y=w1504) -> (x-y*floor(x/y)=w1503:i32)  [unwired: 1 out]
              n720 = case shown="0" w1503 {
                tunnel: [w1506 w1507] -> w1501
                tunnel: w1500 -> [_ w1507]
                tunnel: w1499 -> [w1506 _]
                frame 0 {
                }
                frame 1, Default {
                }
              }
            }
            n721 = property on="Intensity Graph" class="IntGraph (strict)"("Ignore Array"=TRUE ("Write Attribute"), "Color Table"=w1490) -> ()  [unwired: 2 in, 2 out]
          }
          frame #12 {
            n722 = global read "Results_plotter_Global.vi" "Raw Interpolation"() -> (w1509:dbl[][])
            n723 = Add Array Elements(numeric array=w1509) -> (sum=w1508:dbl)
            n724 = Array Size(array=w1509) -> (size(s)=w1519:i32[])
            n725 = Decrement(x=w1519) -> (x-1=w1517:i32[])
            n726 = Index Array(array=w1517, index=0) -> (element=w1518:i32)
            n727 = Index Array(array=w1517, index=1) -> (element=w1514:i32)
            n728 = for {
              N: w1518 -> [_]
              tunnel: w1509 -> [w1527]
              tunnel: w1514 -> [w1526]
              shift-right: [w1522] -> w1511
              shift-left: 0.0 -> [w1523]
              shift-right: [w1521] -> w1510
              shift-left: 0 -> [w1520]
              i -> [w1525]
              n729 = Increment(x=w1525) -> (x+1=w1524:i32)
              n730 = for {
                N: w1526 -> [_]
                tunnel: w1527 -> [w1536]
                tunnel: w1525 -> [w1541]
                tunnel: w1524 -> [w1539]
                shift-right: [w1532] -> w1522
                shift-left: w1523 -> [w1531]
                shift-right: [w1528] -> w1521
                shift-left: w1520 -> [w1529]
                i -> [w1540]
                n731 = Increment(x=w1540) -> (x+1=w1538:i32)
                n732 = Index Array(array=w1536, index (row)=w1541, index (col)=w1538) -> (element=w1537:dbl)
                n733 = Index Array(array=w1536, index (row)=w1539, index (col)=w1538) -> (element=w1534:dbl)
                n734 = Index Array(array=w1536, index (row)=w1541, index (col)=w1540) -> (element=w1542:dbl)
                n735 = Index Array(array=w1536, index (row)=w1539, index (col)=w1540) -> (element=w1535:dbl)
                n736 = Compound Arithmetic op=ADD(w1542, w1537, w1535, w1534) -> (w1530:dbl)
                n737 = Not A Number/Path/Refnum?(number/path/refnum=w1530) -> (NaN/Path/Refnum?=w1533:bool)
                n738 = case shown="False" w1533 {
                  tunnel: [w1546 w1550] -> w1532
                  tunnel: w1531 -> [w1548 w1550]
                  tunnel: w1530 -> [w1547 _]
                  tunnel: [w1545 w1549] -> w1528
                  tunnel: w1529 -> [w1544 w1549]
                  frame False {
                    n739 = Add(x=w1547, y=w1548) -> (x+y=w1546:dbl)
                    n740 = Add(x=1, y=w1544) -> (x+y=w1545:i32)
                  }
                  frame True {
                  }
                }
              }
            }
          }
          frame #13 {
            n741 = local read "Resolution"() -> (w1563:dbl)
            n742 = Divide(x=w1561, y=4.0) -> (x/y=w1559:dbl)
            n743 = Multiply(x=w1563, y=w1563) -> (x*y=w1555:dbl)
            n744 = Multiply(x=w1555, y=w1554) -> ()  [unwired: 1 out]
            n745 = Multiply(x=w1555, y=w1562) -> (x*y=w1556:dbl)
            "Surface Area" <- w1556
            n746 = Multiply(x=w1555, y=w1559) -> (x*y=w1552:dbl)
            "Surface Integral" <- w1552
            n747 = global write "Results_plotter_Global.vi" "Surface Area"(w1556) -> ()
            n748 = global write "Results_plotter_Global.vi" "Surface Integral"(w1552) -> ()
            n749 = Divide(x=16666667, y=w1552) -> (x/y=→"Uadvec":dbl)
            n750 = Divide(x=w1552, y=w1556) -> (x/y=→"Surface Average":dbl)
          }
        }
      }
      frame "Analyse Plot Space" {
        n751 = case shown="True" "Show Plot Space Analysis" {
          tunnel: w1568 -> [_ w1578]
          tunnel: w1565 -> [_ w1577]
          frame False {
          }
          frame True {
            w1574 = TRUE  # Summarise All
            n752 = global read "Results_plotter_Global.vi" "Plot Index values"() -> (w1572:dbl[][])
            n753 = Index Array(array=w1572, index (row)=2) -> (element=w1571:dbl[])  [unwired: 1 in]
            n754 = To Long Integer(number=w1571) -> (32bit integer=w1570:i32[])
            n755 = for {
              tunnel: w1570 -> [w1581] mode=indexing
              tunnel: w1578 -> [w1580]
              tunnel: [w1579] -> w1575 mode=indexing
              n756 = Index Array(array=w1580, index (row)=w1581) -> (element=w1579:string[])  [unwired: 1 in]
            }
            n757 = call "Summarise.vi"("Channel Names"=w1577, "Data"=w1575, "Summarise All"=w1574) -> ("Summary"=w1576:string[][])  [unwired: 2 in]
            n758 = call "Plot_Space_Analysis.vi"("Table"=w1576) -> ()
          }
        }
      }
      frame "Vector Plot" {
        n759 = flat-sequence {
          tunnel: w1586 -> [w1591]
          tunnel: w1584 -> [w1590]
          frame #0 {
            n760 = local read "Job Directory"() -> (w1589:path)
            n761 = Build Path(base path=w1589, name or relative path="Vectors") -> (appended path=w1588:path)
            n762 = local read "Template"() -> (w1592:path)
            n763 = call "Vector_Plotting.vi"("JobVectorDirectory"=w1588, "Data"=w1590, "Template Filename"=w1592, "Channel Names"=w1591) -> ()  [unwired: 1 in]
          }
          frame #1 {
            n764 = local write "Vector Plot?"(FALSE ("Vector Plot?")) -> ()
          }
        }
      }
      frame "Coloured Dot Plot" {
        n765 = flat-sequence {
          tunnel: w1598 -> [w1603]
          tunnel: w1596 -> [w1602]
          frame #0 {
            n766 = local read "Job Directory"() -> (w1601:path)
            n767 = Build Path(base path=w1601, name or relative path="Dot_Plot") -> (appended path=w1600:path)
            n768 = local read "Template"() -> (w1604:path)
            n769 = call "Coloured_Dot_Plotting.vi"("JobVectorDirectory"=w1600, "Data"=w1602, "Template Filename"=w1604, "Channel Names"=w1603) -> ()  [unwired: 1 in]
          }
          frame #1 {
            n770 = local write "Dot Plot?"(FALSE ("Vector Plot?")) -> ()
          }
        }
      }
      frame "What to do next?" {
        n771 = property on="XY Plot" class="XYGraph (strict)"() -> ("YScale.Maximum"=w1607:dbl, "YScale.Minimum"=w1608:dbl, "XScale.Maximum"=w1609:dbl, "XScale.Minimum"=w1610:dbl)  [unwired: 2 in, 2 out]
        n772 = local read "Warning!"() -> (w1622:string)
        n773 = global write "Results_plotter_Global.vi" "First Loop"(FALSE) -> ()
        n774 = Empty String/Path?(string/path=w1622) -> (empty?=w1621:bool)
        n775 = Not(x=w1621) -> (.not. x?=w1620:bool)
        n776 = global write "Results_plotter_Global.vi" "Y plot min"(w1608) -> ()
        n777 = global write "Results_plotter_Global.vi" "Y plot max"(w1607) -> ()
        n778 = global write "Results_plotter_Global.vi" "X plot max"(w1609) -> ()
        n779 = global write "Results_plotter_Global.vi" "X plot min"(w1610) -> ()
        n780 = property on="Warning!" class="Str" props=["Visible", "Blinking", "Caption"]("Visible"=w1620, "Blinking"=w1620) -> ()  [unwired: 2 in, 3 out]
        n781 = case shown="False" "Add results file" {
          tunnel: [w1644 "More files options"] -> w1625
          tunnel: "Add results file" -> [_ _]
          tunnel: "Edit Template File" -> [w1635 _]
          frame False {
            n782 = Select(t="Edit template file", s=w1635, f="What to do next 2nd?") -> (s? t:f=w1633:string)
            n783 = Or(x="Save Plot data", y="Save Surface Fit") -> (x .or. y?=w1637:bool)
            n784 = Select(t="Save Plot Data", s=w1637, f=w1633) -> (s? t:f=w1640:string)
            n785 = Select(t="Create Plot summary", s="Save Plot as jpg", f=w1640) -> (s? t:f=w1631:string)
            n786 = Select(t="Save Data in Rows", s="Save Data in Rows", f=w1631) -> (s? t:f=w1644:string)
          }
          frame True {
            n787 = local write "Add results file"(FALSE) -> ()
          }
        }
        n788 = Select(t="End", s="stop", f=w1625) -> (s? t:f=w1616:string)
        n789 = Select(t="Vector Plot", s="Vector Plot?", f=w1616) -> (s? t:f=w1612:string)
        n790 = Select(t="Coloured Dot Plot", s="Dot Plot?", f=w1612) -> (s? t:f=w1611:string)
      }
      frame "What to do next 2nd?" {
        n791 = local read "Empty"() -> (w1668:bool)
        n792 = local read "Last used Template"() -> (w1656:path)
        n793 = local read "Template"() -> (w1648:path)
        n794 = Select(t="Empty Results file array", s=w1668, f="What to do next 3rd?") -> (s? t:f=w1651:string)
        n795 = global write "Results_plotter_Global.vi" "Template"(w1648) -> ()
        n796 = Not Equal?(x=w1656, y=w1648) -> (x != y?=w1655:bool)
        n797 = local read "Selected Row"() -> (w1647:i32)
        n798 = Select(t="What type of row averaging?", s="Save Averaged rows", f=w1651) -> (s? t:f=w1663:string)
        n799 = case shown="True" "Delete Plotted data from file" {
          tunnel: [w1698 "Full Res file manipulator" ("t")] -> w1661
          tunnel: w1663 -> [w1698 _]
          frame False {
          }
          frame True {
            n800 = local write "Plotted rows only?"(TRUE ("Save Plotted rows only?")) -> ()
            n801 = local write "Mode"(Plotter_Mode."Delete unwanted rows" ("Mode")) -> ()
          }
        }
        n802 = case shown="True" "Add /Edit metadata" {
          tunnel: [w1673 w1690] -> w1653
          tunnel: w1661 -> [w1674 w1691]
          tunnel: w1659 -> [_ w1689]
          tunnel: "Reload Files" -> [w1675 _]
          tunnel: [string[] [] ("New Chs Out") w1683] -> w1650
          tunnel: [string[][] [] w1682] -> w1649
          tunnel: w1647 -> [_ w1678]
          frame False {
            n803 = Select(t="Initialise", s=w1675, f=w1674) -> (s? t:f=w1673:string)
          }
          frame True {
            n804 = local read "Result files to read"() -> (w1684:path[])
            n805 = call "Edit_Channel_Panel.vi"("All Channel names"=w1689, "Result files to read"=w1684, "Selected Row"=w1678) -> ("New Values Out"=w1697:string[], "New Chs Out"=w1683:string[], "Cancel Out"=w1686:bool, "Edit Raw Data Header Info Out"=w1680:bool, "Plotted rows only?"=w1696:bool, "Selected Row?"=→"Selected Row?":bool, "Edit Raw data files?"=→"Edit Raw DF?":bool, "Raw data files in Orig Positions?"=→"Raw DF in Orig Pos?":bool, "Mode"=w1694:T4)  [unwired: 4 out]
            "Edit Raw Data Header Info" <- w1680
            n806 = Array Size(array=w1683) -> (size(s)=w1693:i32)
            n807 = Build Array(w1697) -> (w1682:string[][])
            n808 = local write "Add /Edit metadata"(FALSE ("Add /Edit metadata")) -> ()
            n809 = Greater Than 0?(x=w1693) -> (x > 0?=w1681:bool)
            n810 = local write "Plotted rows only?"(w1696) -> ()
            n811 = Or(x=w1680, y=w1681) -> (x .or. y?=w1679:bool)
            n812 = local write "Mode"(w1694) -> ()
            n813 = Compound Arithmetic op=AND(invert w1686, w1679) -> (w1685:bool)
            n814 = Select(t="Full Res file manipulator", s=w1685, f=w1691) -> (s? t:f=w1690:string)
          }
        }
        n815 = global write "Results_plotter_Global.vi" "New Chs In"(w1650) -> ()
        n816 = global write "Results_plotter_Global.vi" "New Values In"(w1649) -> ()
        n817 = Select(t="Initialise", s=w1655, f=w1653) -> (s? t:f=w1652:string)
      }
      frame "What to do next 3rd?" {
        n818 = local read "Show Results Space Analysis"() -> (w1719:bool)
        n819 = local read "Show Plot Space Analysis"() -> (w1718:bool)
        n820 = while {
          shift-right: [w1746] -> _
          shift-left: _ -> [w1745]
          shift-left: _ -> [w1744]
          shift-left: _ -> [w1743]
          tunnel: w1719 -> [w1746]
          shift-right: [w1751] -> _
          shift-left: _ -> [w1750]
          shift-left: _ -> [w1749]
          shift-left: _ -> [w1748]
          tunnel: w1718 -> [w1751]
          tunnel: [w1747] -> w1717
          tunnel: [w1742] -> w1716
          stop <- TRUE stop-if-true
          n821 = Compound Arithmetic op=AND(w1746, w1745, w1744, w1743) -> (w1742:bool)
          n822 = Compound Arithmetic op=AND(w1751, w1750, w1749, w1748) -> (w1747:bool)
        }
        n823 = local read "Index when last displayed"() -> (w1706:i32)
        n824 = local read "Index when last plotted"() -> (w1705:i32)
        n825 = global write "Results_plotter_Global.vi" "Plot EnFlo Tunnel Display"("Plot EnFlo Tunnel Display") -> ()
        n826 = Select(t="Run Calculation Routine", s="Calculate new metadata", f="What to do next 4th?") -> (s? t:f=w1725:string)
        n827 = case shown="True" w1717 {
          frame False {
          }
          frame True {
            n828 = Open VI Reference(vi path="Plot_Space_Analysis.vi" ("VI path")) -> (vi reference=w1763:refnum<vi>, error out=w1762:errorcluster)  [unwired: 1 in, 4 out]
            n829 = property class="VI"(reference=w1763, error in=w1762) -> (reference out=w1761:refnum<vi>, error out=w1760:errorcluster, "Front Panel Window:Open"=w1758:bool)
            n830 = local write "Show Plot Space Analysis"(w1758) -> ()
            n831 = Close Reference(reference=w1761, error in (no error)=w1760) -> ()  [unwired: 1 out]
          }
        }
        n832 = case shown="True" w1716 {
          frame False {
          }
          frame True {
            n833 = Open VI Reference(vi path="Results_Space_Analysis.vi" ("VI path")) -> (vi reference=w1757:refnum<vi>, error out=w1756:errorcluster)  [unwired: 1 in, 4 out]
            n834 = property class="VI"(reference=w1757, error in=w1756) -> (reference out=w1755:refnum<vi>, error out=w1754:errorcluster, "Front Panel Window:Open"=w1752:bool)
            n835 = local write "Show Results Space Analysis"(w1752) -> ()
            n836 = Close Reference(reference=w1755, error in (no error)=w1754) -> ()  [unwired: 1 out]
          }
        }
        n837 = Select(t="Save Setup", s="Save Setup", f=w1725) -> (s? t:f=w1722:string)
        n838 = Select(t="Choose Setup file", s="Load Setup", f=w1722) -> (s? t:f=w1715:string)
        n839 = Not Equal?(x=w1705, y=w1706) -> (x != y?=w1704:bool)
        n840 = And(x=w1704, y="Plot EnFlo Tunnel Display") -> (x .and. y?=w1703:bool)
        n841 = Or(x="Kill Point", y="Process Point") -> (x .or. y?=w1712:bool)
        n842 = Select(t="Process cursor point", s=w1712, f=w1715) -> (s? t:f=w1709:string)
        n843 = case shown="True" "Post Process Plotted Data" {
          tunnel: [w1737 "Full Res file manipulator" ("t")] -> w1708
          tunnel: w1709 -> [w1737 _]
          frame False {
          }
          frame True {
            n844 = local write "Plotted rows only?"(TRUE ("Plotted rows only?")) -> ()
            n845 = local write "Mode"(Plotter_Mode."Post Process Plotted Rows" ("Mode")) -> ()
          }
        }
        n846 = case shown="True" w1703 {
          tunnel: [w1733 "Full Res file manipulator" ("t")] -> w1707
          tunnel: w1708 -> [w1733 _]
          frame False {
          }
          frame True {
            n847 = local write "Plotted rows only?"(TRUE ("Plotted rows only?")) -> ()
            n848 = local write "Mode"(Plotter_Mode."Plot EnFlo Tunnel Display" ("Mode")) -> ()
          }
        }
      }
      frame "What to do next 4th?" {
        n849 = case shown="True" "Add Inlet Temperature offset" {
          tunnel: [w1771 "Full Res file manipulator" ("t")] -> w1765
          tunnel: "Time to save setup?" -> [w1771 _]
          frame False {
          }
          frame True {
            n850 = local write "Plotted rows only?"(TRUE ("Plotted rows only?")) -> ()
            n851 = local write "Mode"(Plotter_Mode."Add Inlet Temperature Offset" ("Mode")) -> ()
          }
        }
      }
      frame "Time to save setup?" {
        n852 = stacked-sequence {
          seq-local: [w1783 _] -> [_ w1823]
          seq-local: [w1782 _] -> [_ w1822]
          tunnel: [w1791 _] -> w1777
          tunnel: w1776 -> [w1781 _]
          frame #0 {
            n853 = while {
              shift-right: [w1812] -> _
              shift-left: _ -> [w1810]
              shift-right: [w1799] -> _
              shift-left: _ -> [w1807]
              tunnel: [w1799] -> w1790
              tunnel: [w1798] -> w1789
              shift-right: [w1800] -> _
              shift-left: _ -> [w1806]
              tunnel: [w1804] -> w1784
              tunnel: [w1801] -> w1785
              tunnel: [w1800] -> w1786
              tunnel: [w1797] -> w1782
              tunnel: w1781 -> [w1793]
              stop <- FALSE continue-if-true
              n854 = Get Date/Time In Seconds() -> (seconds since 1Jan1904=w1808:timestamp)
              n855 = To Double Precision Float(number=w1808) -> (double precision float=w1811:dbl)
              n856 = local read "Show Plot Space Analysis"() -> (w1800:bool)
              n857 = Subtract(x=w1811, y=w1810) -> (x-y=w1814:dbl)
              n858 = local read "Show Results Space Analysis"() -> (w1799:bool)
              n859 = Greater?(x=w1814, y=600.0) -> (0:w1795:bool)
              n860 = Greater?(x=w1793, y=300) -> (0:w1792:bool)
              n861 = And(x=w1795, y=w1792) -> (x .and. y?=w1794:bool)
              n862 = case shown="False" w1794 {
                tunnel: [w1815 w1821] -> w1812
                tunnel: w1811 -> [w1816 w1821]
                tunnel: w1810 -> [w1817 _]
                tunnel: ["Check modification dates?" "Save Setup"] -> w1803
                tunnel: w1792 -> [w1818 _]
                frame False {
                  n863 = Select(t=w1817, s=w1818, f=w1816) -> (s? t:f=w1815:dbl)
                }
                frame True {
                }
              }
              n864 = Not Equal?(x=w1800, y=w1806) -> (x != y?=w1801:bool)
              n865 = Not Equal?(x=w1799, y=w1807) -> (x != y?=w1798:bool)
              n866 = Compound Arithmetic op=AND(invert w1799, w1798) -> (w1797:bool)
              n867 = And(x=w1800, y=w1801) -> (x .and. y?=w1805:bool)
              n868 = Select(t="Analyse Plot Space", s=w1805, f=w1803) -> (s? t:f=w1804:string)
            }
            n869 = Compound Arithmetic op=AND(invert w1786, w1785) -> (w1783:bool)
            n870 = And(x=w1790, y=w1789) -> (x .and. y?=w1788:bool)
            n871 = Select(t="What is present?", s=w1788, f=w1784) -> (s? t:f=w1791:string)
          }
          frame #1 {
            n872 = case shown="True" w1822 {
              frame False {
              }
              frame True {
                n873 = Open VI Reference(vi path="Results_Space_Analysis.vi" ("VI path")) -> (vi reference=w1829:refnum<vi>, error out=w1828:errorcluster)  [unwired: 1 in, 4 out]
                n874 = property class="VI"(reference=w1829, error in=w1828, "Front Panel Window:Open"=FALSE) -> (reference out=w1827:refnum<vi>, error out=w1826:errorcluster)
                n875 = Close Reference(reference=w1827, error in (no error)=w1826) -> ()  [unwired: 1 out]
              }
            }
            n876 = case shown="True" w1823 {
              frame False {
              }
              frame True {
                n877 = Open VI Reference(vi path="Plot_Space_Analysis.vi" ("VI path")) -> (vi reference=w1835:refnum<vi>, error out=w1834:errorcluster)  [unwired: 1 in, 4 out]
                n878 = property class="VI"(reference=w1835, error in=w1834, "Front Panel Window:Open"=FALSE) -> (reference out=w1833:refnum<vi>, error out=w1832:errorcluster)
                n879 = Close Reference(reference=w1833, error in (no error)=w1832) -> ()  [unwired: 1 out]
              }
            }
          }
        }
      }
      frame "Check modification dates?" {
        n880 = while {
          shift-right: [w1854] -> _
          shift-left: _ -> [w1852]
          tunnel: [w1851] -> w1844
          stop <- FALSE continue-if-true
          n881 = Get Date/Time In Seconds() -> (seconds since 1Jan1904=w1849:timestamp)
          n882 = To Double Precision Float(number=w1849) -> (double precision float=w1853:dbl)
          n883 = Subtract(x=w1853, y=w1852) -> (x-y=w1857:dbl)
          n884 = Greater?(x=w1857, y=200.0) -> (0:w1855:bool)
          n885 = case shown="True" w1855 {
            tunnel: [w1859 w1862] -> w1854
            tunnel: w1853 -> [_ w1862]
            tunnel: w1852 -> [w1859 _]
            tunnel: [FALSE w1860] -> w1851
            frame False {
            }
            frame True {
              n886 = global read "Results_plotter_Global.vi" "First Loop"() -> (w1861:bool)
              n887 = Not(x=w1861) -> (.not. x?=w1860:bool)
            }
          }
        }
        n888 = Equal?(x="Tab Control", y=enum32{"Load ", "Plot ", "Save ", "Cursor"}."Cursor" ("Tab Control")) -> (x = y?=w1840:bool)
        n889 = Select(t="Read Cursor", s=w1840, f="Ordinate Selector Type") -> (s? t:f=w1838:string)
        n890 = Select(t="Files Modified?", s=w1844, f=w1838) -> (s? t:f=w1843:string)
      }
      frame "Files Modified?" {
        n891 = local read "nRows"() -> (w1866:i32)
        n892 = Less?(x=w1866, y=w1865) -> (x < y?=w1863:bool)
        n893 = case shown="True" w1863 {
          tunnel: [w1872 w1878] -> w1867
          tunnel: "Ordinate Selector Type" -> [w1872 w1873]
          frame False {
          }
          frame True {
            n894 = local read "Result files to read"() -> (w1877:path[])
            n895 = for {
              tunnel: w1877 -> [w1881] mode=indexing
              tunnel: [w1879] -> w1876 mode=indexing
              n896 = call "File_Modified_Since_Check.vi"("Pathname"=w1881, "Just Modified?"=TRUE) -> ("Modified?"=w1879:bool)
            }
            n897 = Or Array Elements(Boolean array=w1876) -> (logical OR=w1875:bool)
            n898 = Select(t="Initialise", s=w1875, f=w1873) -> (s? t:f=w1878:string)
          }
        }
      }
      frame "Read Cursor" {
        n899 = stacked-sequence {
          seq-local: [w1887 _] -> [_ w1922]
          tunnel: ["Ordinate Selector Type" _] -> w1885
          tunnel: [TRUE _] -> w1884
          tunnel: w1883 -> [_ w1921]
          tunnel: w1882 -> [_ w1920]
          frame #0 {
            n900 = property on="XY Plot" class="XYGraph (strict)"() -> ("Cursor.Cursor Position:Cursor X"=w1889:dbl, "Cursor.Cursor Position:Cursor Y"=w1888:dbl)  [unwired: 2 in, 2 out]
            n901 = local read "Transpose"() -> (w1902:bool)
            n902 = global read "Results_plotter_Global.vi" "Plot Index values"() -> (w1895:dbl[][])
            n903 = Index Array(array=w1895, index (row)=1) -> (element=w1893:dbl[])  [unwired: 1 in]
            n904 = Index Array(array=w1895, index (row)=2) -> (element=w1892:dbl[])  [unwired: 1 in]
            n905 = Index Array(array=w1895, index (row)=0) -> (element=w1894:dbl[])  [unwired: 1 in]
            n906 = case shown="True" w1902 {
              tunnel: [w1906 w1908] -> w1901
              tunnel: w1889 -> [w1906 w1907]
              tunnel: [w1905 w1907] -> w1900
              tunnel: w1888 -> [w1905 w1908]
              frame False {
              }
              frame True {
              }
            }
            n907 = for {
              tunnel: w1901 -> [w1917]
              tunnel: w1900 -> [w1916]
              tunnel: [w1911] -> w1899 mode=indexing
              tunnel: w1894 -> [w1910] mode=indexing
              tunnel: w1893 -> [w1909] mode=indexing
              n908 = Subtract(x=w1917, y=w1910) -> (x-y=w1915:dbl)
              n909 = Subtract(x=w1916, y=w1909) -> (x-y=w1914:dbl)
              n910 = Multiply(x=w1915, y=w1915) -> (x*y=w1912:dbl)
              n911 = Multiply(x=w1914, y=w1914) -> (x*y=w1913:dbl)
              n912 = Add(x=w1912, y=w1913) -> (x+y=w1911:dbl)
            }
            n913 = Array Max & Min(array=w1899) -> (min index (indices)=w1891:i32)  [unwired: 3 out]
            n914 = Index Array(array=w1892, index=w1891) -> (element=w1890:dbl)
            n915 = To Long Integer(number=w1890) -> (32bit integer=w1887:i32)
            "Cursor index" <- w1887
          }
          frame #1 {
            n916 = Index Array(array=w1921, index (row)=w1922) -> (element=w1919:string[])  [unwired: 1 in]
            n917 = for {
              tunnel: w1920 -> [w1930] mode=indexing
              tunnel: w1919 -> [w1923] mode=indexing
              tunnel: [w1929] -> w1918 mode=indexing
              n918 = while {
                shift-right: [w1942] -> _
                shift-left: w1923 -> [w1943]
                tunnel: [w1939] -> w1927
                tunnel: [w1938] -> w1925 mode=indexing
                i -> [w1939]
                stop <- w1940 continue-if-true
                n919 = Match Pattern(string=w1943, regular expression=":") -> (before substring=w1938:string, after substring=w1942:string, offset past match=w1941:i32)  [unwired: 2 out]
                n920 = Greater Than 0?(x=w1941) -> (x > 0?=w1940:bool)
              }
              n921 = Greater?(x=w1927, y=2) -> (0:w1926:bool)
              n922 = Reverse 1D Array(array=w1925) -> (reversed array=w1924:string[])
              n923 = case shown="True" w1926 {
                tunnel: w1930 -> [w1933 w1937]
                tunnel: [w1931 w1936] -> w1929
                tunnel: w1924 -> [_ w1935]
                tunnel: w1923 -> [w1932 w1934]
                frame False {
                  n924 = Build Array(w1933, w1932) -> (w1931:string[])
                }
                frame True {
                  n925 = Build Array (concatenate)(w1937, w1935, w1934) -> (w1936:string[])
                }
              }
            }
            "Table" <- w1918
          }
        }
      }
      frame "Process Cursor Point" {
        n926 = stacked-sequence {
          tunnel: [w1959] -> w1949
          tunnel: [TRUE] -> w1948
          tunnel: w1947 -> [_]
          tunnel: w1946 -> [_]
          tunnel: w1945 -> [w1960]
          frame #0 {
            n927 = local read "Kill Point"() -> (w1961:bool)
            n928 = global read "Results_plotter_Global.vi" "Row Reference"() -> (w1967:i32[][])
            n929 = local read "Cursor index"() -> (w1966:i32)
            n930 = Index Array(array=w1967, index (row)=w1966) -> (element=w1962:i32[])  [unwired: 1 in]
            n931 = local read "Result files to read"() -> (w1965:path[])
            n932 = Index Array(array=w1962, index #1=0 ("index"), index #2=1 ("index")) -> (element #1=w1964:i32, element #2=w1951:i32)
            "Selected Row" <- w1951
            n933 = Index Array(array=w1965, index=w1964) -> (element=w1958:path)
            n934 = call "GetRawDataFilePaths.vi"("Results file or Folder"=w1958) -> ("RawDataFilePaths"=w1957:string[], "RowNumbers"=w1953:i32[])  [unwired: 9 in]
            n935 = Search 1D Array(1D array=w1953, element=w1951) -> (index of element=w1952:i32)  [unwired: 1 in]
            n936 = Index Array(array=w1957, index=w1952) -> (element=w1956:string)
            n937 = call "String_to_Pathname.vi"("Input String"=w1956) -> ("path"=w1955:path)
            n938 = case shown="True" w1961 {
              tunnel: w1958 -> [_ w1989]
              tunnel: w1951 -> [_ w1985]
              tunnel: w1960 -> [_ w1992]
              tunnel: ["What to do next?" ("t") w1991] -> w1959
              tunnel: w1955 -> [w1969 w1983]
              frame False {
                n939 = disable-structure shown="Enabled" {
                  disable-tunnel: w1969 -> [_ w1981]
                  frame Disabled {
                    n940 = local read "Table"() -> (w1980:string[][])
                    n941 = Index Array(array=w1980, index (col) #1=1 ("disabled index (col)"), index (col) #2=0 ("index (col)")) -> (element #1=w1973:string[], element #2=w1972:string[])  [unwired: 2 in]
                    n942 = Search 1D Array(1D array=w1972, element="Raw Data Filename") -> (index of element=w1976:i32)  [unwired: 1 in]
                    n943 = Index Array(array=w1973, index=w1976) -> (element=w1975:string)
                    n944 = call "String_to_Pathname.vi"("Input String"=w1975) -> ("path"=w1974:path)
                    n945 = call "Post_Process_Measurement.vi"("Raw data file"=w1974) -> ()  [unwired: 1 out]
                  }
                  frame Enabled {
                    n946 = call "Post_Process_Measurement.vi"("Raw data file"=w1981) -> ()  [unwired: 1 out]
                  }
                }
                n947 = local write "Process Point"(FALSE ("Kill Point")) -> ()
              }
              frame True {
                n948 = Strip Path(path=w1989) -> (name=w1984:string)  [unwired: 1 out]
                n949 = Strip Path(path=w1983) -> (name=w1982:string)  [unwired: 1 out]
                n950 = local read "nRows"() -> (w1994:i32)
                n951 = Format Into String(format string="Are you sure you want to remove the row in the results file \"%s\" generated from the raw data filename \"%s\"?", w1984, w1982) -> (resulting string=w1987:string)  [unwired: 2 in, 1 out]
                n952 = Less?(x=w1994, y=w1992) -> (x < y?=w1993:bool)
                n953 = Two Button Dialog(message=w1987) -> (T button?=w1986:bool)  [unwired: 2 out]
                n954 = case shown="True" w1993 {
                  tunnel: ["Create Selectors" "Initialise" ("t")] -> w1991
                  frame False {
                  }
                  frame True {
                  }
                }
                n955 = case shown="True" w1986 {
                  tunnel: w1989 -> [_ w1996]
                  tunnel: w1985 -> [_ w1995]
                  frame False {
                  }
                  frame True {
                    n956 = Build Array(w1995) -> (w1997:i32[])
                    n957 = call "Delete_unwanted_rows.vi"("Selected Rows"=w1997, "Filename"=w1996) -> ()  [unwired: 1 out]
                  }
                }
                n958 = local write "Kill Point"(FALSE ("Kill Point")) -> ()
              }
            }
          }
        }
      }
      frame "Edit template file" {
        n959 = stacked-sequence {
          frame #0 {
            n960 = local read "Template"() -> (w2006:path)
            n961 = call "Valid_Path.vi"("Filename"=w2006) -> ("Valid Path?"=w2005:bool)
            n962 = case shown="False" w2005 {
              tunnel: [T8."Edit Existing Template File" ("Mode") T8."Create New Template File" ("Mode")] -> w2009
              frame True {
              }
              frame False {
              }
            }
            n963 = local read "Results file"() -> (w2008:path)
            n964 = call "Edit_Template_File.vi"("Mode"=w2009, "Template Filename"=w2006, "Data Filename"=w2008) -> ("Template Filename Out"=w2007:path)  [unwired: 12 out]
            n965 = local write "Template"(w2007) -> ()
          }
          frame #1 {
            n966 = local read "Job Directory"() -> (w2012:path)
            n967 = Path To String(path=w2012) -> (string=w2015:string)
            n968 = call "Read_Write_Template.vi"("Mode"=Global_mode."Write Global to File", "Single Value In"=w2015, "Data type"="Log Folder Name" ("Variable name")) -> ()  [unwired: 5 in, 8 out]
            n969 = local write "Edit Template File"(FALSE ("Edit Template File")) -> ()
            n970 = Current VI's Path() -> (path=w2018:path)
            n971 = call "Open_Close_Front_Panel.ph.vi"("Front Panel Window:Open"=TRUE, "VI path"=w2018) -> ()  [unwired: 2 out]
          }
        }
      }
      frame "Save Plot Data" {
        n972 = global read "Results_plotter_Global.vi" "XY Graph Cluster"() -> (w2019:cluster{dbl[], dbl[]}[])
        n973 = local read "Tolerances"() -> (w2026:dbl[])
        n974 = local read "Absisca"() -> (w2025:u16)
        n975 = local read "Transpose"() -> (w2024:bool)
        n976 = local read "Multi Ordinate"() -> (w2023:i32[])
        n977 = global read "Results_plotter_Global.vi" "Precision"() -> (w2020:string[])
        n978 = stacked-sequence {
          seq-local: [w2037 _ _ _ _ _ _ _ _] -> [_ w2062 _ w2100 _ _ _ _ _]
          seq-local: [_ w2058 _ _ _ _ _ _ _] -> [_ _ _ _ _ _ _ w2222 _]
          seq-local: [_ _ _ _ _ w2152 _ _ _] -> [_ _ _ _ _ _ _ w2221 _]
          seq-local: [_ _ _ _ _ w2154 _ _ _] -> [_ _ _ _ _ _ w2190 _ _]
          seq-local: [_ _ _ w2098 _ _ _ _ _] -> [_ _ _ _ _ _ w2191 _ _]
          seq-local: [_ _ _ _ w2121 _ _ _ _] -> [_ _ _ _ _ w2147 _ _ _]
          seq-local: [w2034 _ _ _ _ _ _ _ _] -> [_ _ _ _ _ _ _ _ w2227]
          seq-local: [w2033 _ _ _ _ _ _ _ _] -> [_ w2050 _ _ _ _ _ _ _]
          seq-local: [_ _ w2079 _ _ _ _ _ _] -> [_ _ _ w2099 _ _ w2192 _ _]
          seq-local: [_ _ _ _ _ _ w2188 _ _] -> [_ _ _ _ _ _ _ w2219 _]
          tunnel: [_ _ _ _ _ _ _ _ TRUE] -> w2032
          tunnel: [_ _ _ _ _ _ _ _ w2225] -> w2031
          tunnel: w2029 -> [_ _ _ _ _ w2150 _ _ _]
          tunnel: w2030 -> [_ w2055 _ _ _ w2153 _ _ _]
          tunnel: [_ _ _ _ _ w2153 _ _ _] -> w2028
          tunnel: [_ _ _ _ _ w2150 _ _ _] -> w2027
          tunnel: w2026 -> [w2039 _ _ _ w2126 w2151 _ _ _]
          tunnel: w2019 -> [w2038 _ _ w2102 _ _ _ _ _]
          tunnel: w2025 -> [w2036 w2072 _ _ w2128 _ _ _ _]
          tunnel: w2024 -> [w2035 _ _ w2101 _ _ _ _ _]
          tunnel: w2023 -> [_ _ _ _ w2125 _ _ _ _]
          tunnel: [_ _ _ w2096 _ _ _ _ _] -> w2022
          tunnel: w2021 -> [_ _ w2082 w2096 _ _ _ _ _]
          tunnel: w2020 -> [_ _ _ w2095 _ w2146 _ _ _]
          frame #0 {
            n979 = local read "Save Surface Fit"() -> (w2034:bool)
            n980 = Not(x=w2035) -> (.not. x?=w2042:bool)
            n981 = for {
              tunnel: w2038 -> [w2049] mode=indexing
              tunnel: w2042 -> [w2046]
              shift-right: [w2044] -> w2040
              shift-left: dbl[] [] -> [w2045]
              n982 = Unbundle(w2049) -> (w2048:dbl[], w2047:dbl[])
              n983 = Select(t=w2048, s=w2046, f=w2047) -> (s? t:f=w2043:dbl[])
              n984 = Build Array (concatenate)(w2045, w2043) -> (w2044:dbl[])
            }
            n985 = Index Array(array=w2039, index=w2036) -> (element=w2033:dbl)
            n986 = call "Numeric_bins.vi"("Values"=w2040, "Tolerance"=w2033) -> ("Bin Centres"=w2037:dbl[])  [unwired: 2 out]
          }
          frame #1 {
            n987 = Index Array(array=w2055, index=w2072) -> (element=w2075:string)
            n988 = Match Pattern(string=w2075, regular expression=":") -> (before substring=w2074:string, after substring=w2073:string)  [unwired: 3 out]
            n989 = Concatenate Strings(w2074, " ", w2073, " =:" ("regular expression")) -> (w2057:string)
            n990 = Greater?(x=w2050, y=0.4) -> (0:w2070:bool)
            n991 = Greater?(x=w2050, y=0.09) -> (0:w2065:bool)
            n992 = call <vilib>:"Trim Whitespace.vi"("string"=w2057) -> ("trimmed string"=w2056:string)  [unwired: 1 in]
            n993 = Select(t=i16 0 ("precision (6)"), s=w2070, f=i16 2 ("precision (6)")) -> (s? t:f=w2066:i16)
            n994 = Select(t=w2066, s=w2065, f=i16 3) -> (s? t:f=w2063:i16)
            n995 = Number To Fractional String(number=w2062, precision (6)=w2063) -> (F-format string=w2061:string[])  [unwired: 2 out]
            n996 = for {
              tunnel: w2056 -> [w2078]
              tunnel: w2061 -> [w2076] mode=indexing
              tunnel: [w2077] -> w2060 mode=indexing
              n997 = Concatenate Strings(w2078, w2076) -> (w2077:string)
            }
            n998 = Build Array (concatenate)("Plot:Legend:" ("Input Element"), w2060, "End of:Plot Series:" ("Input Element")) -> (w2058:string[])
          }
          frame #2 {
            n999 = local read "Multi Ordinate?"() -> (w2081:bool)
            n1000 = global read "Results_plotter_Global.vi" "Legend"() -> (w2080:string[])
            n1001 = case shown="False" w2081 {
              tunnel: w2082 -> [w2086 _]
              tunnel: [w2083 w2094] -> w2079
              tunnel: w2080 -> [w2085 w2094]
              frame False {
                n1002 = local read "Multi Ordinate"() -> (w2089:i32[])
                n1003 = Index Array(array=w2089, index=0 ("Index")) -> (element=w2087:i32)
                n1004 = Index Array(array=w2086, index=w2087) -> (element=w2084:string)
                n1005 = for {
                  tunnel: w2085 -> [w2093] mode=indexing
                  tunnel: w2084 -> [w2092]
                  tunnel: [w2090] -> w2083 mode=indexing
                  n1006 = Format Into String(format string="; %s", initial string=w2092, w2093) -> (resulting string=w2090:string)  [unwired: 1 in, 1 out]
                }
              }
              frame True {
              }
            }
          }
          frame #3 {
            n1007 = call "Grid_Data.vi"("Transpose"=w2101, "XY Graph"=w2102, "Bin Centres"=w2100) -> ("Grided data"=w2097:dbl[][])  [unwired: 1 out]
            n1008 = for {
              tunnel: w2099 -> [w2109] mode=indexing
              tunnel: [w2111] -> w2098 mode=indexing
              tunnel: w2097 -> [w2110] mode=indexing
              tunnel: w2096 -> [w2105]
              tunnel: w2095 -> [w2104]
              n1009 = Match Pattern(string=w2109, regular expression=";") -> (before substring=w2106:string)  [unwired: 4 out]
              n1010 = Search 1D Array(1D array=w2105, element=w2106) -> (index of element=w2107:i32)  [unwired: 1 out]
              n1011 = Index Array(array=w2104, index=w2107) -> (element=w2103:string)
              n1012 = for {
                tunnel: w2103 -> [w2116]
                tunnel: [w2115] -> w2112 mode=indexing
                tunnel: w2110 -> [w2113] mode=indexing
                n1013 = Not A Number/Path/Refnum?(number/path/refnum=w2113) -> (NaN/Path/Refnum?=w2114:bool)
                n1014 = case shown="True" w2114 {
                  tunnel: w2116 -> [w2119 _]
                  tunnel: [w2118 ""] -> w2115
                  tunnel: w2113 -> [w2117 _]
                  frame False {
                    n1015 = call "Number_2_string.vi"("precision"=w2119, "number"=w2117) -> ("String"=w2118:string)
                  }
                  frame True {
                  }
                }
              }
              n1016 = Build Array (concatenate)(w2109, w2112) -> (w2111:string[])
            }
          }
          frame #4 {
            n1017 = Index Array(array=w2125, index=0 ("Index")) -> (element=w2123:i32)
            n1018 = global read "Results_plotter_Global.vi" "Summarise"() -> (w2122:string[])
            n1019 = for {
              shift-right: [w2135] -> w2121
              shift-left: i32[] [] -> [w2136]
              tunnel: w2128 -> [w2141]
              tunnel: w2123 -> [w2140]
              tunnel: w2126 -> [w2133] mode=indexing
              tunnel: w2122 -> [w2131] mode=indexing
              i -> [w2134]
              n1020 = Equal?(x=w2140, y=w2134) -> (x = y?=w2139:bool)
              n1021 = Not A Number/Path/Refnum?(number/path/refnum=w2133) -> (NaN/Path/Refnum?=w2132:bool)
              n1022 = Equal?(x=w2141, y=w2134) -> (x = y?=w2138:bool)
              n1023 = Equal?(x="FALSE", y=w2131) -> (x = y?=w2129:bool)
              n1024 = Compound Arithmetic op=OR(w2138, w2139, w2132, w2129) -> (w2137:bool)
              n1025 = case shown="False" w2137 {
                tunnel: w2136 -> [w2144 w2145]
                tunnel: [w2143 w2145] -> w2135
                tunnel: w2134 -> [w2142 _]
                frame False {
                  n1026 = Build Array (concatenate)(w2144, w2142) -> (w2143:i32[])
                }
                frame True {
                }
              }
            }
          }
          frame #5 {
            n1027 = local read "Plotted Series"() -> (w2149:bool[][])
            n1028 = for {
              tunnel: w2151 -> [w2165]
              tunnel: [w2164] -> w2154 mode=indexing
              tunnel: w2147 -> [w2163]
              tunnel: w2150 -> [w2162]
              tunnel: w2149 -> [w2161] mode=indexing
              tunnel: i32[] [] -> [w2159]
              tunnel: w2146 -> [w2158]
              n1029 = for {
                shift-right: [w2167] -> w2160
                shift-left: w2159 -> [w2168]
                tunnel: w2161 -> [w2166] mode=indexing
                i -> [w2169]
                n1030 = case shown="True" w2166 {
                  tunnel: w2169 -> [_ w2173]
                  tunnel: w2168 -> [w2170 w2172]
                  tunnel: [w2170 w2171] -> w2167
                  frame False {
                  }
                  frame True {
                    n1031 = Build Array (concatenate)(w2172, w2173) -> (w2171:i32[])
                  }
                }
              }
              n1032 = for {
                tunnel: w2165 -> [w2181]
                tunnel: [w2182] -> w2164 mode=indexing
                tunnel: w2163 -> [w2176] mode=indexing
                tunnel: w2162 -> [w2179]
                tunnel: w2160 -> [w2178]
                tunnel: w2158 -> [w2175]
                n1033 = for {
                  tunnel: w2178 -> [w2187] mode=indexing
                  tunnel: [w2186] -> w2183 mode=indexing
                  tunnel: w2176 -> [w2185]
                  tunnel: w2179 -> [w2184]
                  n1034 = Index Array(array=w2184, index (row)=w2187, index (col)=w2185) -> (element=w2186:string)
                }
                n1035 = Index Array(array=w2175, index=w2176) -> (element=w2177:string)
                n1036 = Index Array(array=w2181, index=w2176) -> (element=w2180:dbl)
                n1037 = call "Value_Occurence_Analysis.vi"("Average Numeric Values?"=FALSE, "Tolerance"=w2180, "Precision (3)"=w2177, "String Array"=w2183) -> ("Output String"=w2182:string)  [unwired: 2 out]
              }
            }
            n1038 = for {
              tunnel: w2147 -> [w2157] mode=indexing
              tunnel: w2153 -> [w2156]
              tunnel: [w2155] -> w2152 mode=indexing
              n1039 = Index Array(array=w2156, index=w2157) -> (element=w2155:string)
            }
          }
          frame #6 {
            n1040 = for {
              shift-right: [w2205] -> w2188
              shift-left: string[][] [] -> [w2206]
              shift-right: [w2201] -> _
              shift-left: _ -> [w2202]
              tunnel: w2192 -> [w2203] mode=indexing
              tunnel: w2191 -> [w2195] mode=indexing
              tunnel: w2190 -> [w2194] mode=indexing
              i -> [w2200]
              n1041 = Greater Than 0?(x=w2200) -> (x > 0?=w2199:bool)
              n1042 = Match Pattern(string=w2203, regular expression="; ") -> (before substring=w2201:string)  [unwired: 4 out]
              n1043 = Equal?(x=w2202, y=w2201) -> (x = y?=w2198:bool)
              n1044 = Build Array (concatenate)(w2195, "", w2194) -> (w2193:string[])
              n1045 = Compound Arithmetic op=AND(w2199, invert w2198) -> (w2197:bool)
              n1046 = case shown="True" w2197 {
                tunnel: w2206 -> [w2210 w2213]
                tunnel: [w2209 w2212] -> w2205
                tunnel: w2193 -> [w2208 w2211]
                frame True {
                  n1047 = Build Array (concatenate)(w2210, string[] [] ("array"), w2208) -> (w2209:string[][])
                }
                frame False {
                  n1048 = Build Array (concatenate)(w2213, w2211) -> (w2212:string[][])
                }
              }
            }
          }
          frame #7 {
            w2218 = TRUE  # Simple Save?
            n1049 = Build Array (concatenate)(w2222, w2221) -> (w2220:string[])
            n1050 = local read "Header"() -> (w2215:string)
            n1051 = call "Write_output_file.vi"("Output filename"="Output Filename", "Header"=w2215, "Channel Names"=w2220, "Data"=w2219, "Simple Save?"=w2218, "Summarise mode"=T9."No data summary") -> ("Output filename Out"=w2216:path)  [unwired: 6 in, 3 out]
            n1052 = local write "Output Filename"(w2216) -> ()
          }
          frame #8 {
            n1053 = local write "Save Plot data"(FALSE ("Save Plot data")) -> ()
            n1054 = local write "Header"("") -> ()
            n1055 = Select(t="Save Surface Fit data", s=w2227, f="Create Selectors") -> (s? t:f=w2225:string)
          }
        }
      }
      frame "What type of row averaging?" {
        n1056 = Two Button Dialog(message="Do you want to Combine rows with identical positions together?", 1:"Just average series" ("F button name (\"Cancel\")"), 2:"Combine rows" ("T button name (\"OK\")")) -> (T button?=w2233:bool)
        n1057 = Select(t="Combine rows" ("T button name (\"OK\")"), s=w2233, f="Average Rows together") -> (s? t:f=w2230:string)
      }
      frame "Combine rows" {
        w2243 = TRUE  # Show panel ?
        n1058 = local read "Output Filename"() -> (w2242:path)
        n1059 = call "Combined_file_Panel.vi"("Show panel ?"=w2243, "Output filename"=w2242) -> ("Only Plotted data?"=w2244:bool, "Include Empty Rows? Out"=w2245:bool, "Give Audit Channels Out"=w2246:bool, "Output filename Out"=w2241:path)  [unwired: 5 out]
        n1060 = case shown="True" w2244 {
          tunnel: w2248 -> [w2257 w2260]
          tunnel: [w2257 w2258] -> w2247
          frame False {
          }
          frame True {
            n1061 = global read "Results_plotter_Global.vi" "Plot Index values"() -> (w2262:dbl[][])
            n1062 = Index Array(array=w2262, index (row)=2) -> (element=w2259:dbl[])  [unwired: 1 in]
            n1063 = for {
              tunnel: w2260 -> [w2265]
              tunnel: w2259 -> [w2264] mode=indexing
              tunnel: [w2263] -> w2258 mode=indexing
              n1064 = Index Array(array=w2265, index (row)=w2264) -> (element=w2263:string[])  [unwired: 1 in]
            }
          }
        }
        n1065 = local write "Save Averaged rows"(FALSE ("Save Plot data")) -> ()
        n1066 = local read "X Ch Name"() -> (w2252:u16)
        n1067 = local read "Y Ch Name"() -> (w2253:u16)
        n1068 = local read "Z Ch Name"() -> (w2254:u16)
        n1069 = call "Find_Rows_to_Combine.vi"("Include Empty Rows?"=w2245, "file path (dialog if empty)"=w2241, "Give Audit Channels"=w2246, "Full Channel Names"=w2251, "Data"=w2247, "Z Column Index"=w2254, "Y Column Index"=w2253, "X Column Index"=w2252) -> ()  [unwired: 4 out]
        n1070 = local write "Output Filename"(w2241) -> ()
      }
      frame "Average Rows together" {
        n1071 = local read "Output Filename"() -> (w2267:path)
        n1072 = global read "Results_plotter_Global.vi" "XY Graph Cluster"() -> (w2269:cluster{dbl[], dbl[]}[])
        n1073 = call "Does_file_exist_(simple).vi"("Pathname"=w2267) -> ("exists?"=w2266:bool)
        n1074 = local read "Tolerances"() -> (w2275:dbl[])
        n1075 = local read "Absisca"() -> (w2274:u16)
        n1076 = local read "Transpose"() -> (w2273:bool)
        n1077 = global read "Results_plotter_Global.vi" "Precision"() -> (w2271:string[])
        n1078 = global read "Results_plotter_Global.vi" "Summarise"() -> (w2270:string[])
        n1079 = stacked-sequence {
          seq-local: [w2287 _ _ _ _] -> [_ w2304 _ _ _]
          seq-local: [_ w2307 _ _ _] -> [_ _ _ w2385 _]
          seq-local: [w2283 _ _ _ _] -> [_ w2305 _ _ _]
          seq-local: [_ _ w2367 _ _] -> [_ _ _ w2384 _]
          tunnel: [_ _ _ _ TRUE] -> w2281
          tunnel: [_ _ _ _ "Create Selectors"] -> w2280
          tunnel: w2278 -> [_ w2310 _ _ w2410]
          tunnel: w2279 -> [_ _ w2368 _ w2409]
          tunnel: [_ _ _ _ w2409] -> w2277
          tunnel: [_ _ _ _ w2410] -> w2276
          tunnel: w2275 -> [w2289 w2308 _ _ _]
          tunnel: w2269 -> [w2288 _ _ _ _]
          tunnel: w2274 -> [w2286 _ _ _ _]
          tunnel: w2273 -> [w2285 _ _ _ _]
          tunnel: w2272 -> [w2282 _ _ _ _]
          tunnel: w2271 -> [_ w2309 _ _ _]
          tunnel: w2270 -> [_ w2306 w2369 _ _]
          tunnel: [w2282 _ _ _ _] -> w2268
          tunnel: w2267 -> [_ _ _ w2383 _]
          tunnel: w2266 -> [_ _ _ w2382 _]
          frame #0 {
            n1080 = Not(x=w2285) -> (.not. x?=w2292:bool)
            n1081 = for {
              tunnel: w2288 -> [w2299] mode=indexing
              tunnel: w2292 -> [w2296]
              shift-right: [w2294] -> w2290
              shift-left: dbl[] [] -> [w2295]
              n1082 = Unbundle(w2299) -> (w2298:dbl[], w2297:dbl[])
              n1083 = Select(t=w2298, s=w2296, f=w2297) -> (s? t:f=w2293:dbl[])
              n1084 = Build Array (concatenate)(w2295, w2293) -> (w2294:dbl[])
            }
            n1085 = Index Array(array=w2289, index=w2286) -> (element=w2284:dbl)
            n1086 = call "Numeric_bins.vi"("Values"=w2290, "Tolerance"=w2284) -> ("Bin Centres"=w2287:dbl[], "Bin Index"=w2283:i32[])  [unwired: 1 out]
          }
          frame #1 {
            n1087 = Array Size(array=w2304) -> (size(s)=w2303:i32)
            n1088 = global read "Results_plotter_Global.vi" "Plot Index values"() -> (w2301:dbl[][])
            n1089 = Index Array(array=w2301, index (row)=2) -> (element=w2300:dbl[])  [unwired: 1 in]
            n1090 = for {
              N: w2303 -> [_]
              tunnel: w2310 -> [w2320]
              tunnel: w2309 -> [w2319]
              tunnel: w2308 -> [w2318]
              tunnel: [w2311] -> w2307 mode=indexing
              tunnel: w2306 -> [w2317]
              tunnel: w2305 -> [w2315]
              tunnel: w2300 -> [w2314]
              i -> [w2316]
              n1091 = stacked-sequence {
                seq-local: [w2324 _] -> [_ w2343]
                tunnel: w2320 -> [_ w2344]
                tunnel: w2319 -> [_ w2342]
                tunnel: w2318 -> [_ w2341]
                tunnel: w2317 -> [_ w2340]
                tunnel: w2316 -> [w2323 _]
                tunnel: w2315 -> [w2322 _]
                tunnel: w2314 -> [w2321 _]
                tunnel: [_ w2338] -> w2313
                tunnel: [_ w2337] -> w2312
                frame #0 {
                  n1092 = for {
                    shift-right: [w2330] -> w2324
                    shift-left: i32[] [] -> [w2331]
                    tunnel: w2323 -> [w2329]
                    tunnel: w2322 -> [w2328] mode=indexing
                    tunnel: w2321 -> [w2326] mode=indexing
                    n1093 = Equal?(x=w2328, y=w2329) -> (x = y?=w2327:bool)
                    n1094 = case shown="False" w2327 {
                      tunnel: w2331 -> [w2332 w2335]
                      tunnel: [w2332 w2336] -> w2330
                      tunnel: w2326 -> [_ w2333]
                      frame False {
                      }
                      frame True {
                        n1095 = To Long Integer(number=w2333) -> (32bit integer=w2334:i32)
                        n1096 = Build Array (concatenate)(w2335, w2334) -> (w2336:i32[])
                      }
                    }
                  }
                }
                frame #1 {
                  n1097 = for {
                    tunnel: w2344 -> [w2358]
                    tunnel: w2343 -> [w2357]
                    tunnel: w2342 -> [w2355] mode=indexing
                    tunnel: w2341 -> [w2354] mode=indexing
                    tunnel: [w2353] -> w2338 mode=indexing
                    tunnel: w2340 -> [w2350] mode=indexing
                    shift-right: [w2345] -> w2337
                    shift-left: string[] [] -> [w2346]
                    i -> [w2352]
                    n1098 = for {
                      tunnel: w2358 -> [w2366]
                      tunnel: w2357 -> [w2365] mode=indexing
                      tunnel: [w2364] -> w2356 mode=indexing
                      tunnel: w2352 -> [w2363]
                      n1099 = Index Array(array=w2366, index (row)=w2365, index (col)=w2363) -> (element=w2364:string)
                    }
                    n1100 = Equal?(x="TRUE", y=w2350) -> (x = y?=w2349:bool)
                    n1101 = Not(x=w2349) -> (.not. x?=w2348:bool)
                    n1102 = call "Value_Occurence_Analysis.vi"("Average Numeric Values?"=w2348, "Tolerance"=w2354, "Precision (3)"=w2355, "String Array"=w2356) -> ("St Dev"=w2347:string, "Output String"=w2353:string)  [unwired: 1 out]
                    n1103 = case shown="False" w2348 {
                      tunnel: w2347 -> [_ w2362]
                      tunnel: w2346 -> [w2359 w2361]
                      tunnel: [w2359 w2360] -> w2345
                      frame False {
                      }
                      frame True {
                        n1104 = Build Array (concatenate)(w2361, w2362) -> (w2360:string[])
                      }
                    }
                  }
                }
              }
              n1105 = Build Array (concatenate)(w2313, w2312) -> (w2311:string[])
            }
          }
          frame #2 {
            n1106 = for {
              tunnel: w2369 -> [w2374] mode=indexing
              shift-right: [w2370] -> w2367
              shift-left: w2368 -> [w2371]
              tunnel: w2368 -> [w2372] mode=indexing
              n1107 = Equal?(x="TRUE", y=w2374) -> (x = y?=w2373:bool)
              n1108 = case shown="False" w2373 {
                tunnel: w2372 -> [w2380 _]
                tunnel: w2371 -> [w2377 w2381]
                tunnel: [w2376 w2381] -> w2370
                frame False {
                  n1109 = Concatenate Strings(w2380, "St Dev") -> (w2378:string)
                  n1110 = Build Array (concatenate)(w2377, w2378) -> (w2376:string[])
                }
                frame True {
                }
              }
            }
          }
          frame #3 {
            n1111 = case shown="False" w2382 {
              tunnel: w2385 -> [w2388 w2396]
              tunnel: w2384 -> [w2391 w2397]
              tunnel: w2383 -> [w2389 w2398]
              frame False {
                w2392 = FALSE  # Save Plotted rows only?
                w2394 = TRUE  # Simple Save?
                n1112 = Build Array (concatenate)(string[] [] ("array"), w2388) -> (w2387:string[][])
                n1113 = local read "Template"() -> (w2393:path)
                n1114 = call "Write_output_file.vi"("Output filename"=w2389, "Template Filename"=w2393, "Channel Names"=w2391, "Data"=w2387, "Simple Save?"=w2394, "Save Plotted rows only?"=w2392, "Summarise mode"=T9."No data summary") -> ("Output filename Out"=w2395:path)  [unwired: 5 in, 3 out]
                n1115 = local write "Output Filename"(w2395) -> ()
              }
              frame True {
                w2401 = FALSE  # Present Channels only
                w2403 = TRUE  # exists?
                n1116 = call "Check_and_rewrite_file.vi"("Filename"=w2398, "Present Channels only"=w2401, "Present Channels"=w2397) -> ("Merged Channels"=w2402:string[], "Merged?"=w2400:bool)  [unwired: 1 in, 10 out]
                n1117 = case shown="True" w2400 {
                  tunnel: w2396 -> [w2404 w2406]
                  tunnel: w2397 -> [_ w2407]
                  tunnel: [w2404 w2405] -> w2399
                  tunnel: w2402 -> [_ w2408]
                  frame False {
                  }
                  frame True {
                    n1118 = call "Merge_2D_values.vi"("Values In"=w2406, "Present Channels"=w2407, "Desired Channels"=w2408) -> ("Values Out"=w2405:string[][])
                  }
                }
                n1119 = call "Write_Ch_data_file.vi"("exists?"=w2403, "Channel Values"=w2399, "Channel names"=w2402, "Filename"=w2398) -> ()  [unwired: 4 in, 4 out]
              }
            }
          }
          frame #4 {
            n1120 = local write "Save Averaged rows"(FALSE ("Save Plot data")) -> ()
          }
        }
      }
      frame "Save Surface Fit data" {
        n1121 = local read "Transpose"() -> (w2414:bool)
        n1122 = local read "Tolerances"() -> (w2421:dbl[])
        n1123 = local read "Absisca"() -> (w2420:u16)
        n1124 = global read "Results_plotter_Global.vi" "Precision"() -> (w2417:string[])
        n1125 = stacked-sequence {
          seq-local: [w2428 _ _ _ _ _] -> [_ w2447 _ _ _ _]
          seq-local: [_ w2444 _ _ _ _] -> [_ _ _ _ w2531 _]
          seq-local: [_ _ w2470 _ _ _] -> [_ _ _ _ w2550 _]
          seq-local: [w2429 _ _ _ _ _] -> [_ _ w2471 _ _ _]
          seq-local: [_ _ w2466 _ _ _] -> [_ _ _ _ w2534 _]
          seq-local: [_ _ w2465 _ _ _] -> [_ _ _ w2501 _ _]
          seq-local: [_ _ _ w2496 _ _] -> [_ _ _ _ w2532 _]
          tunnel: [_ _ _ _ _ TRUE] -> w2425
          tunnel: [_ _ _ _ _ "Create Selectors"] -> w2424
          tunnel: w2422 -> [_ _ _ _ _ w2556]
          tunnel: w2423 -> [_ w2432 _ _ _ w2557]
          tunnel: w2421 -> [_ w2458 _ _ _ _]
          tunnel: w2420 -> [_ w2459 _ _ _ _]
          tunnel: [_ _ w2476 _ _ _] -> w2419
          tunnel: w2418 -> [_ w2435 w2476 _ _ _]
          tunnel: w2417 -> [_ _ w2472 _ _ _]
          tunnel: [_ _ _ _ _ w2557] -> w2416
          tunnel: [_ _ _ _ _ w2556] -> w2415
          tunnel: w2414 -> [_ _ _ w2495 _ _]
          frame #0 {
            n1126 = global read "Results_plotter_Global.vi" "X Values"() -> (w2428:dbl[])
            n1127 = global read "Results_plotter_Global.vi" "Raw Interpolation"() -> (w2426:dbl[][])
            n1128 = global read "Results_plotter_Global.vi" "Y Values"() -> (w2427:dbl[])
            n1129 = Insert Into Array(array=w2426, index (col)=0 ("disabled index (col)"), new element=w2427) -> (w2429:dbl[][])  [unwired: 1 in]
          }
          frame #1 {
            n1130 = global read "Results_plotter_Global.vi" "Y Axis Name"() -> (w2434:string)
            n1131 = Search 1D Array(1D array=w2435, element=w2434) -> (index of element=w2433:i32)  [unwired: 1 out]
            n1132 = Index Array(array=w2432, index=w2433) -> (element=w2431:string)
            n1133 = Match Pattern(string=w2431, regular expression=":") -> (before substring=w2461:string, after substring=w2460:string)  [unwired: 3 out]
            n1134 = Index Array(array=w2458, index=w2459) -> (element=w2449:dbl)
            n1135 = Concatenate Strings(w2461, " ", w2460, " =:" ("regular expression")) -> (w2443:string)
            n1136 = Greater?(x=w2449, y=0.9) -> (0:w2456:bool)
            n1137 = Greater?(x=w2449, y=0.09) -> (0:w2451:bool)
            n1138 = call <vilib>:"Trim Whitespace.vi"("string"=w2443) -> ("trimmed string"=w2442:string)  [unwired: 1 in]
            n1139 = Select(t=i16 0 ("precision (6)"), s=w2456, f=i16 2 ("precision (6)")) -> (s? t:f=w2452:i16)
            n1140 = Select(t=w2452, s=w2451, f=i16 3) -> (s? t:f=w2448:i16)
            n1141 = Number To Fractional String(number=w2447, precision (6)=w2448) -> (F-format string=w2446:string[])  [unwired: 2 out]
            n1142 = for {
              tunnel: w2442 -> [w2464]
              tunnel: w2446 -> [w2462] mode=indexing
              tunnel: [w2463] -> w2437 mode=indexing
              n1143 = Concatenate Strings(w2464, w2462) -> (w2463:string)
            }
            n1144 = Build Array (concatenate)("Channel:Values:Plotted" ("Input Element"), "Axis:Name:" ("Input Element"), "Axis:Values:" ("Input Element"), w2437) -> (w2444:string[])
          }
          frame #2 {
            n1145 = global read "Results_plotter_Global.vi" "X Axis Name"() -> (w2469:string)
            n1146 = Concatenate Strings(w2469, " =" ("string")) -> (w2467:string)
            n1147 = local read "Multi Ordinate"() -> (w2475:i32[])
            n1148 = Index Array(array=w2475, index=0 ("Index")) -> (element=w2473:i32)
            n1149 = Index Array(array=w2472, index=w2473) -> (element=w2465:string)
            n1150 = Index Array(array=w2476, index=w2473) -> (element=w2466:string)
            n1151 = for {
              tunnel: w2466 -> [w2478]
              tunnel: [w2481] -> w2470 mode=indexing
              tunnel: w2465 -> [w2480]
              tunnel: w2471 -> [w2479] mode=indexing
              tunnel: w2467 -> [w2477]
              n1152 = for {
                tunnel: w2479 -> [w2484] mode=indexing
                tunnel: [w2483] -> w2482 mode=indexing
                tunnel: w2480 -> [w2486]
                n1153 = Not A Number/Path/Refnum?(number/path/refnum=w2484) -> (NaN/Path/Refnum?=w2485:bool)
                n1154 = case shown="False" w2485 {
                  tunnel: w2486 -> [w2489 _]
                  tunnel: w2484 -> [w2488 _]
                  tunnel: [w2487 ""] -> w2483
                  frame False {
                    n1155 = call "Number_2_string.vi"("precision"=w2489, "number"=w2488) -> ("String"=w2487:string)
                  }
                  frame True {
                  }
                }
              }
              n1156 = Build Array (concatenate)(w2478, w2477, w2482) -> (w2481:string[])
            }
          }
          frame #3 {
            w2500 = "\t"
            n1157 = global read "Results_plotter_Global.vi" "Intensity Plot data in rows"() -> (w2502:dbl[][])
            n1158 = global read "Results_plotter_Global.vi" "Value plotted Name"() -> (w2499:string)
            n1159 = global read "Results_plotter_Global.vi" "X Axis Name"() -> (w2493:string)
            n1160 = global read "Results_plotter_Global.vi" "Y Axis Name"() -> (w2492:string)
            n1161 = case shown="False" w2495 {
              tunnel: [w2503 w2506] -> w2494
              tunnel: w2493 -> [w2504 w2506]
              tunnel: w2492 -> [w2503 w2505]
              tunnel: [w2504 w2505] -> w2491
              frame False {
              }
              frame True {
              }
            }
            n1162 = Concatenate Strings(w2494, w2500, w2491, w2500, w2499, "\r\n") -> (w2497:string)
            n1163 = for {
              tunnel: w2502 -> [w2512] mode=indexing
              tunnel: w2501 -> [w2517]
              shift-right: [w2511] -> w2496
              shift-left: w2497 -> [w2516]
              n1164 = Index Array(array=w2512, index=0) -> (element=w2508:dbl)
              n1165 = Index Array(array=w2512, index=1) -> (element=w2507:dbl)
              n1166 = Index Array(array=w2512, index=2) -> (element=w2510:dbl)
              n1167 = Not A Number/Path/Refnum?(number/path/refnum=w2510) -> (NaN/Path/Refnum?=w2509:bool)
              n1168 = case shown="False" w2509 {
                tunnel: w2517 -> [w2528 _]
                tunnel: w2516 -> [w2527 w2529]
                tunnel: w2510 -> [w2526 _]
                tunnel: [w2525 w2529] -> w2511
                tunnel: w2508 -> [w2524 _]
                tunnel: w2507 -> [w2523 _]
                frame False {
                  w2519 = "\t"
                  n1169 = call "Number_2_string.vi"("number"=w2524) -> ("String"=w2522:string)  [unwired: 1 in]
                  n1170 = call "Number_2_string.vi"("number"=w2523) -> ("String"=w2521:string)  [unwired: 1 in]
                  n1171 = call "Number_2_string.vi"("precision"=w2528, "number"=w2526) -> ("String"=w2520:string)
                  n1172 = Concatenate Strings(w2527, w2522, w2519, w2521, w2519, w2520, "\r\n") -> (w2525:string)
                }
                frame True {
                }
              }
            }
          }
          frame #4 {
            w2546 = TRUE  # append to file? (new file:F)
            n1173 = global read "Results_plotter_Global.vi" "Surface Integral"() -> (w2545:dbl)
            n1174 = global read "Results_plotter_Global.vi" "Surface Area"() -> (w2544:dbl)
            n1175 = Initialize Array("", 10 ("Dimension Size")) -> (w2555:string[])
            n1176 = Divide(x=w2545, y=w2544) -> (x/y=w2543:dbl)
            n1177 = call "Asterisk_header.vi"("Channel names"=w2555) -> ("Header string"=w2533:string)
            n1178 = call "Value_to_string.vi"("Value"=w2545, "Label for value"="Surface Integral") -> ("Output string"=w2540:string)  [unwired: 1 in]
            n1179 = call "Value_to_string.vi"("Value"=w2544, "Label for value"="Surface Area") -> ("Output string"=w2541:string)  [unwired: 1 in]
            n1180 = call "Value_to_string.vi"("Value"=w2543, "Label for value"="Surface Average") -> ("Output string"=w2539:string)  [unwired: 1 in]
            n1181 = Concatenate Strings(w2541, w2540, w2539) -> (w2536:string)
            n1182 = call "Ch_names_to_rows.vi"("Channel Names"=w2531) -> ("3 Row names"=w2530:string[][])
            n1183 = local read "Output Filename"() -> (w2547:path)
            n1184 = Build Array (concatenate)(w2530, w2550) -> (w2548:string[][])
            n1185 = Array To Spreadsheet String(array=w2548, 3:"%s" ("format string")) -> (spreadsheet string=w2535:string)  [unwired: 1 out]
            n1186 = Format Into String(format string="\n%s\n\n%s\n%s\n\n\nInterpolated Surface of %s\n%s\n%s\n%s\n\n\n%s", w2533, w2532, w2533, w2534, w2533, w2535, w2533, w2536) -> (resulting string=w2538:string)  [unwired: 2 in, 1 out]
            n1187 = call "Write_Characters_To_File.vi"("file path (dialog if empty)"=w2547, "character string"=w2538, "append to file? (new file:F)"=w2546) -> ()  [unwired: 2 in, 4 out]
          }
          frame #5 {
            n1188 = local write "Save Surface Fit"(FALSE ("Save Plot data")) -> ()
          }
        }
      }
      frame "Save Data in Rows" {
        w2572 = TRUE  # Show panel ?
        n1189 = local read "Output Filename"() -> (w2569:path)
        n1190 = local write "Save Data in Rows"(FALSE ("Save All data")) -> ()
        n1191 = call "Output_file_Panel.vi"("Show panel ?"=w2572, "Channel Names"=w2567, "Header"="Header", "Output filename"=w2569) -> ("Save Full Res Data?"=w2564:bool, "Desired Columns"=w2573:i32[], "Header Out"=w2571:string, "Output filename Out"=w2575:path, "Channels to Tabulate in header Out"=w2561:i32[], "Save Plotted rows only?"=w2562:bool, "Summarise mode"=w2570:T9, "Grouping info"=w2563:T15[])
        "Plotted rows only?" <- w2562
        n1192 = case shown="False" w2564 {
          tunnel: w2575 -> [w2591 w2593]
          tunnel: w2573 -> [w2590 _]
          tunnel: w2571 -> [w2589 _]
          tunnel: w2562 -> [w2588 _]
          tunnel: w2570 -> [w2587 _]
          tunnel: w2568 -> [w2586 _]
          tunnel: w2567 -> [w2585 _]
          tunnel: [w2584 w2593] -> w2566
          tunnel: ["Create Selectors" "Is Filename Empty?"] -> w2565
          tunnel: w2563 -> [w2580 _]
          tunnel: w2561 -> [w2579 _]
          frame False {
            w2582 = FALSE  # Simple Save?
            n1193 = local read "Template"() -> (w2583:path)
            n1194 = call "Write_output_file.vi"("Output filename"=w2591, "Header"=w2589, "Template Filename"=w2583, "Channel Names"=w2585, "Data"=w2586, "Desired Columns"=w2590, "Simple Save?"=w2582, "Save Plotted rows only?"=w2588, "Summarise mode"=w2587, "Grouping info"=w2580, "Channels to Tabulate in header"=w2579) -> ("Output filename Out"=w2584:path)  [unwired: 1 in, 3 out]
          }
          frame True {
            "Mode" <- Plotter_Mode."Save file" ("Mode")
          }
        }
        n1195 = local write "Output Filename"(w2566) -> ()
      }
      frame "Is Filename Empty?" {
        # "This Express VI is the reason we can't strip object code from ResultsFilePlotter; may be able to convert to standard VI"
        n1196 = call "File Dialog"("start path"="Full_Res_Results_Folder", "prompt"="Please select a new or existing folder to save the results files in") -> ("selected path"=w2597:path, "cancelled"=w2595:bool)  [unwired: 5 in, 7 out]
        n1197 = local write "Full_Res_Results_Folder"(w2597) -> ()
        n1198 = case shown="False" w2595 {
          tunnel: ["Full Res file manipulator" ("f") "Create Selectors" ("t")] -> w2599
          frame False {
          }
          frame True {
          }
        }
      }
      frame "Check for overwrite or append" {
        n1199 = local read "Output Filename"() -> (w2613:path)
        n1200 = Format Into String(format string="Do you want to append to the result file\n\"%s\"" ("message"), w2613) -> (resulting string=w2608:string)  [unwired: 2 in, 1 out]
        n1201 = call <vilib>:"Three Button Dialog.vi"("Window Title (\"\")"="Output File Dialog" ("Window Title (\"\")"), "Right Button Text (\"Cancel\")"="Cancel" ("Button 3 Name"), "Center Button Text (\"No\")"="Overwrite" ("F button name (\"Cancel\")"), "Left Button Text (\"Yes\")"="Append" ("T button name (\"OK\")"), "message"=w2608) -> ("Which Button?"=w2607:T11)  [unwired: 6 out]
        n1202 = case shown="\"Center Button\"" w2607 {
          tunnel: w2613 -> [_ w2620 _]
          tunnel: ["Full Res file manipulator" "Full Res file manipulator" "Create Selectors" ("t")] -> w2606
          frame "Left Button" {
          }
          frame "Center Button" {
            n1203 = call "Delete_with_Check.vi"("FilePath"=w2620) -> ()  [unwired: 1 out]
          }
          frame "Right Button", Default {
          }
        }
      }
      frame "Create Plot summary" {
        w2635 = TRUE  # Summarise All
        n1204 = global read "Results_plotter_Global.vi" "Plot Index values"() -> (w2638:dbl[][])
        n1205 = local read "Intensity Plot?"() -> (w2634:bool)
        n1206 = global read "Results_plotter_Global.vi" "Row Reference"() -> (w2630:i32[][])
        n1207 = Index Array(array=w2630, index (col)=0 ("disabled index (col)")) -> (element=w2629:i32[])  [unwired: 1 in]
        n1208 = Index Array(array=w2638, index (row)=2) -> (element=w2640:dbl[])  [unwired: 1 in]
        n1209 = Select(t="Save Intensity plot as jpg", s=w2634, f="Create summary per series") -> (s? t:f=w2625:string)
        n1210 = To Long Integer(number=w2640) -> (32bit integer=w2637:i32[])
        n1211 = for {
          tunnel: w2645 -> [w2658]
          tunnel: [w2657] -> w2636 mode=indexing
          tunnel: w2637 -> [w2655] mode=indexing
          tunnel: w2629 -> [w2656]
          shift-right: [w2652] -> w2627
          shift-left: i32[] [] -> [w2653]
          n1212 = Index Array(array=w2656, index=w2655) -> (element=w2651:i32)
          n1213 = Search 1D Array(1D array=w2653, element=w2651) -> (index of element=w2654:i32)  [unwired: 1 out]
          n1214 = Index Array(array=w2658, index (row)=w2655) -> (element=w2657:string[])  [unwired: 1 in]
          n1215 = case shown="0, Default" w2654 {
            tunnel: w2651 -> [_ w2662]
            tunnel: w2653 -> [w2659 w2661]
            tunnel: [w2659 w2660] -> w2652
            frame 0, Default {
            }
            frame -1 {
              n1216 = Build Array (concatenate)(w2661, w2662) -> (w2660:i32[])
            }
          }
        }
        n1217 = local read "Result files to read"() -> (w2626:path[])
        n1218 = for {
          tunnel: w2627 -> [w2650] mode=indexing
          tunnel: w2626 -> [w2649]
          tunnel: [w2646] -> w2624 mode=indexing
          n1219 = Index Array(array=w2649, index=w2650) -> (element=w2648:path)
          n1220 = Strip Path(path=w2648) -> (name=w2647:string)  [unwired: 1 out]
          n1221 = call "Add_filename_suffix.vi"("Filename"=w2647) -> ("Base name"=w2646:string)  [unwired: 1 in, 3 out]
        }
        n1222 = call "Value_Occurence_Analysis.vi"("String Array"=w2624) -> ("Output String"=w2623:string)  [unwired: 3 in, 2 out]
        n1223 = global write "Results_plotter_Global.vi" "Current Data Filenames"(w2623) -> ()
        n1224 = call "Summarise.vi"("Channel Names"=w2641, "Data"=w2636, "Summarise All"=w2635) -> ("Summary"=w2643:string[][])  [unwired: 2 in]
        n1225 = global write "Results_plotter_Global.vi" "Plot Summary"(w2643) -> ()
      }
      frame "Create summary per series" {
        n1226 = global read "Results_plotter_Global.vi" "Plot Summary"() -> (w2664:string[][])
        n1227 = local read "Plotted Series"() -> (w2666:bool[][])
        n1228 = for {
          tunnel: w2666 -> [w2683] mode=indexing
          tunnel: i32[] [] -> [w2682]
          tunnel: w2671 -> [w2680]
          tunnel: w2668 -> [w2678]
          shift-right: [w2672] -> w2663
          shift-left: w2664 -> [w2674]
          w2677 = TRUE  # Summarise All
          n1229 = for {
            shift-right: [w2691] -> w2681
            shift-left: w2682 -> [w2692]
            tunnel: w2683 -> [w2690] mode=indexing
            i -> [w2693]
            n1230 = case shown="True" w2690 {
              tunnel: w2693 -> [_ w2697]
              tunnel: w2692 -> [w2694 w2696]
              tunnel: [w2694 w2695] -> w2691
              frame False {
              }
              frame True {
                n1231 = Build Array (concatenate)(w2696, w2697) -> (w2695:i32[])
              }
            }
          }
          n1232 = for {
            tunnel: w2681 -> [w2689] mode=indexing
            tunnel: w2680 -> [w2688]
            tunnel: [w2687] -> w2679 mode=indexing
            n1233 = Index Array(array=w2688, index (row)=w2689) -> (element=w2687:string[])  [unwired: 1 in]
          }
          n1234 = call "Summarise.vi"("Channel Names"=w2678, "Data"=w2679, "Summarise All"=w2677) -> ("Summary"=w2675:string[][])  [unwired: 2 in]
          n1235 = Index Array(array=w2675, index (col)=2 ("disabled index (col)")) -> (element=w2673:string[])  [unwired: 1 in]
          n1236 = for {
            tunnel: w2674 -> [w2686] mode=indexing
            tunnel: w2673 -> [w2685] mode=indexing
            tunnel: [w2684] -> w2672 mode=indexing
            n1237 = Build Array (concatenate)(w2686, w2685) -> (w2684:string[])
          }
        }
        n1238 = global write "Results_plotter_Global.vi" "Plot Summary"(w2663) -> ()
      }
      frame "Save Intensity plot as jpg" {
        n1239 = local read "Job Directory"() -> (w2704:path)
        n1240 = global read "Constants_global.vi" "EnFlo SW Folder"() -> (w2706:path)
        n1241 = Build Path(base path=w2706, name or relative path=path "Anemometry/Anemometry Sub Vis/Data_plotting_vis/Intensity Plot Vis") -> (appended path=w2700:path)
        n1242 = call "Remote_call_prep.vi"("Vi Name in"="Create picture Vi Name", "Job Directory In"=w2704, "VI Directory"=w2700) -> ("Vi Name out"=w2702:string, "Job Directory out"=w2699:path, "cancelled"=w2698:bool)
        n1243 = local write "Create picture Vi Name"(w2702) -> ()
        n1244 = local write "Job Directory"(w2699) -> ()
        n1245 = Build Path(base path=w2700, name or relative path=w2702) -> (appended path=w2701:path)
        n1246 = case shown="False" w2698 {
          tunnel: w2701 -> [w2715 _]
          tunnel: w2699 -> [w2714 _]
          frame False {
            n1247 = Open VI Reference(type specifier VI Refnum (for type only)="type specifier VI Refnum (for type only)", vi path=w2715) -> (vi reference=w2720:refnum<vi>, error out=w2719:errorcluster)  [unwired: 2 in, 2 out]
            n1248 = property class="VI Interface Type 1"(reference=w2720, error in=w2719, "Front Panel Window:Open"=TRUE) -> (reference out=w2716:refnum<vi>, error out=w2717:errorcluster)
            n1249 = local read "Intensity Graph"() -> (w2723:dbl[][])
            n1250 = local read "No of Contours"() -> (w2713:i32)
            n1251 = call-by-ref "?"(reference=w2716, error in=w2717, "No of Contours"=w2713, "Job Directory"=w2714, "Intensity Graph"=w2723) -> (reference out=w2722:refnum<vi>, error out=w2721:errorcluster)  [unwired: 3 in]
            n1252 = Close Reference(reference=w2722, error in (no error)=w2721) -> ()  [unwired: 1 out]
          }
          frame True {
          }
        }
        n1253 = local write "Save Plot as jpg"(FALSE ("Save All data")) -> ()
      }
      frame "Run Calculation Routine" {
        n1254 = stacked-sequence {
          seq-local: [w2732 _ _] -> [_ w2742 _]
          seq-local: [w2731 _ _] -> [_ w2743 _]
          tunnel: [_ w2741 _] -> w2726
          tunnel: w2725 -> [_ _ _]
          frame #0 {
            n1255 = global read "Constants_global.vi" "EnFlo SW Folder"() -> (w2738:path)
            n1256 = local read "Job Directory"() -> (w2734:path)
            n1257 = Build Path(base path=w2738, name or relative path=path "Anemometry/Anemometry Sub Vis/Data_plotting_vis/Calculation Vis") -> (appended path=w2735:path)
            n1258 = call "Remote_call_prep.vi"("Vi Name in"="...using routine", "Job Directory In"=w2734, "VI Directory"=w2735) -> ("Vi Name out"=w2736:string, "Job Directory out"=w2733:path, "cancelled"=w2732:bool)
            n1259 = local write "Job Directory"(w2733) -> ()
            n1260 = local write "...using routine"(w2736) -> ()
            n1261 = Build Path(base path=w2735, name or relative path=w2736) -> (appended path=w2731:path)
          }
          frame #1 {
            n1262 = case shown="False" w2742 {
              tunnel: w2743 -> [w2751 _]
              tunnel: [w2747 w2764] -> w2741
              tunnel: "What to do next?" -> [w2746 w2764]
              frame False {
                n1263 = Open VI Reference(type specifier VI Refnum (for type only)="VI Refnum Calculation", vi path=w2751) -> (vi reference=w2757:refnum<vi>, error out=w2756:errorcluster)  [unwired: 1 in, 3 out]
                n1264 = property class="VI Interface Type 0"(reference=w2757, error in=w2756, "Front Panel Window:Open"=TRUE) -> (reference out=w2753:refnum<vi>, error out=w2754:errorcluster)
                n1265 = call-by-ref "?"(reference=w2753, error in=w2754) -> (reference out=w2759:refnum<vi>, error out=w2758:errorcluster, "New Values In"=w2744:string[][], "New Chs In"=w2752:string[])  [unwired: 2 in]
                n1266 = for {
                  tunnel: w2752 -> [w2762] mode=indexing
                  tunnel: [w2761] -> w2745 mode=indexing
                  n1267 = call "Check_Ch_Name_colons.vi"("No of Colons"=2, "Ch Name in"=w2762) -> ("Ch Name out"=w2761:string)
                }
                n1268 = Empty String/Path?(string/path=w2745) -> (empty?=w2749:bool[])
                n1269 = Or Array Elements(Boolean array=w2749) -> (logical OR=w2748:bool)
                n1270 = Close Reference(reference=w2759, error in (no error)=w2758) -> ()  [unwired: 1 out]
                n1271 = Select(t=w2746, s=w2748, f="Input calculated values") -> (s? t:f=w2747:string)
                n1272 = global write "Results_plotter_Global.vi" "New Values In"(w2744) -> ()
                n1273 = global write "Results_plotter_Global.vi" "New Chs In"(w2745) -> ()
              }
              frame True {
              }
            }
          }
          frame #2 {
            w2767 = FALSE ("Raw DF in Orig Pos?")
            n1274 = local write "Edit Raw Data Header Info"(w2767) -> ()
            n1275 = local write "Calculate new metadata"(FALSE ("Save All data")) -> ()
            n1276 = local write "Plotted rows only?"(TRUE ("Plotted rows only?")) -> ()
            n1277 = local write "Raw DF in Orig Pos?"(w2767) -> ()
            n1278 = local write "Edit Raw DF?"(w2767) -> ()
            n1279 = local write "Mode"(Plotter_Mode."Edit values per row" ("Mode")) -> ()
          }
        }
      }
      frame "Input calculated values" {
        n1280 = local read "Result files to read"() -> (w2773:path[])
        n1281 = local read "Raw DF in Orig Pos?"() -> (w2770:bool)
        n1282 = stacked-sequence {
          seq-local: [w2777 _ _ _] -> [_ w2790 w2802 _]
          seq-local: [_ w2787 _ _] -> [_ _ w2803 _]
          tunnel: [_ _ _ w2855] -> w2775
          tunnel: w2773 -> [_ _ w2804 _]
          tunnel: w2772 -> [_ _ w2801 _]
          tunnel: w2771 -> [_ _ w2800 _]
          tunnel: w2770 -> [_ _ w2799 _]
          tunnel: w2769 -> [_ _ _ w2852]
          frame #0 {
            n1283 = global read "Results_plotter_Global.vi" "Plot Index values"() -> (w2780:dbl[][])
            n1284 = global read "Results_plotter_Global.vi" "Row Reference"() -> (w2781:i32[][])
            n1285 = Index Array(array=w2780, index (row)=2) -> (element=w2778:dbl[])  [unwired: 1 in]
            n1286 = for {
              tunnel: w2781 -> [w2785]
              tunnel: w2778 -> [w2784] mode=indexing
              tunnel: [w2783] -> w2777 mode=indexing
              n1287 = Index Array(array=w2785, index (row)=w2784) -> (element=w2783:i32[])  [unwired: 1 in]
            }
            n1288 = local write "Delete Plotted data from file"(FALSE ("Save All data")) -> ()
          }
          frame #1 {
            n1289 = Index Array(array=w2790, index (col)=0 ("disabled index (col)")) -> (element=w2786:i32[])  [unwired: 1 in]
            n1290 = for {
              shift-right: [w2792] -> w2787
              shift-left: i32[] [] -> [w2793]
              tunnel: w2786 -> [w2791] mode=indexing
              n1291 = Search 1D Array(1D array=w2793, element=w2791) -> (index of element=w2794:i32)  [unwired: 1 out]
              n1292 = case shown="-1" w2794 {
                tunnel: w2793 -> [w2795 w2798]
                tunnel: [w2795 w2797] -> w2792
                tunnel: w2791 -> [_ w2796]
                frame 0, Default {
                }
                frame -1 {
                  n1293 = Build Array (concatenate)(w2798, w2796) -> (w2797:i32[])
                }
              }
            }
          }
          frame #2 {
            n1294 = for {
              tunnel: w2804 -> [w2811]
              tunnel: w2803 -> [w2808] mode=indexing
              tunnel: w2802 -> [w2809]
              tunnel: w2801 -> [w2807]
              tunnel: w2800 -> [w2806]
              tunnel: w2799 -> [w2805]
              # "New Values"
              # "Row in file"
              n1295 = Index Array(array=w2811, index=w2808) -> (element=w2810:path)
              n1296 = stacked-sequence {
                seq-local: [w2816 _] -> [_ w2850]
                seq-local: [w2814 _] -> [_ w2845]
                tunnel: w2810 -> [_ w2851]
                tunnel: w2809 -> [w2818 _]
                tunnel: w2808 -> [w2817 _]
                tunnel: w2807 -> [_ _]
                tunnel: w2806 -> [_ _]
                tunnel: w2805 -> [_ w2849]
                frame #0 {
                  n1297 = global read "Results_plotter_Global.vi" "New Values In"() -> (w2812:string[][])
                  n1298 = for {
                    tunnel: w2817 -> [w2829]
                    tunnel: w2818 -> [w2825] mode=indexing
                    shift-right: [w2823] -> w2816
                    shift-left: i32[] [] -> [w2824]
                    shift-right: [w2822] -> w2814
                    shift-left: string[][] [] -> [w2821]
                    tunnel: w2812 -> [w2820]
                    i -> [w2819]
                    n1299 = Index Array(array=w2825, index=0) -> (element=w2827:i32)
                    n1300 = Equal?(x=w2827, y=w2829) -> (x = y?=w2826:bool)
                    n1301 = case shown="False" w2826 {
                      tunnel: w2825 -> [_ w2835]
                      tunnel: w2824 -> [w2831 w2840]
                      tunnel: [w2831 w2838] -> w2823
                      tunnel: w2821 -> [w2830 w2836]
                      tunnel: [w2830 w2837] -> w2822
                      tunnel: w2820 -> [_ w2833]
                      tunnel: w2819 -> [_ w2832]
                      frame False {
                      }
                      frame True {
                        n1302 = Index Array(array=w2833, index (row)=w2832) -> (element=w2834:string[])  [unwired: 1 in]
                        n1303 = Index Array(array=w2835, index=1) -> (element=w2839:i32)
                        n1304 = Build Array (concatenate)(w2840, w2839) -> (w2838:i32[])
                        n1305 = Build Array (concatenate)(w2836, w2834) -> (w2837:string[][])
                      }
                    }
                  }
                }
                frame #1 {
                  w2844 = FALSE  # Edit all Rows?
                  w2846 = FALSE  # Edit Raw DF?
                  w2847 = FALSE  # Edit Raw Data Header Info
                  w2848 = FALSE  # Value  Constant?
                  n1306 = global read "Results_plotter_Global.vi" "New Chs In"() -> (w2842:string[])
                  n1307 = local read "Job Directory"() -> (w2843:path)
                  n1308 = call "Add_Update_Values.vi"("Filename"=w2851, "Value  Constant?"=w2848, "Edit Raw data files?"=w2846, "New Chs In"=w2842, "Edit Raw Data Header Info"=w2847, "New Values In"=w2845, "Selected Rows"=w2850, "Edit all Rows?"=w2844, "Raw DF in Orig Pos?"=w2849, "Job Directory"=w2843) -> ()  [unwired: 1 in, 5 out]
                }
              }
            }
          }
          frame #3 {
            n1309 = local read "nRows"() -> (w2854:i32)
            n1310 = Less?(x=w2854, y=w2852) -> (x < y?=w2853:bool)
            n1311 = Current VI's Path() -> (path=w2856:path)
            n1312 = case shown="True" w2853 {
              tunnel: ["Create Selectors" "Initialise" ("t")] -> w2855
              frame False {
              }
              frame True {
              }
            }
            n1313 = call "Bring_to_front.vi"("path"=w2856) -> ()
          }
        }
      }
      frame "Save XY plot as jpg" {
        n1314 = local read "Create picture Vi Name"() -> (w2863:string)
        n1315 = local read "Job Directory"() -> (w2866:path)
        n1316 = global read "Constants_global.vi" "EnFlo SW Folder"() -> (w2868:path)
        n1317 = Build Path(base path=w2868, name or relative path=path "Anemometry/Anemometry Sub Vis/Data_plotting_vis/XY Plot Vis") -> (appended path=w2864:path)
        n1318 = call "Remote_call_prep.vi"("Vi Name in"=w2863, "Job Directory In"=w2866, "VI Directory"=w2864) -> ("Vi Name out"=w2865:string, "Job Directory out"=w2861:path, "cancelled"=w2860:bool)
        n1319 = local write "Create picture Vi Name"(w2865) -> ()
        n1320 = local write "Job Directory"(w2861) -> ()
        n1321 = Build Path(base path=w2864, name or relative path=w2865) -> (appended path=w2862:path)
        n1322 = case shown="False" w2860 {
          tunnel: [w2881 FALSE ("Saved Automatically?")] -> w2871
          tunnel: [w2880 path "" ("Plot data file")] -> w2870
          tunnel: [w2879 "" ("Tex Info String")] -> w2869
          tunnel: w2862 -> [w2878 _]
          tunnel: w2861 -> [w2877 _]
          frame False {
            n1323 = Open VI Reference(type specifier VI Refnum (for type only)="type specifier VI Refnum (for type only) 2", vi path=w2878) -> (vi reference=w2888:refnum<vi>, error out=w2887:errorcluster)  [unwired: 1 in, 3 out]
            n1324 = property class="VI Interface Type 2"(reference=w2888, error in=w2887, "Front Panel Window:Open"=TRUE) -> (reference out=w2884:refnum<vi>, error out=w2885:errorcluster)
            n1325 = global read "Results_plotter_Global.vi" "XY Graph Cluster"() -> (w2882:cluster{dbl[], dbl[]}[])
            n1326 = call-by-ref "?"(reference=w2884, error in=w2885, "Plot Array"=w2882, "Template"=w2877) -> (reference out=w2890:refnum<vi>, error out=w2889:errorcluster, "Saved Automatically?"=w2881:bool, "Tex Info String"=w2879:string, "Plot data file"=w2880:path)
            n1327 = Close Reference(reference=w2890, error in (no error)=w2889) -> ()  [unwired: 1 out]
          }
          frame True {
          }
        }
        n1328 = local write "Save Plot as jpg"(FALSE ("Save All data")) -> ()
        n1329 = case shown="True" w2871 {
          tunnel: w2870 -> [_ w2902]
          tunnel: [w2894 "Save Plot Data"] -> w2859
          tunnel: w2869 -> [_ w2900]
          frame False {
            n1330 = global read "Results_plotter_Global.vi" "New Chs In"() -> (w2899:string[])
            n1331 = Array Size(array=w2899) -> (size(s)=w2898:i32)
            n1332 = Greater Than 0?(x=w2898) -> (x > 0?=w2897:bool)
            n1333 = Select(t="Input calculated values", s=w2897, f="Create Selectors") -> (s? t:f=w2894:string)
          }
          frame True {
            n1334 = local write "Output Filename"(w2902) -> ()
            n1335 = local write "Header"(w2900) -> ()
          }
        }
      }
      frame "Full Res file manipulator" {
        n1336 = local read "Result files to read"() -> (w2912:path[])
        n1337 = local read "Output Filename"() -> (w2910:path)
        n1338 = local read "Mode"() -> (w2911:T4)
        n1339 = local read "Raw DF in Orig Pos?"() -> (w2907:bool)
        n1340 = global read "Results_plotter_Global.vi" "New Values In"() -> (w2904:string[][])
        n1341 = local read "Plotted rows only?"() -> (w2903:bool)
        n1342 = global read "Results_plotter_Global.vi" "New Chs In"() -> (w2905:string[])
        n1343 = stacked-sequence {
          seq-local: [w2917 _ _ _ _] -> [_ w2945 w2998 _ _]
          seq-local: [_ w2944 _ _ _] -> [_ _ w2981 _ _]
          seq-local: [_ w2940 _ _ _] -> [_ _ w2990 _ _]
          seq-local: [_ _ w2988 _ _] -> [_ _ _ w3242 _]
          seq-local: [_ _ w2987 _ _] -> [_ _ _ w3241 _]
          seq-local: [_ _ w2982 _ _] -> [_ _ _ w3238 _]
          tunnel: [_ _ _ w3245 _] -> w2914
          tunnel: w2912 -> [_ _ w2999 _ _]
          tunnel: w2911 -> [_ w2942 w2997 w3243 _]
          tunnel: w2910 -> [_ _ w2996 _ _]
          tunnel: w2903 -> [w2916 _ w2995 _ _]
          tunnel: w2905 -> [_ _ w2994 _ _]
          tunnel: w2909 -> [_ _ w2993 w3239 _]
          tunnel: w2908 -> [_ _ w2992 w3240 _]
          tunnel: w2907 -> [_ _ w2991 _ _]
          tunnel: w2906 -> [_ _ _ w3244 _]
          tunnel: w2904 -> [_ _ w2984 _ _]
          frame #0 {
            n1344 = global read "Results_plotter_Global.vi" "Row Reference"() -> (w2918:i32[][])
            n1345 = case shown="True" w2916 {
              tunnel: w2918 -> [w2920 w2921]
              tunnel: [w2920 w2922] -> w2917
              frame False {
              }
              frame True {
                n1346 = local read "Plotted Series"() -> (w2924:bool[][])
                n1347 = for {
                  tunnel: w2924 -> [w2931]
                  shift-right: [w2925] -> w2922
                  shift-left: i32[][] [] -> [w2927]
                  tunnel: w2921 -> [w2926] mode=indexing
                  i -> [w2930]
                  n1348 = Index Array(array=w2931, index (col)=w2930) -> (element=w2929:bool[])  [unwired: 1 in]
                  n1349 = Or Array Elements(Boolean array=w2929) -> (logical OR=w2928:bool)
                  n1350 = case shown="True" w2928 {
                    tunnel: w2927 -> [w2932 w2935]
                    tunnel: w2926 -> [_ w2934]
                    tunnel: [w2932 w2933] -> w2925
                    frame False {
                    }
                    frame True {
                      n1351 = Build Array (concatenate)(w2935, w2934) -> (w2933:i32[][])
                    }
                  }
                }
              }
            }
            n1352 = local write "Delete Plotted data from file"(FALSE ("Save All data")) -> ()
          }
          frame #1 {
            n1353 = local read "Job Directory"() -> (w2941:path)
            n1354 = case shown="\"Edit Raw Data file header\"" w2942 {
              tunnel: [FALSE FALSE FALSE w2962 w2965 w2968 w2971 w2974] -> w2943
              tunnel: [w2954 w2956 w2958 w2960 w2963 w2966 w2969 w2972] -> w2940
              tunnel: w2941 -> [w2954 w2956 w2958 w2961 w2964 w2967 w2970 w2973]
              tunnel: [w2954 w2956 w2958 w2960 w2963 w2966 w2969 w2972] -> w2939
              frame "Post Process Plotted Rows" {
              }
              frame "Save file" {
              }
              frame "Plot EnFlo Tunnel Display" {
              }
              frame "Delete unwanted rows" {
                n1355 = call "Remote_call_prep.vi"("Job Directory In"=w2961) -> ("Job Directory out"=w2960:path)  [unwired: 2 in, 2 out]
                n1356 = local write "Job Directory"(w2960) -> ()
                n1357 = Not Equal?(x=w2961, y=w2960) -> (x != y?=w2962:bool)
              }
              frame "Add Inlet Temperature Offset" {
                n1358 = call "Remote_call_prep.vi"("Job Directory In"=w2964) -> ("Job Directory out"=w2963:path)  [unwired: 2 in, 2 out]
                n1359 = local write "Job Directory"(w2963) -> ()
                n1360 = Not Equal?(x=w2964, y=w2963) -> (x != y?=w2965:bool)
              }
              frame "Edit Values with constants" {
                n1361 = call "Remote_call_prep.vi"("Job Directory In"=w2967) -> ("Job Directory out"=w2966:path)  [unwired: 2 in, 2 out]
                n1362 = local write "Job Directory"(w2966) -> ()
                n1363 = Not Equal?(x=w2967, y=w2966) -> (x != y?=w2968:bool)
              }
              frame "Edit values per row" {
                n1364 = call "Remote_call_prep.vi"("Job Directory In"=w2970) -> ("Job Directory out"=w2969:path)  [unwired: 2 in, 2 out]
                n1365 = local write "Job Directory"(w2969) -> ()
                n1366 = Not Equal?(x=w2970, y=w2969) -> (x != y?=w2971:bool)
              }
              frame "Edit Raw Data file header" {
                n1367 = call "Remote_call_prep.vi"("Job Directory In"=w2973) -> ("Job Directory out"=w2972:path)  [unwired: 2 in, 2 out]
                n1368 = local write "Job Directory"(w2972) -> ()
                n1369 = Not Equal?(x=w2973, y=w2972) -> (x != y?=w2974:bool)
              }
            }
            n1370 = Index Array(array=w2945, index (col)=0 ("disabled index (col)")) -> (element=w2937:i32[])  [unwired: 1 in]
            n1371 = for {
              shift-right: [w2947] -> w2944
              shift-left: i32[] [] -> [w2948]
              tunnel: w2937 -> [w2946] mode=indexing
              n1372 = Search 1D Array(1D array=w2948, element=w2946) -> (index of element=w2949:i32)  [unwired: 1 out]
              n1373 = case shown="-1" w2949 {
                tunnel: w2948 -> [w2950 w2953]
                tunnel: [w2950 w2952] -> w2947
                tunnel: w2946 -> [_ w2951]
                frame 0, Default {
                }
                frame -1 {
                  n1374 = Build Array (concatenate)(w2953, w2951) -> (w2952:i32[])
                }
              }
            }
            n1375 = case shown="True" w2943 {
              tunnel: w2939 -> [_ w2976]
              frame False {
              }
              frame True {
                n1376 = local read "Template"() -> (w2975:path)
                n1377 = Path To String(path=w2976) -> (string=w2979:string)
                n1378 = call "Read_Write_Template.vi"("Template File"=w2975, "Mode"=Global_mode."Write Global to File", "Single Value In"=w2979, "Data type"="Log Folder Name" ("Variable name")) -> ()  [unwired: 4 in, 8 out]
              }
            }
          }
          frame #2 {
            w2986 = path[] []
            n1379 = Array Size(array=w2981) -> (size(s)=w2980:i32)
            n1380 = local read "Full_Res_Results_Folder"() -> (w2985:path)
            n1381 = for {
              tunnel: w2999 -> [w3023]
              tunnel: w2981 -> [w3020] mode=indexing
              tunnel: w2998 -> [w3021]
              tunnel: w2997 -> [w3019]
              tunnel: w2996 -> [w3018]
              tunnel: w2995 -> [w3017]
              tunnel: w2994 -> [w3016]
              tunnel: w2993 -> [w3015]
              tunnel: w2992 -> [w3014]
              tunnel: w2991 -> [w3013]
              tunnel: w2990 -> [w3012]
              shift-right: [w3011] -> _
              shift-left: FALSE -> [w3010]
              shift-right: [w3008] -> w2988
              shift-left: w2986 -> [w3009]
              shift-right: [w3006] -> w2987
              shift-left: w2986 -> [w3007]
              tunnel: w2985 -> [w3005]
              tunnel: w2984 -> [w3004]
              shift-right: [w3002] -> w2982
              shift-left: i32[] [] -> [w3003]
              tunnel: w2980 -> [w3000]
              i -> [w3001]
              # "Row No in file"
              # "Row No in plotter"
              n1382 = Index Array(array=w3023, index=w3020) -> (element=w3022:path)
              n1383 = stacked-sequence {
                seq-local: [w3028 _ _ _] -> [_ w3064 w3120 _]
                seq-local: [_ w3062 _ _] -> [_ _ w3119 _]
                seq-local: [w3024 _ _ _] -> [_ _ w3112 w3236]
                tunnel: w3022 -> [_ w3063 w3121 _]
                tunnel: w3021 -> [w3038 _ _ _]
                tunnel: w3020 -> [w3031 _ _ _]
                tunnel: w3019 -> [_ w3061 w3118 _]
                tunnel: w3018 -> [_ _ w3117 _]
                tunnel: w3017 -> [_ _ w3116 _]
                tunnel: w3016 -> [_ _ w3115 _]
                tunnel: w3015 -> [_ _ w3114 _]
                tunnel: w3014 -> [_ _ w3113 _]
                tunnel: w3013 -> [_ _ w3111 _]
                tunnel: w3012 -> [_ _ w3110 _]
                tunnel: [_ w3060 _ _] -> w3011
                tunnel: w3010 -> [_ w3059 _ _]
                tunnel: w3009 -> [_ _ w3109 _]
                tunnel: [_ _ w3108 _] -> w3008
                tunnel: w3007 -> [_ _ w3107 _]
                tunnel: [_ _ w3106 _] -> w3006
                tunnel: w3005 -> [_ _ w3105 _]
                tunnel: w3004 -> [_ _ w3104 _]
                tunnel: w3003 -> [_ _ _ w3237]
                tunnel: [_ _ _ w3235] -> w3002
                tunnel: w3001 -> [_ _ w3103 _]
                tunnel: w3000 -> [_ _ w3102 _]
                frame #0 {
                  w3037 = i32[] []
                  # "10/30/13\n#optimation"
                  n1384 = global read "Results_plotter_Global.vi" "Row Reference"() -> (w3036:i32[][])
                  n1385 = local read "Cursor index"() -> (w3035:i32)
                  n1386 = for {
                    tunnel: w3031 -> [w3047]
                    tunnel: w3038 -> [w3043] mode=indexing
                    shift-right: [w3041] -> w3029
                    shift-left: w3037 -> [w3042]
                    shift-right: [w3040] -> w3025
                    shift-left: w3037 -> [w3039]
                    n1387 = Index Array(array=w3043, index=0) -> (element=w3045:i32)
                    n1388 = Equal?(x=w3045, y=w3047) -> (x = y?=w3044:bool)
                    n1389 = case shown="True" w3044 {
                      tunnel: w3043 -> [_ w3051]
                      tunnel: w3042 -> [w3049 w3057]
                      tunnel: [w3049 w3055] -> w3041
                      tunnel: w3039 -> [w3048 w3053]
                      tunnel: [w3048 w3054] -> w3040
                      frame False {
                      }
                      frame True {
                        n1390 = Index Array(array=w3051, index=2) -> (element=w3050:i32)
                        n1391 = Build Array (concatenate)(w3053, w3050) -> (w3054:i32[])
                        n1392 = Index Array(array=w3051, index=1) -> (element=w3056:i32)
                        n1393 = Build Array (concatenate)(w3057, w3056) -> (w3055:i32[])
                      }
                    }
                  }
                  n1394 = Index Array(array=w3036, index (row)=w3035) -> (element=w3033:i32[])  [unwired: 1 in]
                  n1395 = local read "Selected Row?"() -> (w3026:bool)
                  n1396 = Index Array(array=w3033, index #1=0 ("index"), index #2=1 ("index")) -> (element #2=w3030:i32)  [unwired: 1 out]
                  n1397 = Build Array(w3030) -> (w3027:i32[])
                  n1398 = Select(t=w3027, s=w3026, f=w3025) -> (s? t:f=w3024:i32[])
                  n1399 = Select(t=w3027, s=w3026, f=w3029) -> (s? t:f=w3028:i32[])
                }
                frame #1 {
                  n1400 = case shown="\"Add Inlet Temperature Offset\"" w3061 {
                    tunnel: w3064 -> [_ _ _ _ _ _ _ w3085]
                    tunnel: w3063 -> [_ _ _ _ _ _ _ w3083]
                    tunnel: [TRUE ("T button?") TRUE ("T button?") TRUE ("T button?") TRUE ("T button?") TRUE ("T button?") TRUE ("T button?") TRUE ("T button?") w3082] -> w3062
                    tunnel: [w3065 w3067 w3070 w3072 w3074 w3076 w3078 w3081] -> w3060
                    tunnel: w3059 -> [w3065 w3067 w3070 w3072 w3074 w3076 w3078 w3080]
                    frame "Save file" {
                    }
                    frame "Add Inlet Temperature Offset" {
                    }
                    frame "Plot EnFlo Tunnel Display" {
                      n1401 = local read "Index when last plotted"() -> (→"Index when last displayed":i32)
                    }
                    frame "Edit values per row" {
                    }
                    frame "Edit Values with constants" {
                    }
                    frame "Edit Raw Data file header" {
                    }
                    frame "Post Process Plotted Rows" {
                    }
                    frame "Delete unwanted rows" {
                      n1402 = Array Size(array=w3085) -> (size(s)=w3084:i32)
                      n1403 = case shown="False" w3080 {
                        tunnel: w3084 -> [w3094 _]
                        tunnel: w3083 -> [w3093 _]
                        tunnel: [w3088 w3101] -> w3082
                        tunnel: [w3087 w3101] -> w3081
                        frame False {
                          n1404 = Format Into String(format string="Remove %d rows from \"%s\"", w3094, w3093) -> (resulting string=w3091:string)  [unwired: 2 in, 1 out]
                          n1405 = call <vilib>:"Three Button Dialog.vi"("Allow user to close window? (TRUE)"=TRUE, "Right Button Text (\"Cancel\")"="Yes To All Files" ("Right Button Text (\"Cancel\")"), "message"=w3091) -> ("Which Button?"=w3089:T11)  [unwired: 3 in, 5 out]
                          n1406 = case shown="\"Left Button\"" w3089 {
                            tunnel: [TRUE TRUE w3099 w3100] -> w3088
                            tunnel: [FALSE TRUE w3099 w3100] -> w3087
                            frame "Left Button" {
                            }
                            frame "Right Button" {
                            }
                            frame "Center Button" {
                              w3099 = FALSE
                            }
                            frame "Window Close" {
                              w3100 = FALSE
                            }
                          }
                        }
                        frame True {
                          w3101 = TRUE
                        }
                      }
                    }
                  }
                }
                frame #2 {
                  n1407 = case shown="True" w3119 {
                    tunnel: w3121 -> [_ w3142]
                    tunnel: w3120 -> [_ w3141]
                    tunnel: w3118 -> [_ w3140]
                    tunnel: w3117 -> [_ w3139]
                    tunnel: w3116 -> [_ w3138]
                    tunnel: w3115 -> [_ w3137]
                    tunnel: w3114 -> [_ w3136]
                    tunnel: w3113 -> [_ w3135]
                    tunnel: w3112 -> [_ w3134]
                    tunnel: w3111 -> [_ w3133]
                    tunnel: w3110 -> [_ w3132]
                    tunnel: w3109 -> [w3123 w3131]
                    tunnel: [w3123 w3130] -> w3108
                    tunnel: w3107 -> [w3122 w3129]
                    tunnel: [w3122 w3128] -> w3106
                    tunnel: w3105 -> [_ w3127]
                    tunnel: w3104 -> [_ w3126]
                    tunnel: w3103 -> [_ w3125]
                    tunnel: w3102 -> [_ w3124]
                    frame False {
                    }
                    frame True {
                      n1408 = case shown="\"Add Inlet Temperature Offset\"" w3140 {
                        tunnel: w3142 -> [w3148 w3154 w3172 w3179 w3185 w3206 w3223]
                        tunnel: w3141 -> [w3151 w3161 w3171 w3178 w3186 w3205 w3222]
                        tunnel: w3139 -> [_ _ _ _ _ _ _]
                        tunnel: w3138 -> [_ _ _ _ _ w3203 w3220]
                        tunnel: w3137 -> [_ _ _ _ _ w3201 w3218]
                        tunnel: w3136 -> [_ _ _ _ w3184 _ w3217]
                        tunnel: w3135 -> [_ _ _ _ w3187 _ w3215]
                        tunnel: w3134 -> [_ _ _ _ w3188 _ w3214]
                        tunnel: w3133 -> [_ _ _ _ _ w3200 w3212]
                        tunnel: w3132 -> [_ _ _ _ _ w3198 w3210]
                        tunnel: w3131 -> [w3150 w3158 w3170 w3181 w3190 w3196 w3208]
                        tunnel: [w3150 w3159 w3170 w3181 w3190 w3196 w3208] -> w3130
                        tunnel: w3129 -> [w3149 w3157 w3169 w3180 w3189 w3195 w3207]
                        tunnel: [w3149 w3155 w3169 w3180 w3189 w3195 w3207] -> w3128
                        tunnel: w3127 -> [w3147 _ _ _ _ _ _]
                        tunnel: w3126 -> [_ _ _ _ _ w3194 _]
                        tunnel: w3125 -> [_ _ _ w3174 _ _ _]
                        tunnel: w3124 -> [_ _ _ w3176 _ _ _]
                        frame "Save file" {
                          n1409 = Strip Path(path=w3148) -> (name=w3145:string)  [unwired: 1 out]
                          n1410 = call "Add_filename_suffix.vi"("Filename"=w3145, "Suffix to add"=".xls") -> ("Filename out"=w3143:string)  [unwired: 3 out]
                          n1411 = Build Path(base path=w3147, name or relative path=w3143) -> (appended path=w3146:path)
                          n1412 = call "Save_full_Res_rows.vi"("Selected Rows"=w3151, "Filename to write"=w3146, "Filename Orig"=w3148) -> ()  [unwired: 2 out]
                        }
                        frame "Edit Raw Data file header", Default {
                          n1413 = call "GetRawDataFilePaths.vi"("Results file or Folder"=w3154) -> ("RawDataFilePaths"=w3152:string[], "RowNumbers"=w3153:i32[])  [unwired: 9 in]
                          n1414 = for {
                            tunnel: w3152 -> [w3168]
                            tunnel: w3161 -> [w3162] mode=indexing
                            tunnel: [w3166] -> w3160 mode=indexing
                            tunnel: [w3165] -> w3156 mode=indexing
                            tunnel: w3154 -> [w3165]
                            tunnel: w3153 -> [w3164]
                            n1415 = Search 1D Array(1D array=w3164, element=w3162) -> (index of element=w3163:i32)  [unwired: 1 in]
                            n1416 = Index Array(array=w3168, index=w3163) -> (element=w3167:string)
                            n1417 = call "String_to_Pathname.vi"("Input String"=w3167) -> ("path"=w3166:path)
                          }
                          n1418 = Build Array (concatenate)(w3157, w3156) -> (w3155:path[])
                          n1419 = Build Array (concatenate)(w3158, w3160) -> (w3159:path[])
                        }
                        frame "Delete unwanted rows" {
                          n1420 = call "Delete_unwanted_rows.vi"("Selected Rows"=w3171, "Filename"=w3172) -> ()  [unwired: 1 out]
                        }
                        frame "Plot EnFlo Tunnel Display" {
                          n1421 = Decrement(x=w3176) -> (x-1=w3175:i32)
                          n1422 = Equal To 0?(x=w3174) -> (x = 0?=w3177:bool)
                          n1423 = Equal?(x=w3175, y=w3174) -> (x = y?=w3173:bool)
                          n1424 = call "Get_requested_rows_from_files.vi"("Last File"=w3173, "First file"=w3177, "Filename"=w3179, "Selected Rows"=w3178) -> ()  [unwired: 3 in]
                        }
                        frame "Add Inlet Temperature Offset" {
                          n1425 = for {
                            tunnel: w3188 -> [w3193] mode=indexing
                            tunnel: w3187 -> [w3192]
                            tunnel: [w3191] -> w3183 mode=indexing
                            n1426 = Index Array(array=w3192, index (row)=w3193) -> (element=w3191:string[])  [unwired: 1 in]
                          }
                          n1427 = local read "Job Directory"() -> (w3182:path)
                          n1428 = call "Get_Inlet_temps_from_files.vi"("Templated Plotted channels"=w3183, "Job Directory"=w3182, "Templated Channel Names"=w3184, "Filename"=w3185, "Selected Rows"=w3186) -> ()  [unwired: 7 in]
                        }
                        frame "Edit Values with constants" {
                          w3204 = TRUE  # Value  Constant?
                          n1429 = local read "Edit Raw Data Header Info"() -> (w3197:bool)
                          n1430 = local read "Edit Raw DF?"() -> (w3199:bool)
                          n1431 = Not(x=w3203) -> (.not. x?=w3202:bool)
                          n1432 = call "Add_Update_Values.vi"("Filename"=w3206, "Value  Constant?"=w3204, "Edit Raw data files?"=w3199, "New Chs In"=w3201, "Edit Raw Data Header Info"=w3197, "New Values In"=w3194, "Selected Rows"=w3205, "Edit all Rows?"=w3202, "Raw DF in Orig Pos?"=w3200, "Job Directory"=w3198) -> ()  [unwired: 1 in, 5 out]
                        }
                        frame "Edit values per row" {
                          w3209 = FALSE  # Edit Raw Data Header Info
                          w3221 = FALSE  # Value  Constant?
                          n1433 = for {
                            tunnel: w3218 -> [w3234] mode=indexing
                            tunnel: w3217 -> [w3233]
                            tunnel: [w3232] -> w3216 mode=indexing
                            n1434 = Search 1D Array(1D array=w3233, element=w3234) -> (index of element=w3232:i32)  [unwired: 1 out]
                          }
                          n1435 = for {
                            tunnel: w3216 -> [w3228]
                            tunnel: w3215 -> [w3227]
                            tunnel: w3214 -> [w3225] mode=indexing
                            tunnel: [w3224] -> w3213 mode=indexing
                            n1436 = Index Array(array=w3227, index (row)=w3225) -> (element=w3226:string[])  [unwired: 1 in]
                            n1437 = for {
                              tunnel: w3228 -> [w3231] mode=indexing
                              tunnel: w3226 -> [w3230]
                              tunnel: [w3229] -> w3224 mode=indexing
                              n1438 = Index Array(array=w3230, index=w3231) -> (element=w3229:string)
                            }
                          }
                          n1439 = Not(x=w3220) -> (.not. x?=w3219:bool)
                          n1440 = local read "Edit Raw DF?"() -> (w3211:bool)
                          n1441 = call "Add_Update_Values.vi"("Filename"=w3223, "Value  Constant?"=w3221, "Edit Raw data files?"=w3211, "New Chs In"=w3218, "Edit Raw Data Header Info"=w3209, "New Values In"=w3213, "Selected Rows"=w3222, "Edit all Rows?"=w3219, "Raw DF in Orig Pos?"=w3212, "Job Directory"=w3210) -> ()  [unwired: 1 in, 5 out]
                        }
                      }
                    }
                  }
                }
                frame #3 {
                  n1442 = Build Array (concatenate)(w3237, w3236) -> (w3235:i32[])
                }
              }
            }
          }
          frame #3 {
            n1443 = case shown="\"Post Process Plotted Rows\"" w3243 {
              tunnel: ["Create Selectors" "Create Selectors" w3254 "Initialise" ("t") w3288 w3294 w3301 w3307] -> w3245
              tunnel: w3244 -> [_ _ _ _ w3285 w3291 w3298 w3304]
              tunnel: w3242 -> [w3246 _ w3253 _ _ _ _ _]
              tunnel: w3241 -> [_ _ w3252 _ _ _ _ _]
              tunnel: w3240 -> [_ _ w3251 _ _ _ _ _]
              tunnel: w3239 -> [_ _ w3250 _ _ _ _ _]
              tunnel: w3238 -> [_ _ w3249 _ _ _ _ _]
              frame "Edit Raw Data file header" {
                n1444 = call "Edit_Raw_DF_Header.vi"("Selected files"=w3246) -> ()  [unwired: 15 out]
              }
              frame "Plot EnFlo Tunnel Display" {
              }
              frame "Post Process Plotted Rows" {
                n1445 = stacked-sequence {
                  seq-local: [_ w3257 _] -> [_ _ w3280]
                  tunnel: [_ _ "Create Selectors"] -> w3254
                  tunnel: w3253 -> [_ _ w3282]
                  tunnel: w3252 -> [_ _ w3281]
                  tunnel: w3251 -> [_ w3259 _]
                  tunnel: w3250 -> [_ _ w3278]
                  tunnel: w3249 -> [_ w3256 _]
                  frame #0 {
                    n1446 = local write "Post Process Plotted Data"(FALSE ("Post Process Plotted Data")) -> ()
                  }
                  frame #1 {
                    n1447 = global read "Results_plotter_Global.vi" "Precision"() -> (w3258:string[])
                    n1448 = for {
                      tunnel: w3259 -> [w3261]
                      tunnel: w3258 -> [w3264]
                      tunnel: [w3263] -> w3257 mode=indexing
                      tunnel: w3256 -> [w3262] mode=indexing
                      n1449 = Index Array(array=w3261, index (row)=w3262) -> (element=w3260:string[])  [unwired: 1 in]
                      n1450 = for {
                        tunnel: w3260 -> [w3266] mode=indexing
                        tunnel: w3264 -> [w3265] mode=indexing
                        tunnel: [w3268] -> w3263 mode=indexing
                        n1451 = Fract/Exp String To Number(string=w3266) -> (offset past number=w3272:i32, number=w3269:dbl)  [unwired: 3 out]
                        n1452 = String Length(string=w3266) -> (length=w3273:i32)
                        n1453 = Equal?(x=w3273, y=w3272) -> (x = y?=w3270:bool)
                        n1454 = Empty String/Path?(string/path=w3266) -> (empty?=w3271:bool)
                        n1455 = Compound Arithmetic op=AND(invert w3271, w3270) -> (w3267:bool)
                        n1456 = case shown="True" w3267 {
                          tunnel: w3265 -> [_ w3276]
                          tunnel: w3269 -> [_ w3277]
                          tunnel: [w3274 w3275] -> w3268
                          tunnel: w3266 -> [w3274 _]
                          frame False {
                          }
                          frame True {
                            n1457 = call "Number_2_string.vi"("precision"=w3276, "number"=w3277) -> ("String"=w3275:string)
                          }
                        }
                      }
                    }
                  }
                  frame #2 {
                    n1458 = Build Array (concatenate)(w3278, w3280) -> (w3279:string[][])
                    n1459 = call "Post_Process_Profile_Remote.vi"("Results Plotter Rows"=w3279, "Raw Data files to PP"=w3282, "Current Results filenames"=w3281) -> ()  [unwired: 1 out]
                  }
                }
              }
              frame "Delete unwanted rows" {
              }
              frame "Edit Values with constants" {
                n1460 = local read "nRows"() -> (w3287:i32)
                n1461 = Less?(x=w3287, y=w3285) -> (x < y?=w3286:bool)
                n1462 = case shown="True" w3286 {
                  tunnel: ["Create Selectors" "Initialise" ("t")] -> w3288
                  frame False {
                  }
                  frame True {
                  }
                }
              }
              frame "Edit values per row" {
                n1463 = local read "nRows"() -> (w3293:i32)
                n1464 = Less?(x=w3293, y=w3291) -> (x < y?=w3292:bool)
                n1465 = case shown="True" w3292 {
                  tunnel: ["Create Selectors" "Initialise" ("t")] -> w3294
                  frame False {
                  }
                  frame True {
                  }
                }
              }
              frame "Add Inlet Temperature Offset" {
                n1466 = local read "nRows"() -> (w3300:i32)
                n1467 = Less?(x=w3300, y=w3298) -> (x < y?=w3299:bool)
                n1468 = case shown="True" w3299 {
                  tunnel: ["Create Selectors" "Initialise" ("t")] -> w3301
                  frame False {
                  }
                  frame True {
                  }
                }
                n1469 = local write "Add Inlet Temperature offset"(FALSE ("Add Inlet Temperature offset")) -> ()
              }
              frame "Save file" {
                n1470 = local read "nRows"() -> (w3306:i32)
                n1471 = Less?(x=w3306, y=w3304) -> (x < y?=w3305:bool)
                n1472 = case shown="True" w3305 {
                  tunnel: ["Create Selectors" "Initialise" ("t")] -> w3307
                  frame False {
                  }
                  frame True {
                  }
                }
              }
            }
          }
          frame #4 {
            n1473 = Current VI's Path() -> (path=w3310:path)
            n1474 = call "Bring_to_front.vi"("path"=w3310) -> ()
          }
        }
      }
      frame "End" {
        n1475 = local read "Template"() -> (w3313:path)
        n1476 = local read "Empty"() -> (w3314:bool)
        n1477 = call "Valid_Path.vi"("Filename"=w3313) -> ("Valid Path?"=w3312:bool)
        n1478 = case shown="True" w3314 {
          frame False {
          }
          frame True {
            n1479 = property on="Result files to read" class="Arr (strict)"("Index Values"=u32[] [0] ("Write Attribute")) -> ()  [unwired: 2 in, 2 out]
            n1480 = local write "Result files to read"(path[] [] ("Result files to read")) -> ()
            n1481 = local write "Empty"(FALSE ("Empty")) -> ()
          }
        }
        n1482 = case shown="False" w3312 {
          tunnel: w3315 -> [w3324 _]
          frame False {
            n1483 = local write "Template"(w3324) -> ()
          }
          frame True {
          }
        }
        n1484 = global write "Results_plotter_Global.vi" "Plot EnFlo Tunnel Display"(FALSE ("Plot EnFlo Tunnel Display")) -> ()
      }
      frame "Empty Results file array" {
        n1485 = local read "Template"() -> (w3326:path)
        n1486 = call "Valid_Path.vi"("Filename"=w3326) -> ("Valid Path?"=w3325:bool)
        n1487 = case shown="False" w3325 {
          tunnel: w3327 -> [w3336 _]
          frame False {
            n1488 = local write "Template"(w3336) -> ()
          }
          frame True {
          }
        }
        n1489 = property on="Result files to read" class="Arr (strict)"("Index Values"=u32[] [0] ("Write Attribute")) -> ()  [unwired: 2 in, 2 out]
        n1490 = local write "Result files to read"(path[] [] ("Result files to read")) -> ()
        n1491 = local write "Empty"(FALSE ("Empty")) -> ()
      }
      frame "Save Setup" {
        n1492 = local read "Create picture Vi Name"() -> (w3360:string)
        n1493 = local read "Additional X Values"() -> (w3366:dbl[])
        n1494 = local read "Additional Y Values"() -> (w3365:dbl[])
        n1495 = local read "Result files to read"() -> (w3368:path[])
        n1496 = local read "Output Filename"() -> (w3361:path)
        n1497 = local read "Multi Ordinate?"() -> (w3358:bool)
        n1498 = local read "Intensity Plot?"() -> (w3359:bool)
        n1499 = local read "Multi Ordinate"() -> (w3354:i32[])
        n1500 = local read "Filter Array"() -> (w3362:u16[])
        n1501 = local read "Transpose"() -> (w3367:bool)
        n1502 = local read "Template"() -> (w3349:path)
        n1503 = local read "Ordinate"() -> (w3364:u16)
        n1504 = local read "Filter Bins 2"() -> (w3355:i32[])
        n1505 = local read "Filter Bins 1"() -> (w3356:i32[])
        n1506 = local read "Absisca"() -> (w3363:u16)
        n1507 = global read "Trav_pos_global.vi" "Estimated Completion time"() -> (w3345:string)
        n1508 = call "Read_Write_Plot_Setup.vi"("Mode"=enum16{"Load", "Save"}."Load", "Setup filename"=w3339) -> ("Cluster 2"=w3369:T10)  [unwired: 1 in, 1 out]
        n1509 = Bundle By Name(cluster=w3369, "Result files to read"=w3368, "Template"=w3349, "Transpose"=w3367, "Additional X Values"=w3366, "Additional Y Values"=w3365, "Ordinate"=w3364, "Absisca"=w3363, "Filter Array"=w3362, "color and symbol"=TRUE, "Output Filename"=w3361, "Jpg Vi Name"=w3360, "Intensity Plot?"=w3359, "Multi Ordinate?"=w3358, "Filter Bins 1"=w3356, "Filter Bins 2"=w3355, "Multi Ordinate"=w3354) -> (w3357:T10)
        n1510 = local read "stop"() -> (w3352:bool)
        n1511 = Empty String/Path?(string/path=w3345) -> (empty?=w3344:bool)
        n1512 = Not(x=w3352) -> (.not. x?=w3343:bool)
        n1513 = local read "Save Setup"() -> (w3341:bool)
        n1514 = And(x=w3343, y=w3344) -> (x .and. y?=w3342:bool)
        n1515 = call "Path_2_String.vi"("Real Path"="Job Directory") -> ("Path String"=w3337:string)
        n1516 = call "Read_Write_Plot_Setup.vi"("Mode"=enum16{"Load", "Save"}."Save", "Setup filename"=w3339, "Cluster"=w3357) -> ()  [unwired: 2 out]
        n1517 = Or(x=w3341, y=w3342) -> (x .or. y?=w3340:bool)
        n1518 = call "Read_Write_Template.vi"("Template File"=w3349, "Mode"=Global_mode."Write Global to File", "Single Value In"=w3337, "Data type"="Log Folder Name" ("Variable name")) -> ()  [unwired: 4 in, 8 out]
        n1519 = Select(t="Save to named setup file", s=w3341, f="Check modification dates?") -> (s? t:f=w3347:string)
      }
      frame "Save to named setup file" {
        w3376 = TRUE  # Save New File?
        n1520 = call "Save_current_setup.vi"("Save New File?"=w3376, "Setup File Type"=Setup_Filetype."Results File Plotter Setups") -> ()  [unwired: 4 out]
        n1521 = local write "Save Setup"(FALSE ("Save Setup")) -> ()
      }
    }
    n1522 = Wait (ms)(milliseconds to wait=u32 50) -> ()  [unwired: 1 out]
    "Current" <- w20
  }
